vi "Beampointing_Multi_Pico2_test.vi"() -> ()   [LabVIEW 2011]
uses:
  GUI_Template/GUI_master/tcp_new_data_event.ctl
  GUI_Template/GUI_master/tcp new data cluster.ctl
  Ctrs/beam detection.ctl
  GUI_Beampointing_single_TRA/Ctrs/move.ctl
  <vilib>/Utility/file.llb/Read From Spreadsheet File (string).vi
  <userlib>/_OpenG.lib/array/array.llb/Filter 1D Array with Scalar (String)__ogtk.vi
  <userlib>/_OpenG.lib/array/array.llb/Filter 1D Array (String)__ogtk.vi
  <vilib>/Utility/file.llb/Write To Spreadsheet File (string).vi
  <vilib>/Analysis/NI_AALBase.lvlib
panel:
  out "x-y*floor(x/y)":dbl
  out "error out":errorcluster
  out "config path":string
  out "Array 3":bool[](array[boolean])
  out "Array 2":u16[](array[numeric])
  out "Array":u16[](array[numeric])
  out "Moving Y":string
  out "Moving X":string
  out "particles":T1(array[cluster])
  out "millisecond timer value":u32
  out "appended path":path
  out "millisecond timer 2":u32
  in  "GUIdevice 98":string="PicoPad4"
  in  "Position.Axis 111::98":dbl=77.0 caption="Motor Axis 1" min=-20000.0 max=20000.0 format="%#_6f"
  in  "Position.Axis 112::98":dbl=77.0 caption="Motor Axis 1" min=-20000.0 max=20000.0 format="%#_6f"
  in  "Position.Axis 113::98":dbl=77.0 caption="Motor Axis 1" min=-20000.0 max=20000.0 format="%#_6f"
  in  "Position.Axis 121::98":dbl=77.0 caption="Motor Axis 1" min=-999999.0 max=999999.0 format="%#_6f"
  in  "Position.Axis 122::98":dbl=77.0 caption="Motor Axis 1" min=-999999.0 max=999999.0 format="%#_6f"
  in  "Position.Axis 123::98":dbl=77.0 caption="Motor Axis 1" min=-999999.0 max=999999.0 format="%#_6f"
  in  "Position.Axis 131::98":dbl=77.0 caption="Motor Axis 1" min=-999999.0 max=999999.0 format="%#_6f"
  in  "Position.Axis 132::98":dbl=77.0 caption="Motor Axis 1" min=-999999.0 max=999999.0 format="%#_6f"
  in  "Position.Axis 133::98":dbl=77.0 caption="Motor Axis 1" min=-999999.0 max=999999.0 format="%#_6f"
  in  "Position.Axis 141::98":dbl=77.0 caption="Motor Axis 1" min=-999999.0 max=999999.0 format="%#_6f"
  in  "Position.Axis 142::98":dbl=77.0 caption="Motor Axis 1" min=-999999.0 max=999999.0 format="%#_6f"
  in  "Position.Axis 143::98":dbl=77.0 caption="Motor Axis 1" min=-999999.0 max=999999.0 format="%#_6f"
  in  "Position.Axis 211::98":dbl=77.0 caption="Motor Axis 1" min=-999999.0 max=999999.0 format="%#_6f"
  in  "Position.Axis 212::98":dbl=77.0 caption="Motor Axis 1" min=-999999.0 max=999999.0 format="%#_6f"
  in  "Position.Axis 213::98":dbl=77.0 caption="Motor Axis 1" min=-999999.0 max=999999.0 format="%#_6f"
  in  "Position.Axis 221::98":dbl=77.0 caption="Motor Axis 1" min=-999999.0 max=999999.0 format="%#_6f"
  in  "Position.Axis 222::98":dbl=77.0 caption="Motor Axis 1" min=-999999.0 max=999999.0 format="%#_6f"
  in  "Position.Axis 223::98":dbl=77.0 caption="Motor Axis 1" min=-999999.0 max=999999.0 format="%#_6f"
  in  "Position.Axis 231::98":dbl=77.0 caption="Motor Axis 1" min=-999999.0 max=999999.0 format="%#_6f"
  in  "Position.Axis 232::98":dbl=77.0 caption="Motor Axis 1" min=-999999.0 max=999999.0 format="%#_6f"
  in  "Position.Axis 233::98":dbl=77.0 caption="Motor Axis 1" min=-999999.0 max=999999.0 format="%#_6f"
  in  "Position.Axis 241::98":dbl=77.0 caption="Motor Axis 1" min=-999999.0 max=999999.0 format="%#_6f"
  in  "Position.Axis 242::98":dbl=77.0 caption="Motor Axis 1" min=-999999.0 max=999999.0 format="%#_6f"
  in  "Position.Axis 243::98":dbl=77.0 caption="Motor Axis 1" min=-999999.0 max=999999.0 format="%#_6f"
  in  "Position.Axis 311::98":dbl=77.0 caption="Motor Axis 1" min=-999999.0 max=999999.0 format="%#_6f"
  in  "Position.Axis 312::98":dbl=77.0 caption="Motor Axis 1" min=-999999.0 max=999999.0 format="%#_6f"
  in  "Position.Axis 313::98":dbl=77.0 caption="Motor Axis 1" min=-999999.0 max=999999.0 format="%#_6f"
  in  "Position.Axis 321::98":dbl=77.0 caption="Motor Axis 1" min=-999999.0 max=999999.0 format="%#_6f"
  in  "Position.Axis 322::98":dbl=77.0 caption="Motor Axis 1" min=-999999.0 max=999999.0 format="%#_6f"
  in  "Position.Axis 323::98":dbl=77.0 caption="Motor Axis 1" min=-999999.0 max=999999.0 format="%#_6f"
  in  "Position.Axis 331::98":dbl=77.0 caption="Motor Axis 1" min=-999999.0 max=999999.0 format="%#_6f"
  in  "Position.Axis 332::98":dbl=77.0 caption="Motor Axis 1" min=-999999.0 max=999999.0 format="%#_6f"
  in  "Position.Axis 333::98":dbl=77.0 caption="Motor Axis 1" min=-999999.0 max=999999.0 format="%#_6f"
  in  "Position.Axis 341::98":dbl=77.0 caption="Motor Axis 1" min=-999999.0 max=999999.0 format="%#_6f"
  in  "Position.Axis 342::98":dbl=77.0 caption="Motor Axis 1" min=-999999.0 max=999999.0 format="%#_6f"
  in  "Position.Axis 343::98":dbl=77.0 caption="Motor Axis 1" min=-999999.0 max=999999.0 format="%#_6f"
  in  "Position.Axis 411::98":dbl=77.0 caption="Motor Axis 1" min=-999999.0 max=999999.0 format="%#_6f"
  in  "Position.Axis 412::98":dbl=77.0 caption="Motor Axis 1" min=-999999.0 max=999999.0 format="%#_6f"
  in  "Position.Axis 413::98":dbl=77.0 caption="Motor Axis 1" min=-999999.0 max=999999.0 format="%#_6f"
  in  "Position.Axis 421::98":dbl=77.0 caption="Motor Axis 1" min=-999999.0 max=999999.0 format="%#_6f"
  in  "Position.Axis 422::98":dbl=77.0 caption="Motor Axis 1" min=-999999.0 max=999999.0 format="%#_6f"
  in  "Position.Axis 423::98":dbl=77.0 caption="Motor Axis 1" min=-999999.0 max=999999.0 format="%#_6f"
  in  "Position.Axis 431::98":dbl=77.0 caption="Motor Axis 1" min=-999999.0 max=999999.0 format="%#_6f"
  in  "Position.Axis 432::98":dbl=77.0 caption="Motor Axis 1" min=-999999.0 max=999999.0 format="%#_6f"
  in  "Position.Axis 433::98":dbl=77.0 caption="Motor Axis 1" min=-999999.0 max=999999.0 format="%#_6f"
  in  "Position.Axis 441::98":dbl=77.0 caption="Motor Axis 1" min=-999999.0 max=999999.0 format="%#_6f"
  in  "Position.Axis 442::98":dbl=77.0 caption="Motor Axis 1" min=-999999.0 max=999999.0 format="%#_6f"
  in  "Position.Axis 443::98":dbl=77.0 caption="Motor Axis 1" min=-999999.0 max=999999.0 format="%#_6f"
  in  "Position.Axis 511::98":dbl=77.0 caption="Motor Axis 1" min=-999999.0 max=999999.0 format="%#_6f"
  in  "Position.Axis 512::98":dbl=77.0 caption="Motor Axis 1" min=-999999.0 max=999999.0 format="%#_6f"
  in  "Position.Axis 513::98":dbl=77.0 caption="Motor Axis 1" min=-999999.0 max=999999.0 format="%#_6f"
  in  "Position.Axis 521::98":dbl=77.0 caption="Motor Axis 1" min=-999999.0 max=999999.0 format="%#_6f"
  in  "Position.Axis 522::98":dbl=77.0 caption="Motor Axis 1" min=-999999.0 max=999999.0 format="%#_6f"
  in  "Position.Axis 523::98":dbl=77.0 caption="Motor Axis 1" min=-999999.0 max=999999.0 format="%#_6f"
  in  "Position.Axis 531::98":dbl=77.0 caption="Motor Axis 1" min=-999999.0 max=999999.0 format="%#_6f"
  in  "Position.Axis 532::98":dbl=77.0 caption="Motor Axis 1" min=-999999.0 max=999999.0 format="%#_6f"
  in  "Position.Axis 533::98":dbl=77.0 caption="Motor Axis 1" min=-999999.0 max=999999.0 format="%#_6f"
  in  "Position.Axis 541::98":dbl=77.0 caption="Motor Axis 1" min=-999999.0 max=999999.0 format="%#_6f"
  in  "Position.Axis 542::98":dbl=77.0 caption="Motor Axis 1" min=-999999.0 max=999999.0 format="%#_6f"
  in  "Position.Axis 543::98":dbl=77.0 caption="Motor Axis 1" min=-999999.0 max=999999.0 format="%#_6f"
  in  "Numeric":dbl
  out "Current State":string
  in  "output cluster 2":T5 {"detection para"."smal para"."Measurement Parameter" items=["Center of Mass X", "Center of Mass Y", "First Pixel X", "First Pixel Y", "Bounding Rect Left", "Bounding Rect Top", "Bounding Rect Right", "Bounding Rect Bottom", "Max Feret Diameter Start X", "Max Feret Diameter Start Y", "Max Feret Diameter End X", "Max Feret Diameter End Y", "Max Horiz. Segment Length Left", "Max Horiz. Segment Length Right", "Max Horiz. Segment Length Row", "-", "Bounding Rect Width", "Bounding Rect Height", "Bounding Rect Diagonal", "Perimeter", "Convex Hull Perimeter", "Holes' Perimeter", "Max Feret Diameter", "Equivalent Ellipse Major Axis", "Equivalent Ellipse Minor Axis", "Equivalent Ellipse Minor Axis (Feret)", "Equivalent Rect Long Side", "Equivalent Rect Short Side", "Equivalent Rect Diagonal", "Equivalent Rect Short Side (Feret)", "Average Horiz. Segment Length", "Average Vert. Segment Length", "Hydraulic Radius", "Waddel Disk Diameter", "-", "Area", "Holes' Area", "Particle & Holes' Area", "Convex Hull Area", "Image Area", "-", "Number of Holes", "Number of Horiz. Segments", "Number of Vert. Segments", "-", "Orientation", "Max Feret Diameter Orientation", "-", "% Area/Image Area", "% Area/(Particle & Holes' Area)", "Ratio of Equivalent Ellipse Axes", "Ratio of Equivalent Rect Sides", "-", "Elongation Factor", "Compactness Factor", "Heywood Circularity Factor", "Type Factor", "-", "Sum X", "Sum Y", "Sum XX", "Sum XY", "Sum YY", "Sum XXX", "Sum XXY", "Sum XYY", "Sum YYY", "-", "Moment of Inertia XX", "Moment of Inertia XY", "Moment of Inertia YY", "Moment of Inertia XXX", "Moment of Inertia XXY", "Moment of Inertia XYY", "Moment of Inertia YYY", "Norm. Moment of Inertia XX", "Norm. Moment of Inertia XY", "Norm. Moment of Inertia YY", "Norm. Moment of Inertia XXX", "Norm. Moment of Inertia XXY", "Norm. Moment of Inertia XYY", "Norm. Moment of Inertia YYY", "Hu Moment 1", "Hu Moment 2", "Hu Moment 3", "Hu Moment 4", "Hu Moment 5", "Hu Moment 6", "Hu Moment 7"]; "detection para"."smal para"."Range Lower Value" format="%.2f"; "detection para"."smal para"."Range Upper Value" format="%.2f"; "detection para"."detection method" items=["clustering", "entropy", "metric", "moments", "inter-class variance"]; "detection para"."Filter" items=["No Filter", "Median Filter", "Low Pass Filter"]}
  out "CCDs":string[](array[string])
  in  "GUIdevice 12":string
  in  "GUIdevice 11":string
  in  "GUIdevice 10":string
  in  "GUIdevice 9":string
  out "error out 2":errorcluster
  in  "active cams":string[](array[string])
  in  "Motor Y":dbl[][](array[numeric])
  in  "Motor X":dbl[][](array[numeric])
  out "Names":string[](array[string])
  in  "Offset X stats":dbl[][](array[numeric])
  in  "Offset Y stats":dbl[][](array[numeric])
  out "Box":T6(array[cluster])
  in  "Tab Control 2":enum32{"Config ", "Main", "History"}(tab)=enum."Main"
  out "Waveform Chart":u32(graph)
  in  "associated motors":T7
  out "Cameras":T8
  out "Status":cluster{i32, i32, "Centroid X":dbl[][]}(graph)
  in  "Exposure:12":dbl=0.095 min=0.0001 max=1.0 format="%#_6f"
  in  "Triggerdelay::12":dbl=0.003 min=0.0 max=0.09 format="%#_6f"
  in  "Exposure::11":dbl=0.095 min=0.0001 max=1.0 format="%#_6f"
  in  "Triggerdelay::11":dbl=0.003 min=0.0 max=0.09 format="%#_6f"
  in  "Exposure::10":dbl=0.095 min=0.0001 max=1.0 format="%#_6f"
  in  "Triggerdelay::10":dbl=0.003 min=0.0 max=0.09 format="%#_6f"
  in  "Exposure::9":dbl=0.095 min=0.0001 max=1.0 format="%#_6f"
  in  "Triggerdelay::9":dbl=0.003 min=0.0 max=0.09 format="%#_6f"
  in  "Trigger::9":bool
  in  "Trigger::10":bool caption="Trigger:10"
  in  "Trigger::11":bool
  in  "Trigger::12":bool
  in  "Target.Y::9":dbl=45.0 caption="T9y" min=0.0 max=2000.0 format="%#_6f"
  in  "Target.X::9":dbl=47.0 caption="Tx9" min=0.0 max=2000.0 format="%#_6f"
  in  "Target.Y::10":dbl=45.0 caption="T10y" min=0.0 max=2000.0 format="%#_6f"
  in  "Target.X::10":dbl=47.0 caption="T10x" min=0.0 max=2000.0 format="%#_6f"
  in  "Target.Y::11":dbl=45.0 caption="T11y" min=0.0 max=2000.0 format="%#_6f"
  in  "Target.X::11":dbl=47.0 caption="T11x" min=0.0 max=2000.0 format="%#_6f"
  in  "Target.Y::12":dbl=45.0 caption="T12y" min=0.0 max=2000.0 format="%#_6f"
  in  "Target.X::12":dbl=47.0 caption="T12x" min=0.0 max=2000.0 format="%#_6f"
  in  "Exposure::8":dbl=0.095 min=0.01 max=1.0 format="%#_6f"
  in  "Triggerdelay::8":dbl=0.003 min=0.0 max=0.09 format="%#_6f"
  in  "Trigger::8":bool
  in  "Target.Y::8":dbl=45.0 caption="T8y" min=0.0 max=2000.0 format="%#_6f"
  in  "Target.X::8":dbl=47.0 caption="T8x" min=0.0 max=2000.0 format="%#_6f"
  in  "Target.Y::7":dbl=45.0 caption="T7x" min=0.0 max=2000.0 format="%#_6f"
  in  "Target.X::7":dbl=47.0 caption="T7y" min=0.0 max=2000.0 format="%#_6f"
  in  "Target.Y::6":dbl=45.0 caption="T6y" min=0.0 max=2000.0 format="%#_6f"
  in  "Target.X::6":dbl=47.0 caption="T6x" min=0.0 max=2000.0 format="%#_6f"
  in  "Target.Y::5":dbl=45.0 caption="T5y" min=0.0 max=2000.0 format="%#_6f"
  in  "Target.X::5":dbl=47.0 caption="T5x" min=0.0 max=2000.0 format="%#_6f"
  in  "Target.Y::4":dbl=45.0 caption="T4y" min=0.0 max=2000.0 format="%#_6f"
  in  "Target.X::4":dbl=47.0 caption="T4x" min=0.0 max=2000.0 format="%#_6f"
  in  "Target.Y::3":dbl=163.0 caption="T3y" min=0.0 max=2000.0 format="%#_6f"
  in  "Target.X::3":dbl=152.0 caption="T3x" min=0.0 max=2000.0 format="%#_6f"
  in  "Target.Y::2":dbl=74.0 caption="T2y" min=1.0 max=600.0 format="%#_6f"
  in  "Target.X::2":dbl=75.0 caption="T2x" min=1.0 max=800.0 format="%#_6f"
  in  "Target.Y::1":dbl=61.0 caption="T1y" min=1.0 max=600.0 format="%#_6f"
  in  "Target.X::1":dbl=77.0 caption="T1x" min=1.0 max=800.0 format="%#_6f"
  in  "Exposure::7":dbl=0.095 min=0.0001 max=1.0 format="%#_6f"
  in  "Triggerdelay::7":dbl=0.003 min=0.0 max=0.09 format="%#_6f"
  in  "Trigger::7":bool
  in  "Exposure::6":dbl=0.095 min=0.0001 max=1.0 format="%#_6f"
  in  "Triggerdelay::6":dbl=0.003 min=0.0 max=0.09 format="%#_6f"
  in  "Trigger::6":bool
  in  "Exposure::5":dbl=0.095 min=0.0001 max=1.0 format="%#_6f"
  in  "Triggerdelay::5":dbl=0.003 min=0.0 max=0.09 format="%#_6f"
  in  "Trigger::5":bool
  in  "Exposure::4":dbl=0.095 min=0.0001 max=1.0 format="%#_6f"
  in  "Triggerdelay::4":dbl=0.003 min=0.0 max=0.09 format="%#_6f"
  in  "Trigger::4":bool
  in  "Exposure::3":dbl=0.095 min=0.0001 max=1.0 format="%#_6f"
  in  "Triggerdelay::3":dbl=0.003 min=0.0 max=0.09 format="%#_6f"
  in  "Trigger::3":bool
  in  "Exposure::2":dbl=0.095 min=0.0001 max=1.0 format="%#_6f"
  in  "Triggerdelay::2":dbl=0.003 min=0.0 max=0.09 format="%#_6f"
  in  "Trigger::2":bool
  out "image::1":T9(plugin-control) caption="PA2_Input1"
  out "image::2":T9(plugin-control) caption="PA2_Input2"
  out "image::3":T9(plugin-control) caption="L1_TelInpNear"
  out "image::4":T9(plugin-control) caption="L2_TelInpFar"
  out "image::5":T9(plugin-control) caption="L4_TREXpass1"
  out "image::6":T9(plugin-control) caption="L5_TREXPass2"
  out "image::7":T9(plugin-control) caption="L6_TREXpass3"
  out "image::8":T9(plugin-control) caption="L7_TREXPass4"
  in  "Exposure::1":dbl=0.095 min=0.0001 max=1.0 format="%#_6f"
  in  "Triggerdelay::1":dbl=0.003 min=0.0 max=0.09 format="%#_6f"
  in  "Trigger::1":bool
  in  "UDP error message":string
  out "required Y":bool[](array[boolean])
  out "required X":bool[](array[boolean])
  out "detected":bool[](array[boolean])
  out "name array":string[](array[string])
  out "image::9":T9(plugin-control) caption="L8_M10Leak"
  out "image::10":T9(plugin-control) caption="B1_TelInput"
  out "image::11":T9(plugin-control) caption="B2_TelLens1"
  out "image::12":T9(plugin-control) caption="B5_CompressorOut"
  out "speedmode X":bool[](array[boolean])
  out "speedmode Y":bool[](array[boolean])
  out "CCD 9":cluster{timestamp[], dbl[]}[](graph)
  out "CCD 10":cluster{timestamp[], dbl[]}[](graph)
  out "CCD 11":cluster{timestamp[], dbl[]}[](graph)
  out "CCD 12":cluster{timestamp[], dbl[]}[](graph)
  out "CCD 5":cluster{timestamp[], dbl[]}[](graph)
  out "CCD 6":cluster{timestamp[], dbl[]}[](graph)
  out "CCD 7":cluster{timestamp[], dbl[]}[](graph)
  out "CCD 8":cluster{timestamp[], dbl[]}[](graph)
  out "CCD 2":cluster{timestamp[], dbl[]}[](graph)
  out "CCD 1":cluster{timestamp[], dbl[]}[](graph)
  out "CCD 3":cluster{timestamp[], dbl[]}[](graph)
  out "CCD 4":cluster{timestamp[], dbl[]}[](graph)
  out "History index":i32
  in  "History Size":i32=500
  out "Particle Reports (Pixels)":T10(array[cluster])
  in  "Feedback Global":bool
  in  "detection para":T3[](array[typedef])=[{"Filter"=1, "Filter Para"={"X Size"=5, "Y Size"=5, "% Tolerance"=1}, "detection method"=4, "smal para"=[{"Measurement Parameter"=35, "Range Lower Value"=0.0, "Range Upper Value"=0.0, "Range"=TRUE, "Measurement Type"=FALSE}], "Remove small Objects"=TRUE, "Restrict to round Objects"=FALSE}, {"Filter"=1, "Filter Para"={"X Size"=5, "Y Size"=5, "% Tolerance"=1}, "detection method"=4, "smal para"=[{"Measurement Parameter"=35, "Range Lower Value"=0.0, "Range Upper Value"=500.0, "Range"=FALSE, "Measurement Type"=FALSE}], "Remove small Objects"=TRUE, "Restrict to round Objects"=FALSE}, {"Filter"=1, "Filter Para"={"X Size"=5, "Y Size"=5, "% Tolerance"=1}, "detection method"=4, "smal para"=[{"Measurement Parameter"=35, "Range Lower Value"=0.0, "Range Upper Value"=500.0, "Range"=TRUE, "Measurement Type"=FALSE}], "Remove small Objects"=TRUE, "Restrict to round Objects"=FALSE}, {"Filter"=1, "Filter Para"={"X Size"=5, "Y Size"=5, "% Tolerance"=1}, "detection method"=4, "smal para"=[{"Measurement Parameter"=35, "Range Lower Value"=0.0, "Range Upper Value"=500.0, "Range"=TRUE, "Measurement Type"=FALSE}], "Remove small Objects"=TRUE, "Restrict to round Objects"=FALSE}, {"Filter"=1, "Filter Para"={"X Size"=5, "Y Size"=5, "% Tolerance"=1}, "detection method"=4, "smal para"=[{"Measurement Parameter"=35, "Range Lower Value"=0.0, "Range Upper Value"=500.0, "Range"=TRUE, "Measurement Type"=FALSE}], "Remove small Objects"=TRUE, "Restrict to round Objects"=FALSE}, {"Filter"=1, "Filter Para"={"X Size"=5, "Y Size"=5, "% Tolerance"=1}, "detection method"=4, "smal para"=[{"Measurement Parameter"=35, "Range Lower Value"=0.0, "Range Upper Value"=500.0, "Range"=TRUE, "Measurement Type"=FALSE}], "Remove small Objects"=TRUE, "Restrict to round Objects"=FALSE}, {"Filter"=1, "Filter Para"={"X Size"=5, "Y Size"=5, "% Tolerance"=1}, "detection method"=4, "smal para"=[{"Measurement Parameter"=35, "Range Lower Value"=0.0, "Range Upper Value"=500.0, "Range"=TRUE, "Measurement Type"=FALSE}], "Remove small Objects"=TRUE, "Restrict to round Objects"=FALSE}, {"Filter"=1, "Filter Para"={"X Size"=5, "Y Size"=5, "% Tolerance"=1}, "detection method"=3, "smal para"=[{"Measurement Parameter"=35, "Range Lower Value"=0.0, "Range Upper Value"=0.0, "Range"=FALSE, "Measurement Type"=FALSE}], "Remove small Objects"=TRUE, "Restrict to round Objects"=FALSE}, {"Filter"=1, "Filter Para"={"X Size"=5, "Y Size"=5, "% Tolerance"=1}, "detection method"=4, "smal para"=[{"Measurement Parameter"=35, "Range Lower Value"=0.0, "Range Upper Value"=0.0, "Range"=FALSE, "Measurement Type"=FALSE}], "Remove small Objects"=TRUE, "Restrict to round Objects"=FALSE}, {"Filter"=1, "Filter Para"={"X Size"=5, "Y Size"=5, "% Tolerance"=1}, "detection method"=4, "smal para"=[{"Measurement Parameter"=35, "Range Lower Value"=0.0, "Range Upper Value"=500.0, "Range"=TRUE, "Measurement Type"=FALSE}], "Remove small Objects"=TRUE, "Restrict to round Objects"=FALSE}, {"Filter"=1, "Filter Para"={"X Size"=5, "Y Size"=5, "% Tolerance"=1}, "detection method"=4, "smal para"=[{"Measurement Parameter"=35, "Range Lower Value"=0.0, "Range Upper Value"=500.0, "Range"=TRUE, "Measurement Type"=FALSE}], "Remove small Objects"=TRUE, "Restrict to round Objects"=FALSE}, {"Filter"=1, "Filter Para"={"X Size"=5, "Y Size"=5, "% Tolerance"=1}, "detection method"=4, "smal para"=[{"Measurement Parameter"=35, "Range Lower Value"=0.0, "Range Upper Value"=500.0, "Range"=TRUE, "Measurement Type"=FALSE}], "Remove small Objects"=TRUE, "Restrict to round Objects"=FALSE}] {"smal para"."Measurement Parameter" items=["Center of Mass X", "Center of Mass Y", "First Pixel X", "First Pixel Y", "Bounding Rect Left", "Bounding Rect Top", "Bounding Rect Right", "Bounding Rect Bottom", "Max Feret Diameter Start X", "Max Feret Diameter Start Y", "Max Feret Diameter End X", "Max Feret Diameter End Y", "Max Horiz. Segment Length Left", "Max Horiz. Segment Length Right", "Max Horiz. Segment Length Row", "-", "Bounding Rect Width", "Bounding Rect Height", "Bounding Rect Diagonal", "Perimeter", "Convex Hull Perimeter", "Holes' Perimeter", "Max Feret Diameter", "Equivalent Ellipse Major Axis", "Equivalent Ellipse Minor Axis", "Equivalent Ellipse Minor Axis (Feret)", "Equivalent Rect Long Side", "Equivalent Rect Short Side", "Equivalent Rect Diagonal", "Equivalent Rect Short Side (Feret)", "Average Horiz. Segment Length", "Average Vert. Segment Length", "Hydraulic Radius", "Waddel Disk Diameter", "-", "Area", "Holes' Area", "Particle & Holes' Area", "Convex Hull Area", "Image Area", "-", "Number of Holes", "Number of Horiz. Segments", "Number of Vert. Segments", "-", "Orientation", "Max Feret Diameter Orientation", "-", "% Area/Image Area", "% Area/(Particle & Holes' Area)", "Ratio of Equivalent Ellipse Axes", "Ratio of Equivalent Rect Sides", "-", "Elongation Factor", "Compactness Factor", "Heywood Circularity Factor", "Type Factor", "-", "Sum X", "Sum Y", "Sum XX", "Sum XY", "Sum YY", "Sum XXX", "Sum XXY", "Sum XYY", "Sum YYY", "-", "Moment of Inertia XX", "Moment of Inertia XY", "Moment of Inertia YY", "Moment of Inertia XXX", "Moment of Inertia XXY", "Moment of Inertia XYY", "Moment of Inertia YYY", "Norm. Moment of Inertia XX", "Norm. Moment of Inertia XY", "Norm. Moment of Inertia YY", "Norm. Moment of Inertia XXX", "Norm. Moment of Inertia XXY", "Norm. Moment of Inertia XYY", "Norm. Moment of Inertia YYY", "Hu Moment 1", "Hu Moment 2", "Hu Moment 3", "Hu Moment 4", "Hu Moment 5", "Hu Moment 6", "Hu Moment 7"]; "smal para"."Range Lower Value" format="%.2f"; "smal para"."Range Upper Value" format="%.2f"; "detection method" items=["clustering", "entropy", "metric", "moments", "inter-class variance"]; "Filter" items=["No Filter", "Median Filter", "Low Pass Filter"]}
  in  "GUIdevice 8":string="B5_CompressorOut"
  in  "Tab Control":T11(tab)
  in  "Center":bool
  in  "Save Stats":bool
  in  "Save Config":bool
  in  "Load Config":bool
  in  "update speed [ms]":i32=200
  in  "Img to avg":i32=20
  in  "Reset History":bool
  in  "save path":path=path "W:/BP_DATA"
  in  "autodetect":bool
  in  "Detection Rate":dbl=0.8 min=0.001 max=1.0
  in  "new tdms":bool
  in  "Speedmode @":dbl=3.0 min=1.0 max=20.0
  in  "Align":bool
  in  "deivice ini":bool
  in  "beam detection para":T3={"Filter"=1, "Filter Para"={"X Size"=5, "Y Size"=5, "% Tolerance"=1}, "detection method"=4, "smal para"=[{"Measurement Parameter"=35, "Range Lower Value"=0.0, "Range Upper Value"=500.0, "Range"=FALSE, "Measurement Type"=FALSE}], "Remove small Objects"=TRUE, "Restrict to round Objects"=FALSE} {"smal para"."Measurement Parameter" items=["Center of Mass X", "Center of Mass Y", "First Pixel X", "First Pixel Y", "Bounding Rect Left", "Bounding Rect Top", "Bounding Rect Right", "Bounding Rect Bottom", "Max Feret Diameter Start X", "Max Feret Diameter Start Y", "Max Feret Diameter End X", "Max Feret Diameter End Y", "Max Horiz. Segment Length Left", "Max Horiz. Segment Length Right", "Max Horiz. Segment Length Row", "-", "Bounding Rect Width", "Bounding Rect Height", "Bounding Rect Diagonal", "Perimeter", "Convex Hull Perimeter", "Holes' Perimeter", "Max Feret Diameter", "Equivalent Ellipse Major Axis", "Equivalent Ellipse Minor Axis", "Equivalent Ellipse Minor Axis (Feret)", "Equivalent Rect Long Side", "Equivalent Rect Short Side", "Equivalent Rect Diagonal", "Equivalent Rect Short Side (Feret)", "Average Horiz. Segment Length", "Average Vert. Segment Length", "Hydraulic Radius", "Waddel Disk Diameter", "-", "Area", "Holes' Area", "Particle & Holes' Area", "Convex Hull Area", "Image Area", "-", "Number of Holes", "Number of Horiz. Segments", "Number of Vert. Segments", "-", "Orientation", "Max Feret Diameter Orientation", "-", "% Area/Image Area", "% Area/(Particle & Holes' Area)", "Ratio of Equivalent Ellipse Axes", "Ratio of Equivalent Rect Sides", "-", "Elongation Factor", "Compactness Factor", "Heywood Circularity Factor", "Type Factor", "-", "Sum X", "Sum Y", "Sum XX", "Sum XY", "Sum YY", "Sum XXX", "Sum XXY", "Sum XYY", "Sum YYY", "-", "Moment of Inertia XX", "Moment of Inertia XY", "Moment of Inertia YY", "Moment of Inertia XXX", "Moment of Inertia XXY", "Moment of Inertia XYY", "Moment of Inertia YYY", "Norm. Moment of Inertia XX", "Norm. Moment of Inertia XY", "Norm. Moment of Inertia YY", "Norm. Moment of Inertia XXX", "Norm. Moment of Inertia XXY", "Norm. Moment of Inertia XYY", "Norm. Moment of Inertia YYY", "Hu Moment 1", "Hu Moment 2", "Hu Moment 3", "Hu Moment 4", "Hu Moment 5", "Hu Moment 6", "Hu Moment 7"]; "smal para"."Range Lower Value" format="%.2f"; "smal para"."Range Upper Value" format="%.2f"; "detection method" items=["clustering", "entropy", "metric", "moments", "inter-class variance"]; "Filter" items=["No Filter", "Median Filter", "Low Pass Filter"]}
  in  "move config":T2={"Tolerance [%]"=0.1, "Stepsize"=0.0001, "Invert Axis"=TRUE, "Invert Direction X"=FALSE, "Invert Direction Y"=TRUE, "enable feedback"=FALSE, "Set Centriod Target"=FALSE}
  in  "ActiveMotor":u16(ring)=7 items=["PA2_Input1", "PA2_Input2", "L2_TelInpFar", "L1_TelInpNear", "L4_TREXPASS1", "L5_TREXPass2", "L6_TREXPass3", "L7_TREXPass4", "L8_M10Leak", "B1_TelInput", "B2_TelLens1", "NoName", "NoName", "NoName", "MBeamSplitterL", "Mdiode", "NoName", "NoName", "NoName", "NoName"]
  in  "ActiveMotorName::99":string
  in  "RelativeMove.Axis 1.CCW::99":bool caption="RelativeMove.Axis 1.CCW::1"
  in  "RelativeMove.Axis 1.CW::99":bool caption="RelativeMove.Axis 1.CW::1"
  in  "RelativeMove.Axis 2.CCW::99":bool caption="RelativeMove.Axis. 2.CCW::1"
  in  "RelativeMove.Axis 2.CW::99":bool caption="RelativeMove.Axis 2.CW::1"
  in  "RelativeSettings.Axis 1.Position::99":dbl caption="Axis 1 Position" min=-999999.0 max=999999.0 format="%_4p"
  in  "RelativeSettings.Axis 2.Position::99":dbl caption="Axis 2 Position" min=-999999.0 max=999999.0 format="%_4p"
  in  "RelativeSettings.Axis 2.StepSize::99":dbl=50.0 caption="Axis 2 StepSize" min=0.0 max=999999.0 format="%_4p"
  in  "RelativeSettings.Axis 1.StepSize::99":dbl=50.0 caption="Axis 1 Stepsize" min=0.0 max=999999.0 format="%_4p"
  out "Arguments Y":string
  in  "active axis refs 2":T12(array[cluster])
  in  "active Axis ref":cluster{"Ref X":refnum<vi>, "Ref Y":refnum<vi>}
  in  "CCDs":u16(ring) items=["PA2_Input1", "PA2_Input2", "L1_TelInpNear", "L2_TelInpFar", "L4_TREXpass1", "L5_TREXPass2", "L6_TREXpass3", "L7_TREXPass4", "L8_M10Leak", "B1_TelInput", "B2_TelLens1", "B5_CompressorOut"]
  out "motor refs":refnum<vi>[](array[refnum])
  in  "Position.Axis 511::99":dbl=77.0 caption="Motor Axis 1" min=-20000.0 max=20000.0 format="%#_6f"
  in  "Position.Axis 512::99":dbl=77.0 caption="Motor Axis 1" min=-20000.0 max=20000.0 format="%#_6f"
  in  "Position.Axis 513::99":dbl=77.0 caption="Motor Axis 1" min=-20000.0 max=20000.0 format="%#_6f"
  in  "Position.Axis 521::99":dbl=77.0 caption="Motor Axis 1" min=-20000.0 max=20000.0 format="%#_6f"
  in  "Position.Axis 522::99":dbl=77.0 caption="Motor Axis 1" min=-20000.0 max=20000.0 format="%#_6f"
  in  "Position.Axis 523::99":dbl=77.0 caption="Motor Axis 1" min=-20000.0 max=20000.0 format="%#_6f"
  in  "Position.Axis 531::99":dbl=77.0 caption="Motor Axis 1" min=-20000.0 max=20000.0 format="%#_6f"
  in  "Position.Axis 532::99":dbl=77.0 caption="Motor Axis 1" min=-20000.0 max=20000.0 format="%#_6f"
  in  "Position.Axis 533::99":dbl=77.0 caption="Motor Axis 1" min=-20000.0 max=20000.0 format="%#_6f"
  in  "Position.Axis 541::99":dbl=77.0 caption="Motor Axis 1" min=-20000.0 max=20000.0 format="%#_6f"
  in  "Position.Axis 542::99":dbl=77.0 caption="Motor Axis 1" min=-20000.0 max=20000.0 format="%#_6f"
  in  "Position.Axis 543::99":dbl=77.0 caption="Motor Axis 1" min=-20000.0 max=20000.0 format="%#_6f"
  in  "Position.Axis 411::99":dbl=77.0 caption="Motor Axis 1" min=-20000.0 max=20000.0 format="%#_6f"
  in  "Position.Axis 412::99":dbl=77.0 caption="Motor Axis 1" min=-20000.0 max=20000.0 format="%#_6f"
  in  "Position.Axis 413::99":dbl=77.0 caption="Motor Axis 1" min=-20000.0 max=20000.0 format="%#_6f"
  in  "Position.Axis 421::99":dbl=77.0 caption="Motor Axis 1" min=-20000.0 max=20000.0 format="%#_6f"
  in  "Position.Axis 422::99":dbl=77.0 caption="Motor Axis 1" min=-20000.0 max=20000.0 format="%#_6f"
  in  "Position.Axis 423::99":dbl=77.0 caption="Motor Axis 1" min=-20000.0 max=20000.0 format="%#_6f"
  in  "Position.Axis 431::99":dbl=77.0 caption="Motor Axis 1" min=-20000.0 max=20000.0 format="%#_6f"
  in  "Position.Axis 432::99":dbl=77.0 caption="Motor Axis 1" min=-20000.0 max=20000.0 format="%#_6f"
  in  "Position.Axis 433::99":dbl=77.0 caption="Motor Axis 1" min=-20000.0 max=20000.0 format="%#_6f"
  in  "Position.Axis 441::99":dbl=77.0 caption="Motor Axis 1" min=-20000.0 max=20000.0 format="%#_6f"
  in  "Position.Axis 442::99":dbl=77.0 caption="Motor Axis 1" min=-20000.0 max=20000.0 format="%#_6f"
  in  "Position.Axis 443::99":dbl=77.0 caption="Motor Axis 1" min=-20000.0 max=20000.0 format="%#_6f"
  in  "Position.Axis 311::99":dbl=77.0 caption="Motor Axis 1" min=-200000.0 max=200000.0 format="%#_6f"
  in  "Position.Axis 312::99":dbl=77.0 caption="Motor Axis 1" min=-200000.0 max=200000.0 format="%#_6f"
  in  "Position.Axis 313::99":dbl=77.0 caption="Motor Axis 1" min=-999999.0 max=999999.0 format="%#_6f"
  in  "Position.Axis 321::99":dbl=77.0 caption="Motor Axis 1" min=-20000.0 max=20000.0 format="%#_6f"
  in  "Position.Axis 322::99":dbl=77.0 caption="Motor Axis 1" min=-20000.0 max=20000.0 format="%#_6f"
  in  "Position.Axis 323::99":dbl=77.0 caption="Motor Axis 1" min=-20000.0 max=20000.0 format="%#_6f"
  in  "Position.Axis 331::99":dbl=77.0 caption="Motor Axis 1" min=-20000.0 max=20000.0 format="%#_6f"
  in  "Position.Axis 332::99":dbl=77.0 caption="Motor Axis 1" min=-20000.0 max=20000.0 format="%#_6f"
  in  "Position.Axis 333::99":dbl=77.0 caption="Motor Axis 1" min=-20000.0 max=20000.0 format="%#_6f"
  in  "Position.Axis 341::99":dbl=77.0 caption="Motor Axis 1" min=-20000.0 max=20000.0 format="%#_6f"
  in  "Position.Axis 342::99":dbl=77.0 caption="Motor Axis 1" min=-20000.0 max=20000.0 format="%#_6f"
  in  "Position.Axis 343::99":dbl=77.0 caption="Motor Axis 1" min=-20000.0 max=20000.0 format="%#_6f"
  in  "Position.Axis 241::99":dbl=77.0 caption="Motor Axis 1" min=-20000.0 max=20000.0 format="%#_6f"
  in  "Position.Axis 242::99":dbl=77.0 caption="Motor Axis 1" min=-20000.0 max=20000.0 format="%#_6f"
  in  "Position.Axis 243::99":dbl=77.0 caption="Motor Axis 1" min=-20000.0 max=20000.0 format="%#_6f"
  in  "Position.Axis 231::99":dbl=77.0 caption="Motor Axis 1" min=-20000.0 max=20000.0 format="%#_6f"
  in  "Position.Axis 232::99":dbl=77.0 caption="Motor Axis 1" min=-20000.0 max=20000.0 format="%#_6f"
  in  "Position.Axis 233::99":dbl=77.0 caption="Motor Axis 1" min=-20000.0 max=20000.0 format="%#_6f"
  in  "Position.Axis 221::99":dbl=77.0 caption="Motor Axis 1" min=-20000.0 max=20000.0 format="%#_6f"
  in  "Position.Axis 222::99":dbl=77.0 caption="Motor Axis 1" min=-20000.0 max=200000.0 format="%#_6f"
  in  "Position.Axis 223::99":dbl=77.0 caption="Motor Axis 1" min=-20000.0 max=20000.0 format="%#_6f"
  in  "Position.Axis 211::99":dbl=77.0 caption="Motor Axis 1" min=-20000.0 max=200000.0 format="%#_6f"
  in  "Position.Axis 212::99":dbl=77.0 caption="Motor Axis 1" min=-20000.0 max=20000.0 format="%#_6f"
  in  "Position.Axis 213::99":dbl=77.0 caption="Motor Axis 1" min=-20000.0 max=20000.0 format="%#_6f"
  in  "Position.Axis 141::99":dbl=77.0 caption="Motor Axis 1" min=-20000.0 max=20000.0 format="%#_6f"
  in  "Position.Axis 142::99":dbl=77.0 caption="Motor Axis 1" min=-20000.0 max=20000.0 format="%#_6f"
  in  "Position.Axis 143::99":dbl=77.0 caption="Motor Axis 1" min=-20000.0 max=20000.0 format="%#_6f"
  in  "Position.Axis 131::99":dbl=77.0 caption="Motor Axis 1" min=-20000.0 max=20000.0 format="%#_6f"
  in  "Position.Axis 132::99":dbl=77.0 caption="Motor Axis 1" min=-20000.0 max=20000.0 format="%#_6f"
  in  "Position.Axis 133::99":dbl=77.0 caption="Motor Axis 1" min=-20000.0 max=20000.0 format="%#_6f"
  in  "Position.Axis 121::99":dbl=77.0 caption="Motor Axis 1" min=-20000.0 max=20000.0 format="%#_6f"
  in  "Position.Axis 122::99":dbl=77.0 caption="Motor Axis 1" min=-20000.0 max=20000.0 format="%#_6f"
  in  "Position.Axis 123::99":dbl=77.0 caption="Motor Axis 1" min=-20000.0 max=20000.0 format="%#_6f"
  in  "Position.Axis 113::99":dbl=77.0 caption="Motor Axis 1" min=-20000.0 max=20000.0 format="%#_6f"
  in  "Position.Axis 112::99":dbl=77.0 caption="Motor Axis 1" min=-20000.0 max=20000.0 format="%#_6f"
  in  "Position.Axis 111::99":dbl=77.0 caption="Motor Axis 1" min=-20000.0 max=20000.0 format="%#_6f"
  out "Arguments X":string
  in  "GUIdevice 99":string="PicoPad3"
  in  "move properties":T2[](array[typedef])=[{"Tolerance [%]"=0.1, "Stepsize"=0.0001, "Invert Axis"=TRUE, "Invert Direction X"=FALSE, "Invert Direction Y"=TRUE, "enable feedback"=FALSE, "Set Centriod Target"=FALSE}, {"Tolerance [%]"=0.1, "Stepsize"=0.0001, "Invert Axis"=TRUE, "Invert Direction X"=FALSE, "Invert Direction Y"=TRUE, "enable feedback"=FALSE, "Set Centriod Target"=FALSE}, {"Tolerance [%]"=0.1, "Stepsize"=0.0001, "Invert Axis"=TRUE, "Invert Direction X"=FALSE, "Invert Direction Y"=TRUE, "enable feedback"=FALSE, "Set Centriod Target"=FALSE}, {"Tolerance [%]"=0.1, "Stepsize"=0.0001, "Invert Axis"=TRUE, "Invert Direction X"=FALSE, "Invert Direction Y"=TRUE, "enable feedback"=FALSE, "Set Centriod Target"=FALSE}, {"Tolerance [%]"=0.1, "Stepsize"=0.0001, "Invert Axis"=TRUE, "Invert Direction X"=FALSE, "Invert Direction Y"=TRUE, "enable feedback"=FALSE, "Set Centriod Target"=FALSE}, {"Tolerance [%]"=0.1, "Stepsize"=0.0001, "Invert Axis"=TRUE, "Invert Direction X"=FALSE, "Invert Direction Y"=TRUE, "enable feedback"=FALSE, "Set Centriod Target"=FALSE}, {"Tolerance [%]"=0.1, "Stepsize"=0.0001, "Invert Axis"=TRUE, "Invert Direction X"=FALSE, "Invert Direction Y"=TRUE, "enable feedback"=FALSE, "Set Centriod Target"=FALSE}, {"Tolerance [%]"=0.1, "Stepsize"=0.0001, "Invert Axis"=TRUE, "Invert Direction X"=FALSE, "Invert Direction Y"=TRUE, "enable feedback"=FALSE, "Set Centriod Target"=FALSE}, {"Tolerance [%]"=0.1, "Stepsize"=0.0001, "Invert Axis"=TRUE, "Invert Direction X"=FALSE, "Invert Direction Y"=TRUE, "enable feedback"=FALSE, "Set Centriod Target"=FALSE}, {"Tolerance [%]"=0.1, "Stepsize"=0.0001, "Invert Axis"=TRUE, "Invert Direction X"=FALSE, "Invert Direction Y"=TRUE, "enable feedback"=FALSE, "Set Centriod Target"=FALSE}, {"Tolerance [%]"=0.1, "Stepsize"=0.0001, "Invert Axis"=TRUE, "Invert Direction X"=FALSE, "Invert Direction Y"=TRUE, "enable feedback"=FALSE, "Set Centriod Target"=FALSE}, {"Tolerance [%]"=0.1, "Stepsize"=0.0001, "Invert Axis"=TRUE, "Invert Direction X"=FALSE, "Invert Direction Y"=TRUE, "enable feedback"=FALSE, "Set Centriod Target"=FALSE}, {"Tolerance [%]"=0.1, "Stepsize"=0.0001, "Invert Axis"=TRUE, "Invert Direction X"=FALSE, "Invert Direction Y"=TRUE, "enable feedback"=FALSE, "Set Centriod Target"=FALSE}]
  in  "Time":timestamp[][](array[timestamp])
  in  "Mean Size":dbl[][](array[numeric])
  in  "Size":dbl[][](array[numeric])
  in  "active CCDs":i32(listbox)=1
  in  "Offset Y":dbl[][](array[numeric])
  in  "Offset X":dbl[][](array[numeric])
  in  "Mean Centroid X":dbl[][](array[numeric])
  in  "Mean Centroid Y":dbl[][](array[numeric])
  in  "Centroid Y":dbl[][](array[numeric])
  in  "Centroid X":dbl[][](array[numeric])
  in  "GUIdevice 7":string="B2_TelLens1"
  in  "GUIdevice 6":string="B1_TelInput"
  in  "GUIdevice 5":string="L8_M10Leak"
  in  "GUIdevice 4":string="L7_TREXPass4"
  in  "GUIdevice 3":string="L6_TREXpass3"
  in  "GUIdevice 2":string="L5_TREXPass2"
  in  "insert tag":bool=TRUE
  in  "stop":bool
  in  "GUIdevice 1":string="L4_TREXpass1"
  out "tcp data event":T13
  out "error IO 2":errorcluster
  # "x [Tolerance]"
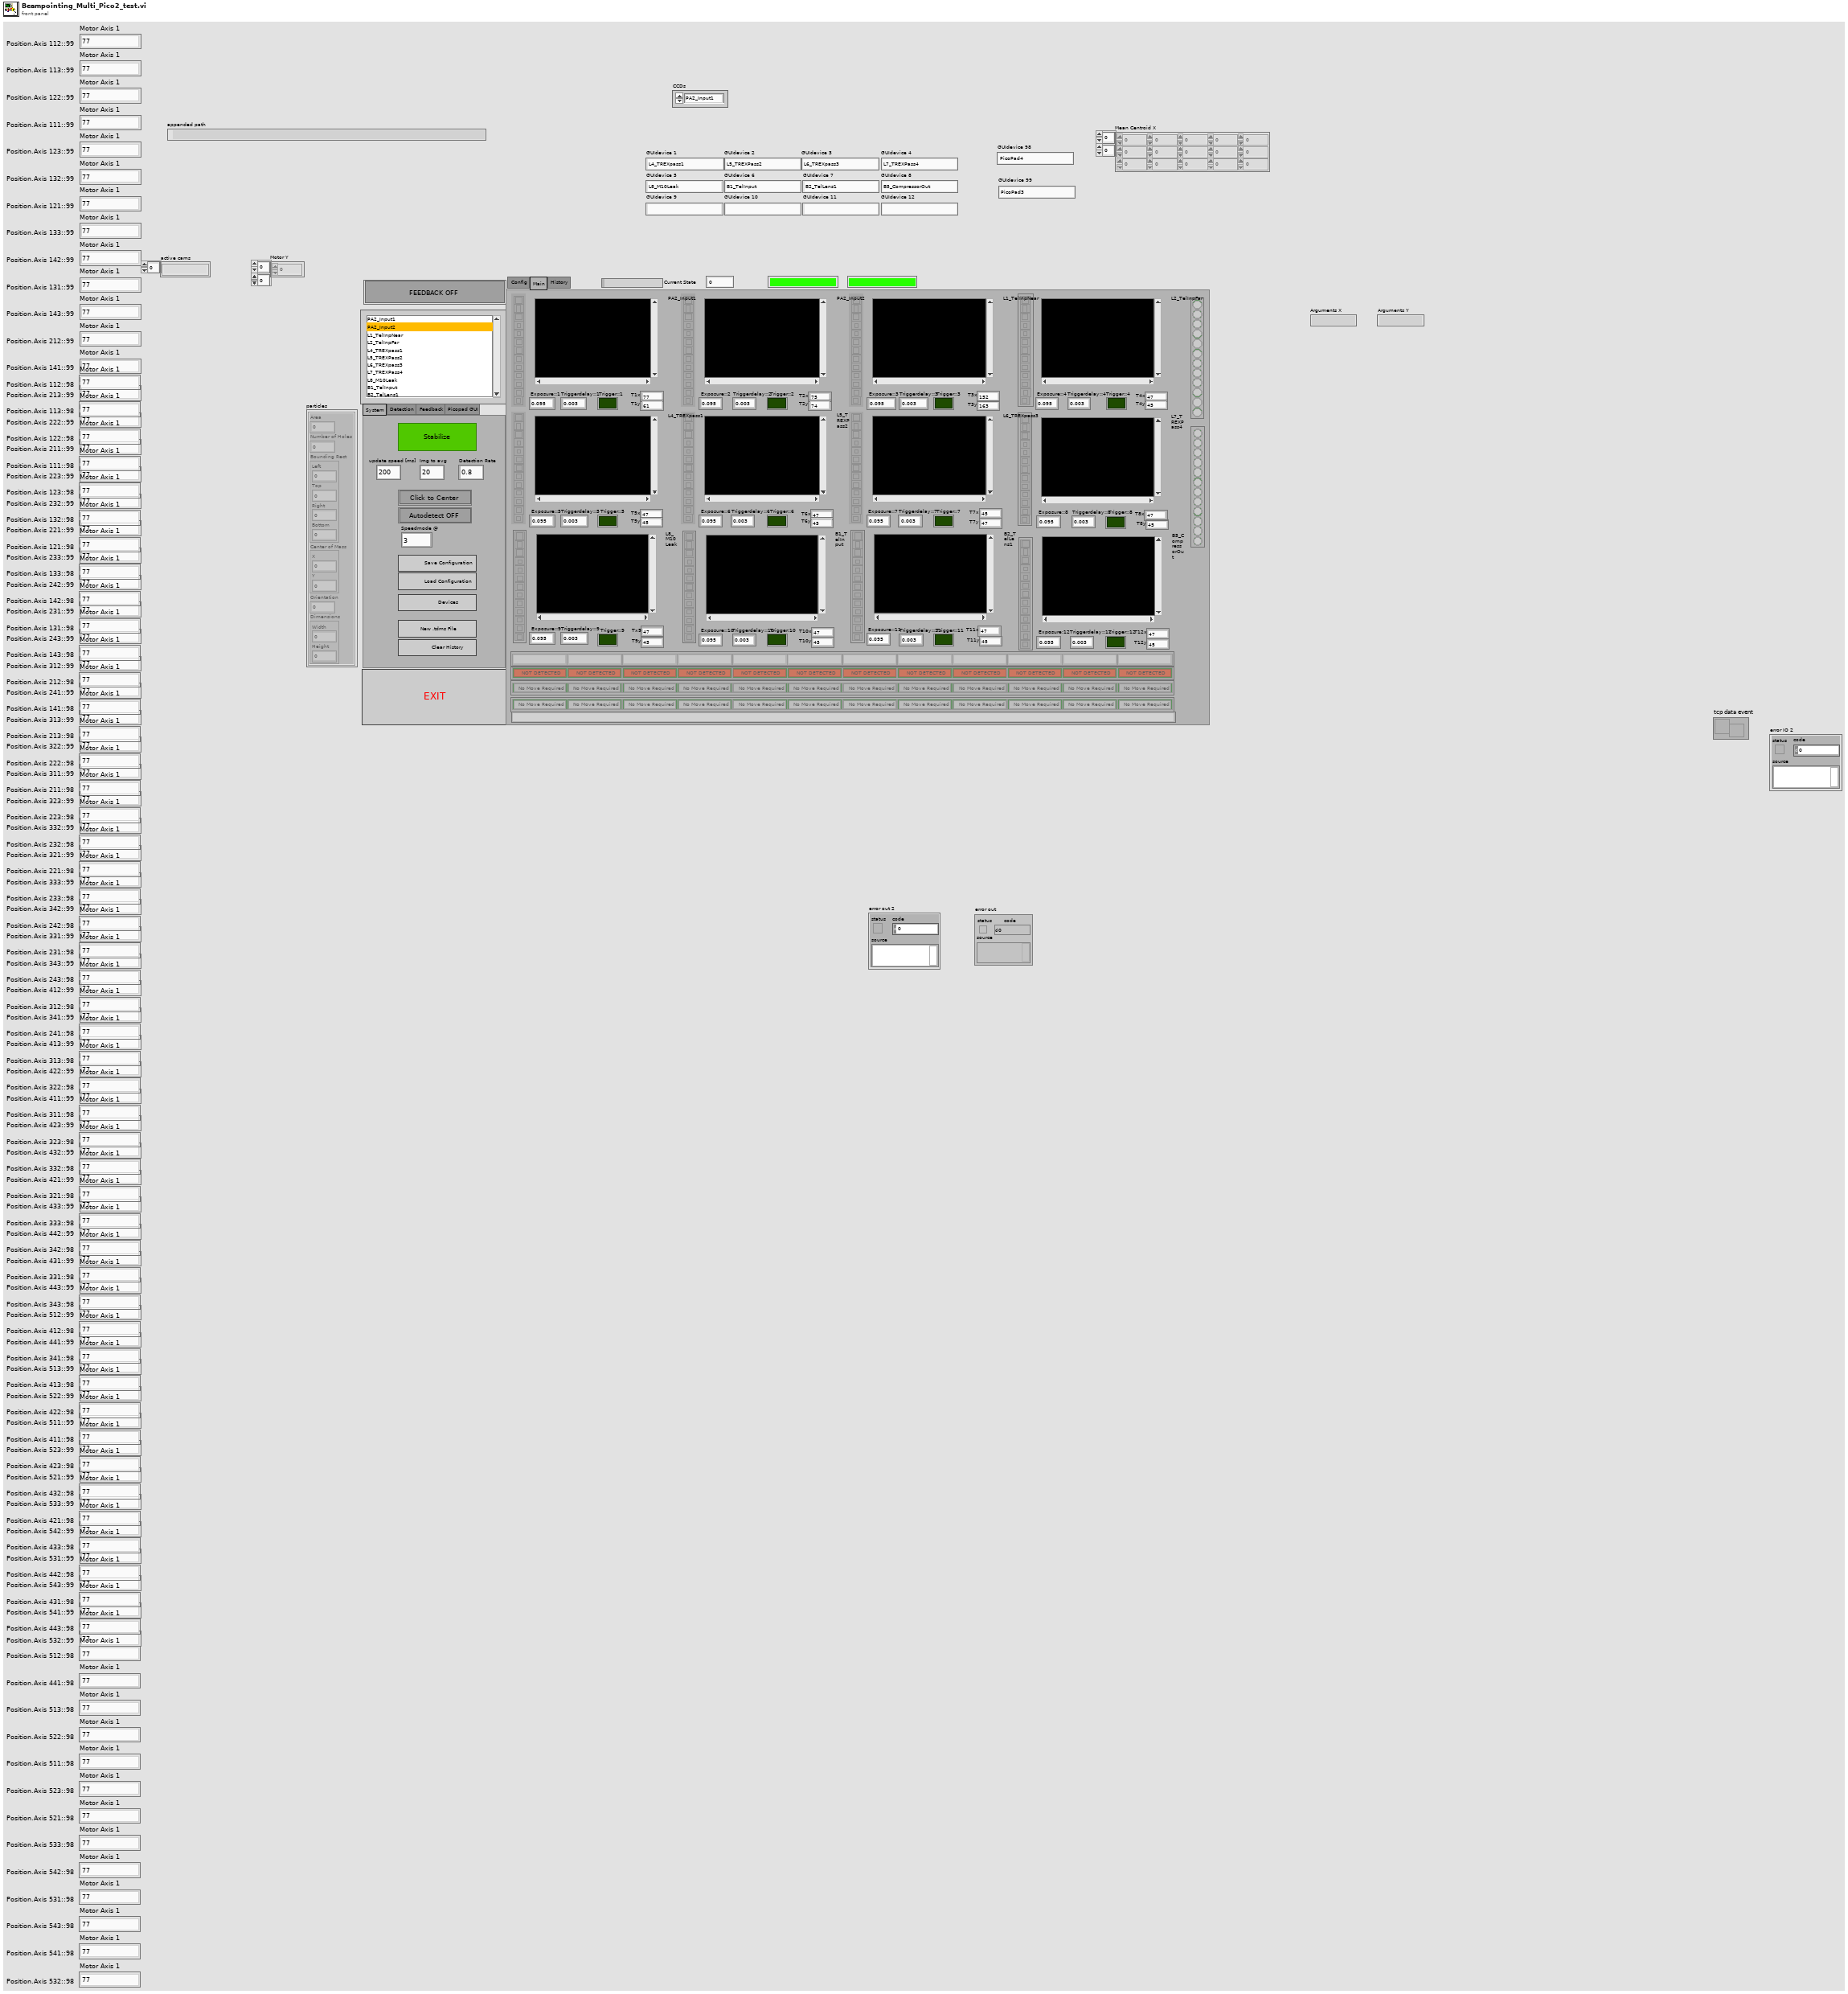
[diagram p1: front panel]
types:
  T1 = cluster{"Area":dbl, "Number of Holes":dbl, "Bounding Rect":cluster{"Left":dbl, "Top":dbl, "Right":dbl, "Bottom":dbl}, "Center of Mass":cluster{"X":dbl, "Y":dbl}, "Orientation":dbl, "Dimensions":cluster{"Width":dbl, "Height":dbl}}[]
  T2 = typedef "move.ctl" = cluster{"Tolerance [%]":dbl, "Stepsize":dbl, "Invert Axis":bool, "Invert Direction X":bool, "Invert Direction Y":bool, "enable feedback":bool, "Set Centriod Target":bool}
  T3 = typedef "beam detection.ctl" = cluster{"Filter":u16, "Filter Para":cluster{"X Size":i32, "Y Size":i32, "% Tolerance":i32}, "detection method":i32, "smal para":cluster{"Measurement Parameter":T4, "Range Lower Value":dbl, "Range Upper Value":dbl, "Range":bool, "Measurement Type":bool}[], "Remove small Objects":bool, "Restrict to round Objects":bool}
  T4 = typedef "Particle Parameters" = i32
  T5 = cluster{"CCDs":string[], "move properties":T2[], "detection para":T3[], "thresholds":cluster{"Lower value":sgl, "Upper value":sgl}[], "Value":cluster{"Motor CCD 1":u16, "Motor CCD 2":u16, "Motor CCD 3":u16, "Motor CCD 4":u16, "Motor CCD 5":u16, "Motor CCD 6":u16, "Motor CCD 7":u16, "Motor CCD 8":u16, "Motor CCD 9":u16, "Motor CCD 10":u16, "Motor CCD 11":u16, "Motor CCD 12":u16}}
  T6 = cluster{"Left":dbl, "Top":dbl, "Right":dbl, "Bottom":dbl}[]
  T7 = cluster{"Motor CCD 1":u16, "Motor CCD 2":u16, "Motor CCD 3":u16, "Motor CCD 4":u16, "Motor CCD 5":u16, "Motor CCD 6":u16, "Motor CCD 7":u16, "Motor CCD 8":u16, "Motor CCD 9":u16, "Motor CCD 10":u16, "Motor CCD 11":u16, "Motor CCD 12":u16}
  T8 = cluster{"[0]":string, "[1]":string, "[2]":string, "[3]":string, "[4]":string, "[5]":string, "[6]":string, "[7]":string, "[8]":string, "[8] 2":string, "[8] 3":string, "[8] 4":string}
  T9 = typedef "IMAQ Image.ctl" = refnum<image>
  T10 = cluster{"Area":dbl, "Number of Holes":dbl, "Bounding Rect":cluster{"Left":dbl, "Top":dbl, "Right":dbl, "Bottom":dbl}, "Center of Mass":cluster{"X":dbl, "Y":dbl}, "Orientation":dbl, "Dimensions":cluster{"Width":dbl, "Height":dbl}}[][]
  T11 = enum32{"System", "Detection", "Feedback", "Picopad GUI"}
  T12 = cluster{"Ref X":refnum<vi>, "Ref Y":refnum<vi>}[]
  T13 = typedef "tcp_new_data_event.ctl" = refnum<user-event>
  T14 = typedef "tcp new data cluster.ctl" = cluster{"EventEnum":enum16{"new data", "connection status update"}, "Device name":string}
  T15 = cluster{"Left":i32, "Top":i32, "Right":i32, "Bottom":i32}
  T16 = enum32{"invalid app kind", "Development System", "Run Time System", "Student Edition", "Embedded LabVIEW", "Evaluation", "Custom"}
  T17 = enum16{"open", "open or create", "create or replace", "create", "open (read-only)"}
  T18 = enum32{"Invalid", "Standard", "Closed", "Hidden", "Minimized", "Maximized"}
  T19 = enum16{"open", "replace", "create", "open or create", "replace or create", "replace or create with confirmation"}
  T20 = typedef "Image Type" = u32
  T21 = cluster{"[0]":string, "[1]":string, "[2]":string, "[3]":string, "[4]":string, "[5]":string, "[6]":string, "[7]":string, "[8]":string, "[9]":string, "[10]":string, "[11]":string}
  T22 = cluster{"Target.X::1":refnum<vi>, "Target.Y::1":refnum<vi>}
  T23 = cluster{"Target.X::2":refnum<vi>, "Target.Y::2":refnum<vi>}
  T24 = cluster{"Target.X::3":refnum<vi>, "Target.Y::3":refnum<vi>}
  T25 = cluster{"Target.X::4":refnum<vi>, "Target.Y::4":refnum<vi>}
  T26 = cluster{"Target.X::5":refnum<vi>, "Target.Y::5":refnum<vi>}
  T27 = cluster{"Target.X::6":refnum<vi>, "Target.Y::6":refnum<vi>}
  T28 = cluster{"Target.X::7":refnum<vi>, "Target.Y::7":refnum<vi>}
  T29 = cluster{"Target.X::8":refnum<vi>, "Target.Y::8":refnum<vi>}
  T30 = cluster{"Target.X::12":refnum<vi>, "Target.Y::12":refnum<vi>}
  T31 = cluster{"Target.X::9":refnum<vi>, "Target.Y::9":refnum<vi>}
  T32 = cluster{"Target.X::10":refnum<vi>, "Target.Y::10":refnum<vi>}
  T33 = cluster{"Target.X::11":refnum<vi>, "Target.Y::11":refnum<vi>}
  T34 = cluster{"Target.X::12":refnum<vi>, "Target.Y::12":refnum<vi>}[]
  T35 = cluster{"Left":dbl, "Top":dbl, "Right":dbl, "Bottom":dbl}
  T36 = cluster{"Core":cluster{"Current VI Reference":refnum<vi>, "Close Panel on Exit?":bool}, "detection para":T3[], "thresholds":cluster{"Lower value":sgl, "Upper value":sgl}[], "Centroid X":dbl[][], "Centroid Y":dbl[][], "img to avg":i32, "Mean Centroid X":dbl[][], "Mean Centroid Y":dbl[][], "Offset X":dbl[][], "Offset Y":dbl[][], "Offset X stats ":dbl[][], "Offset Y stats ":dbl[][], "Size":dbl[][], "Mean Size":dbl[][], "Time":timestamp[][], "move properties":T2[], "active axis refs 2":cluster{"Ref X":refnum<vi>, "Ref Y":refnum<vi>}[], "active ccd":i32, "Feedback global":bool, "Motor X":dbl[][], "Motor Y":dbl[][], "active cams":string[], "Data Value Reference out":refnum<k34>, "detected":bool[], "speedmode X":bool[], "speedmode Y":bool[]}
  T37 = cluster{"Current VI Reference":refnum<vi>, "Close Panel on Exit?":bool}
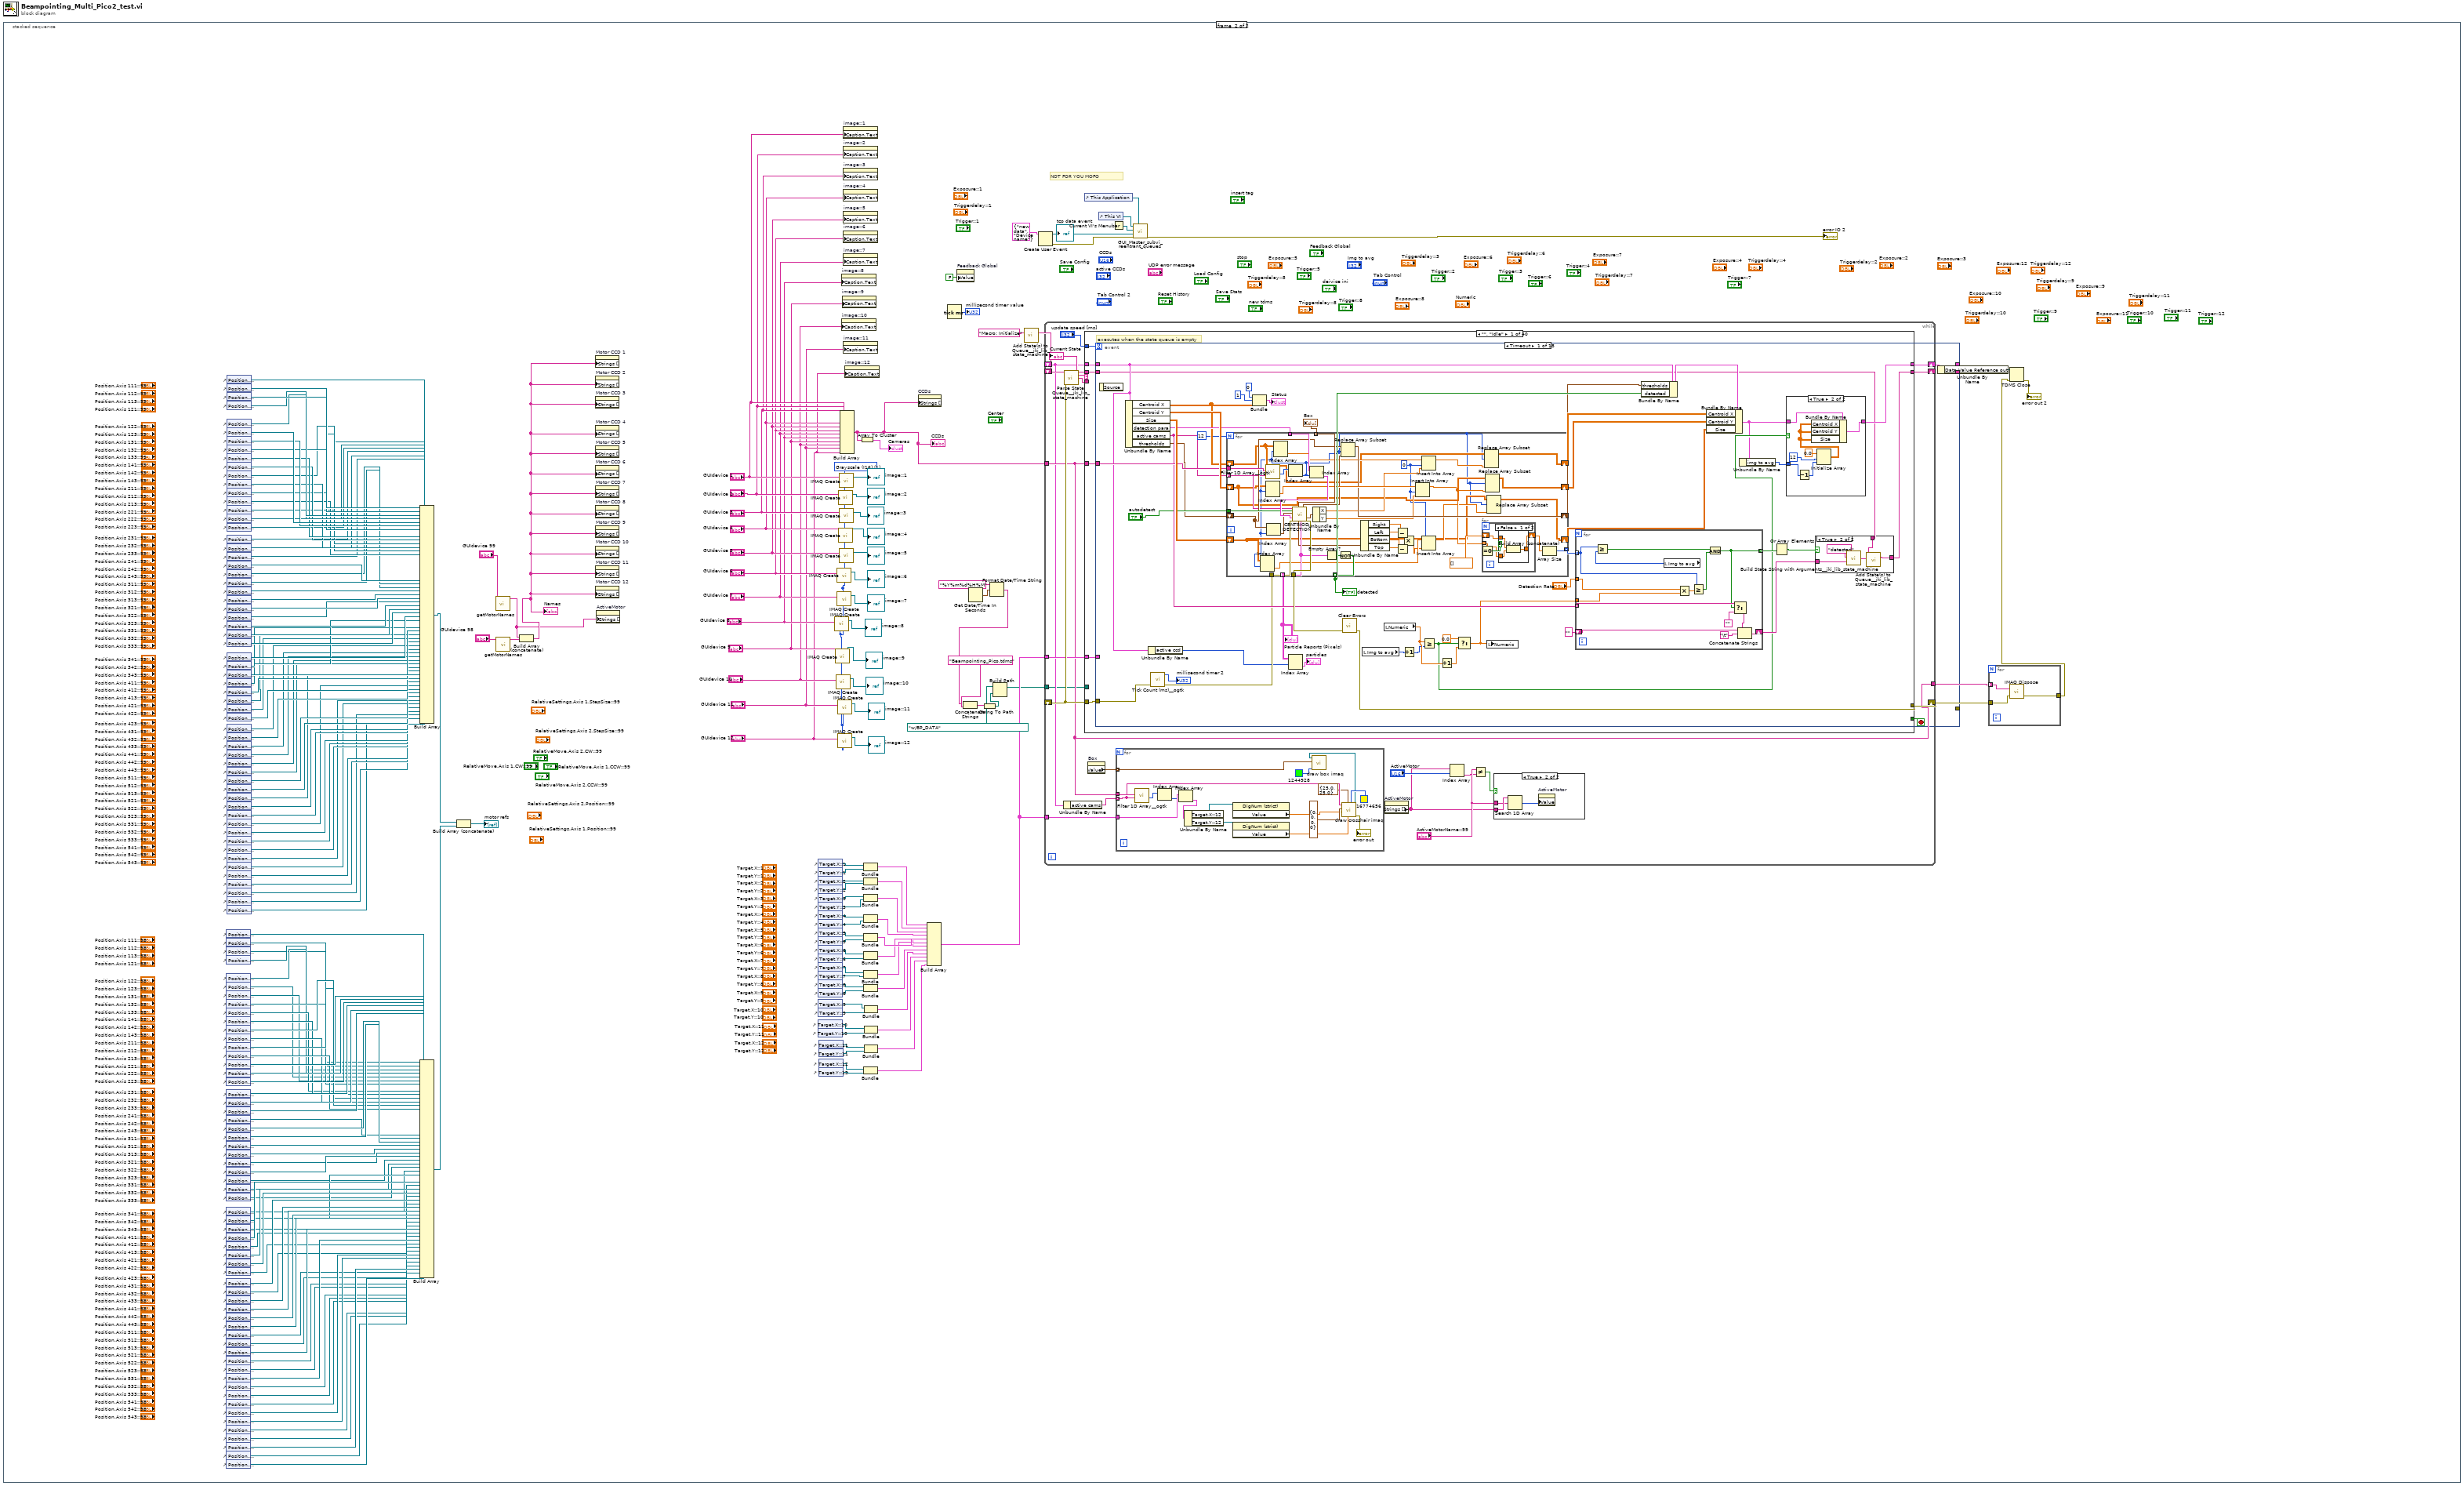
[diagram p0: block diagram]
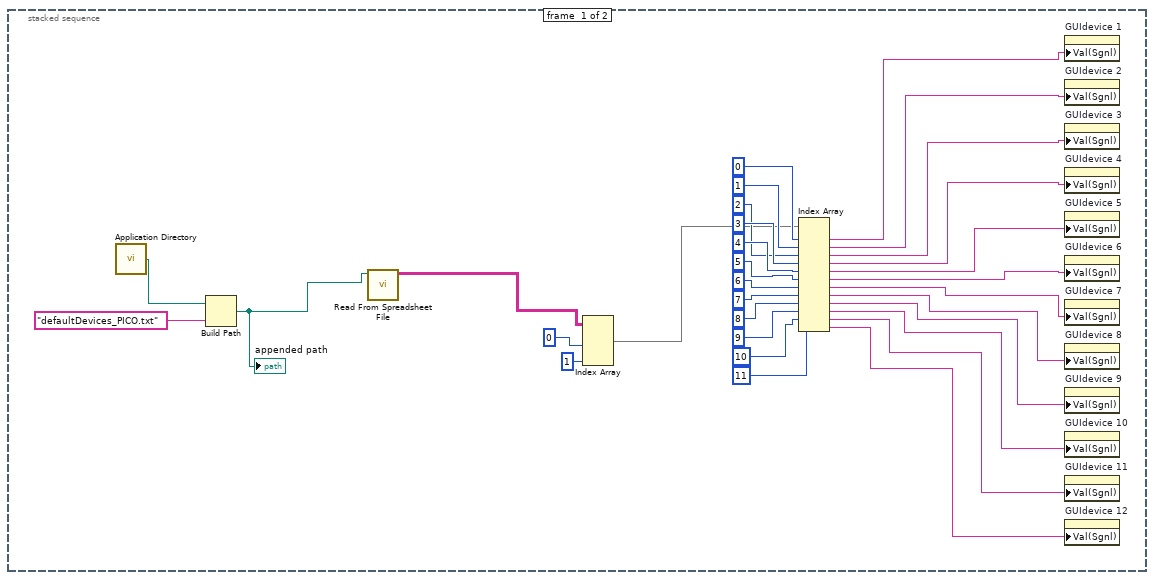
[diagram p2: hidden frame]
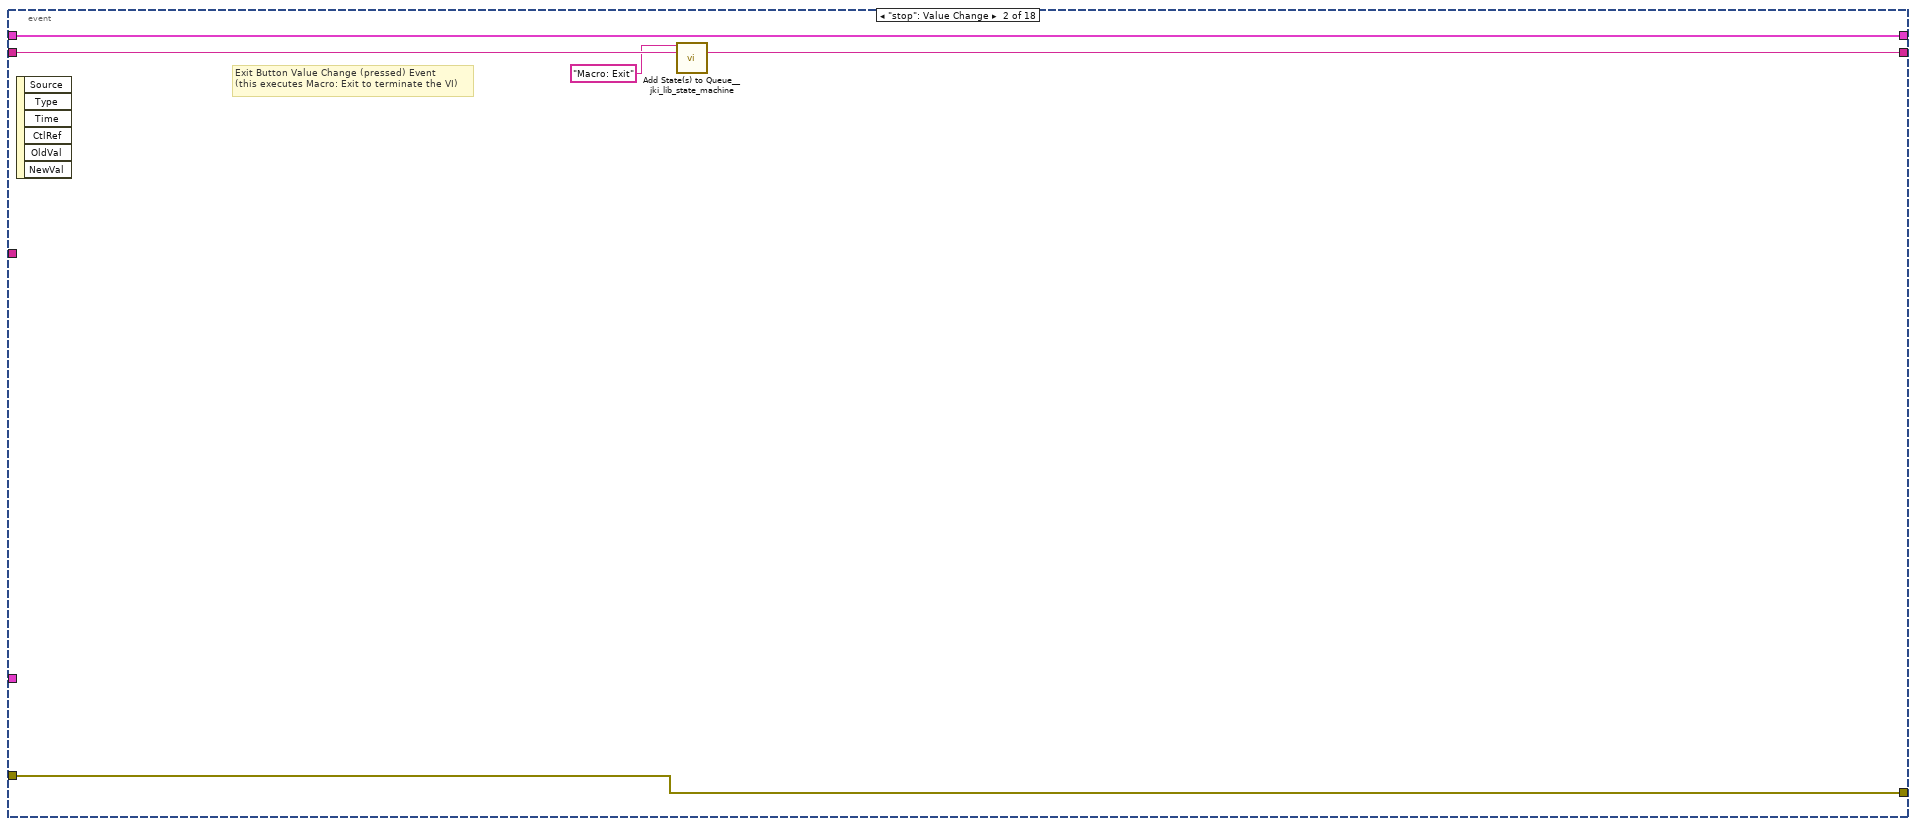
[diagram p7: hidden frame]
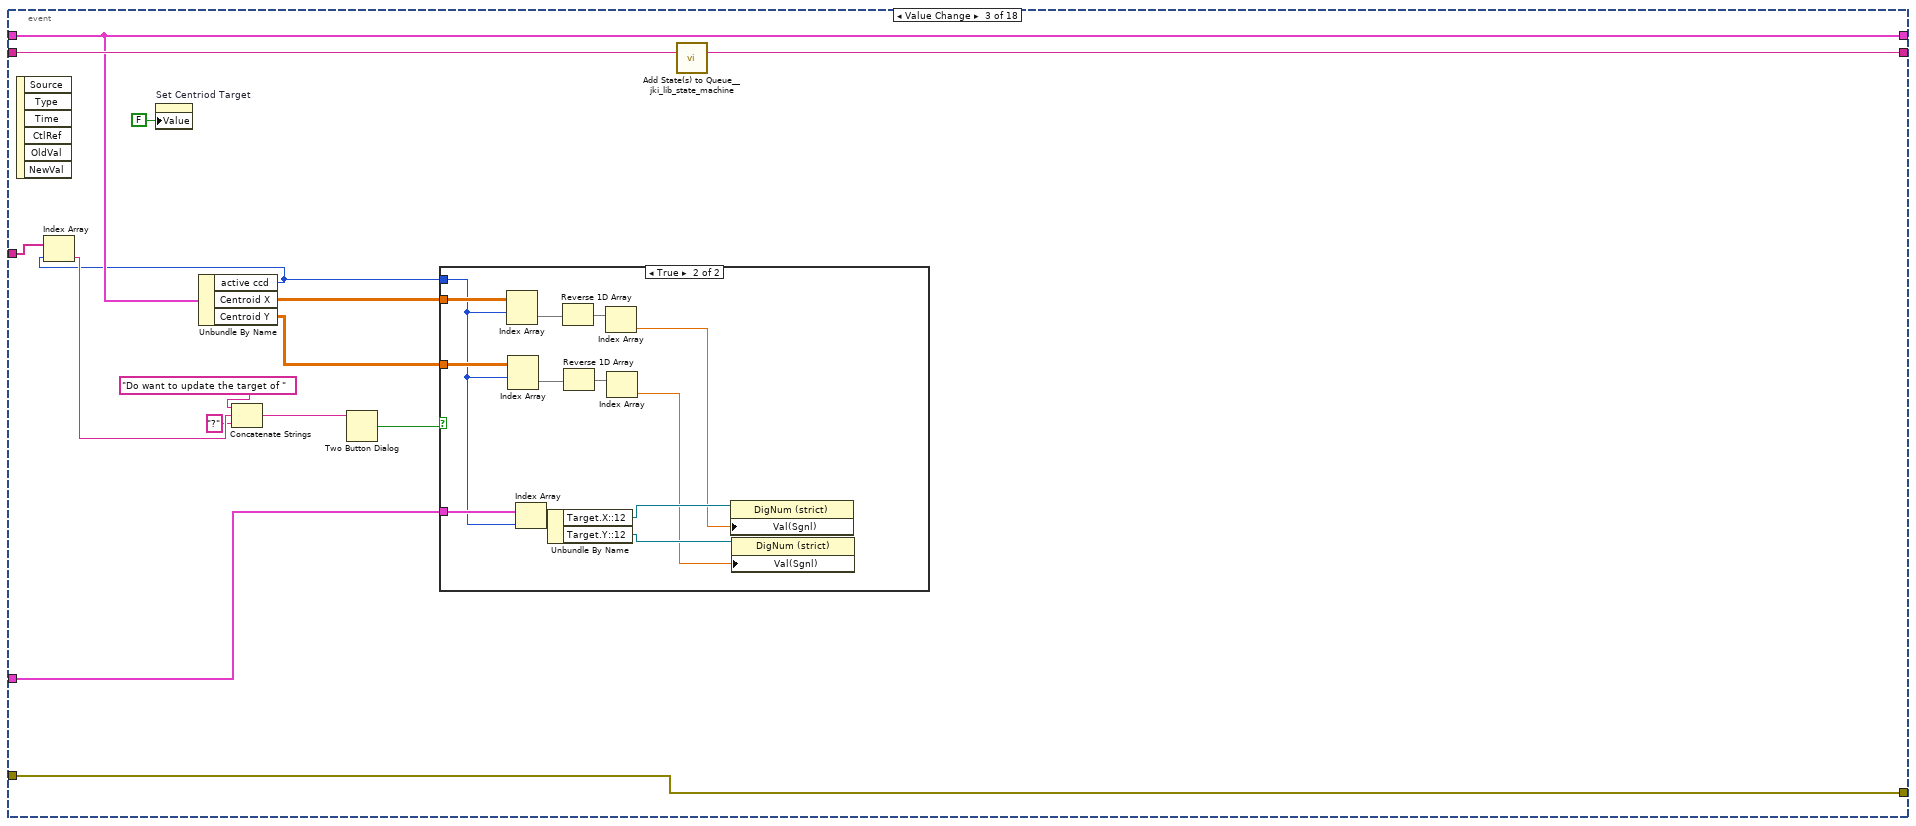
[diagram p8: hidden frame]
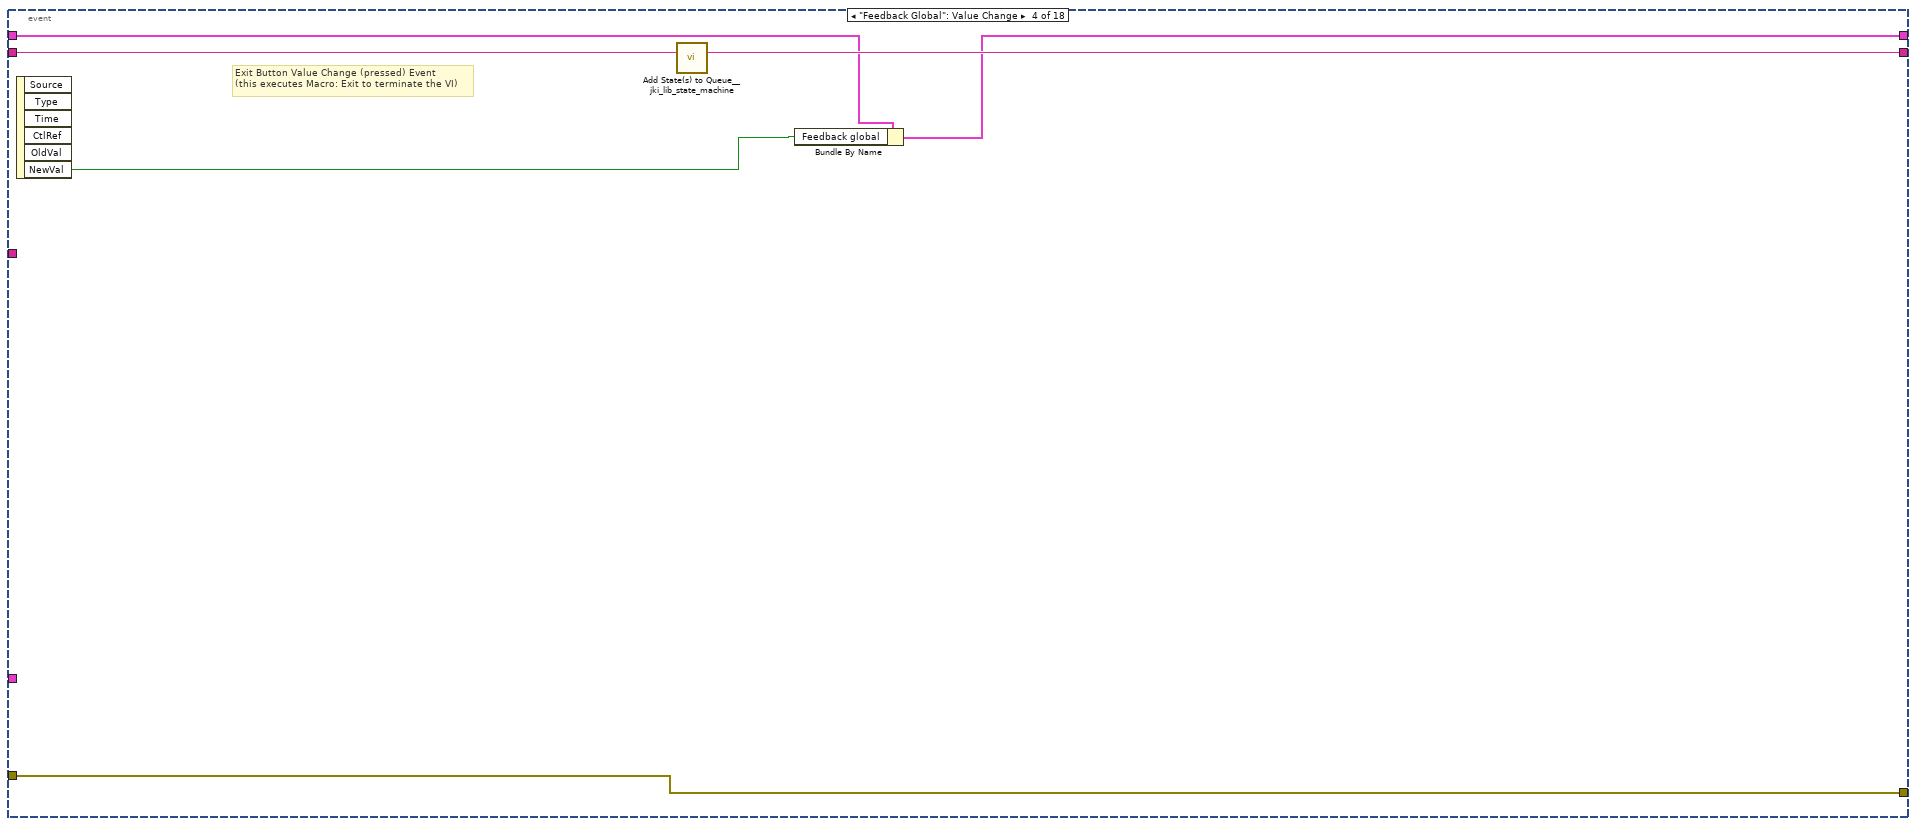
[diagram p10: hidden frame]
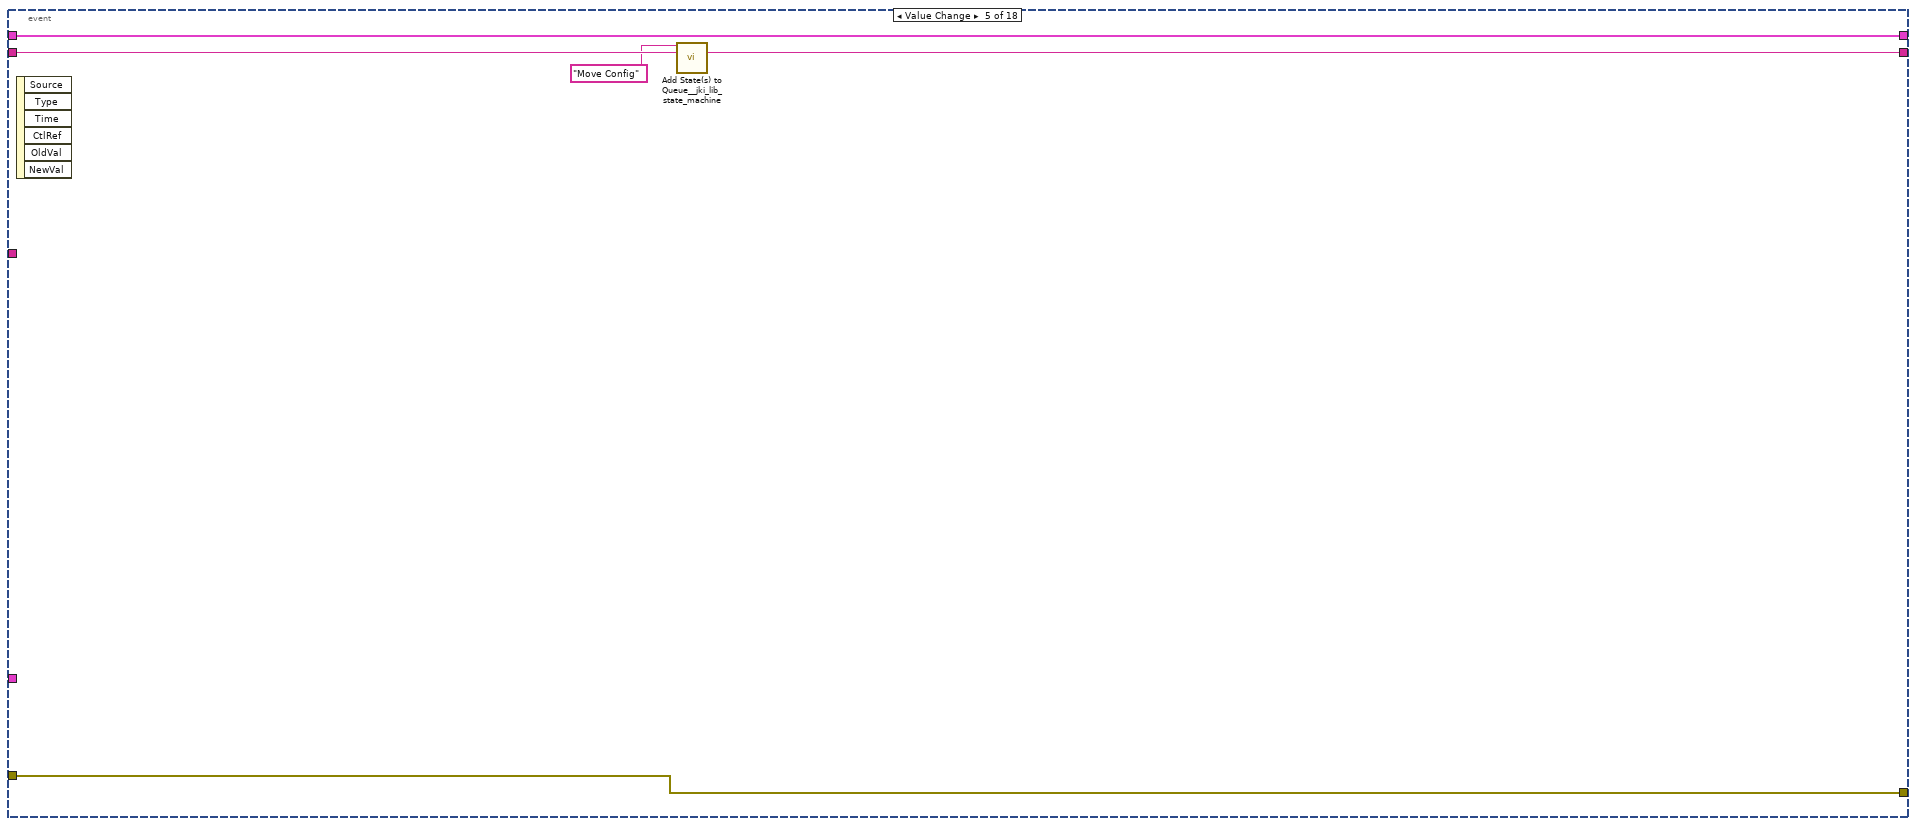
[diagram p11: hidden frame]
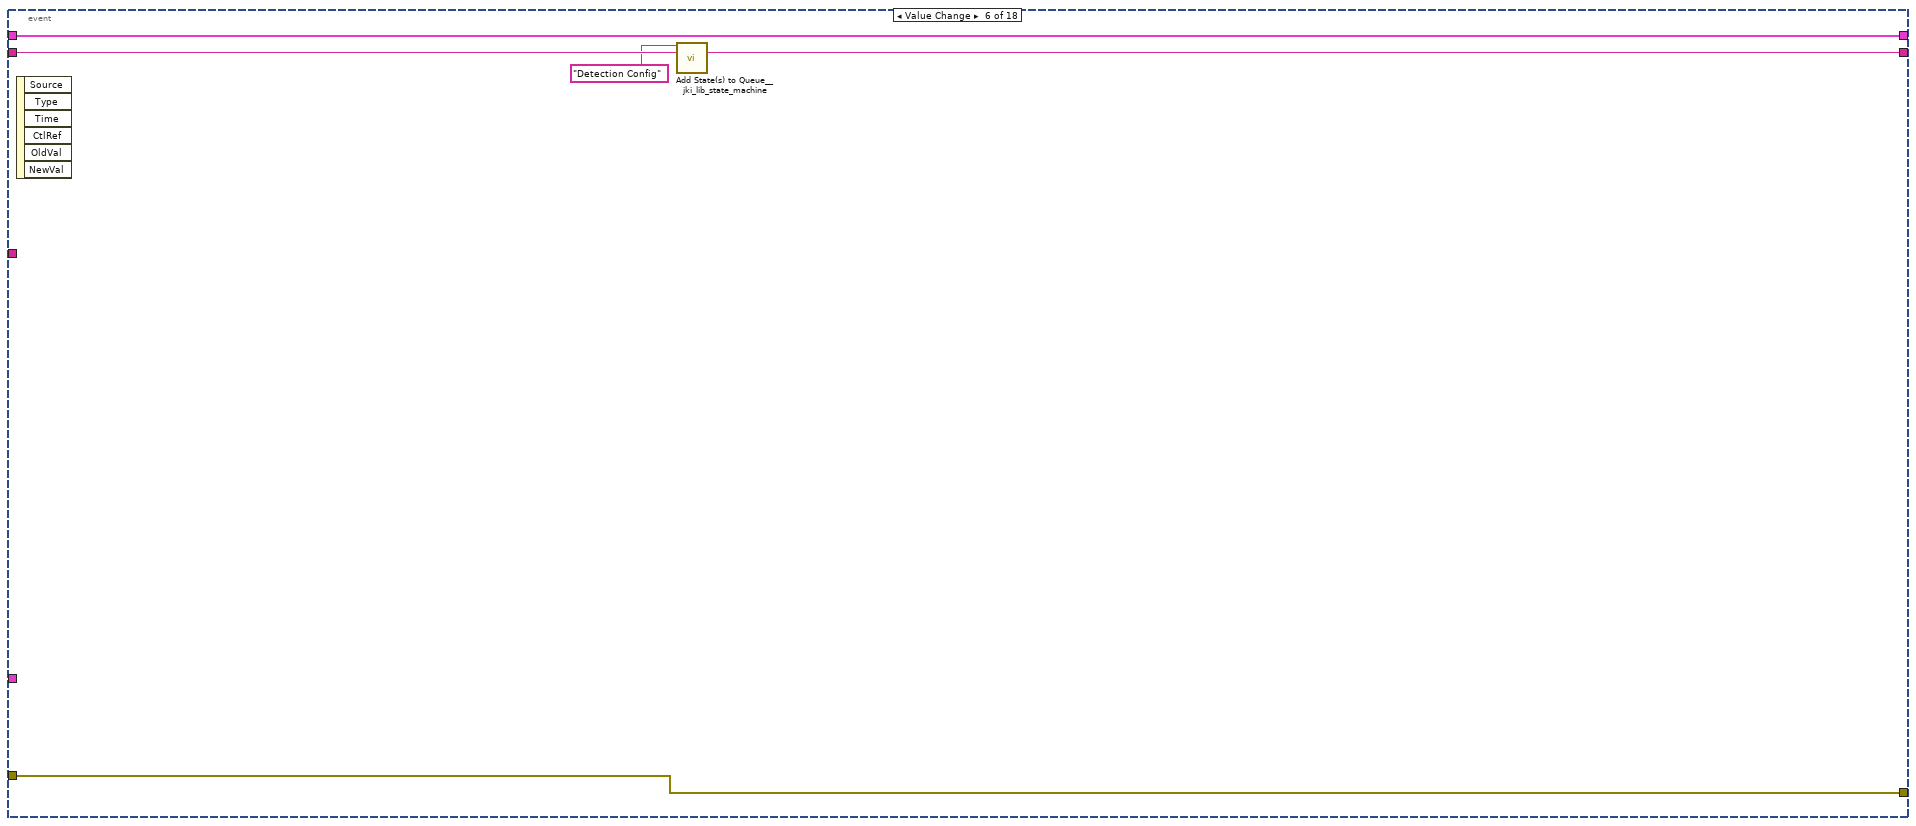
[diagram p12: hidden frame]
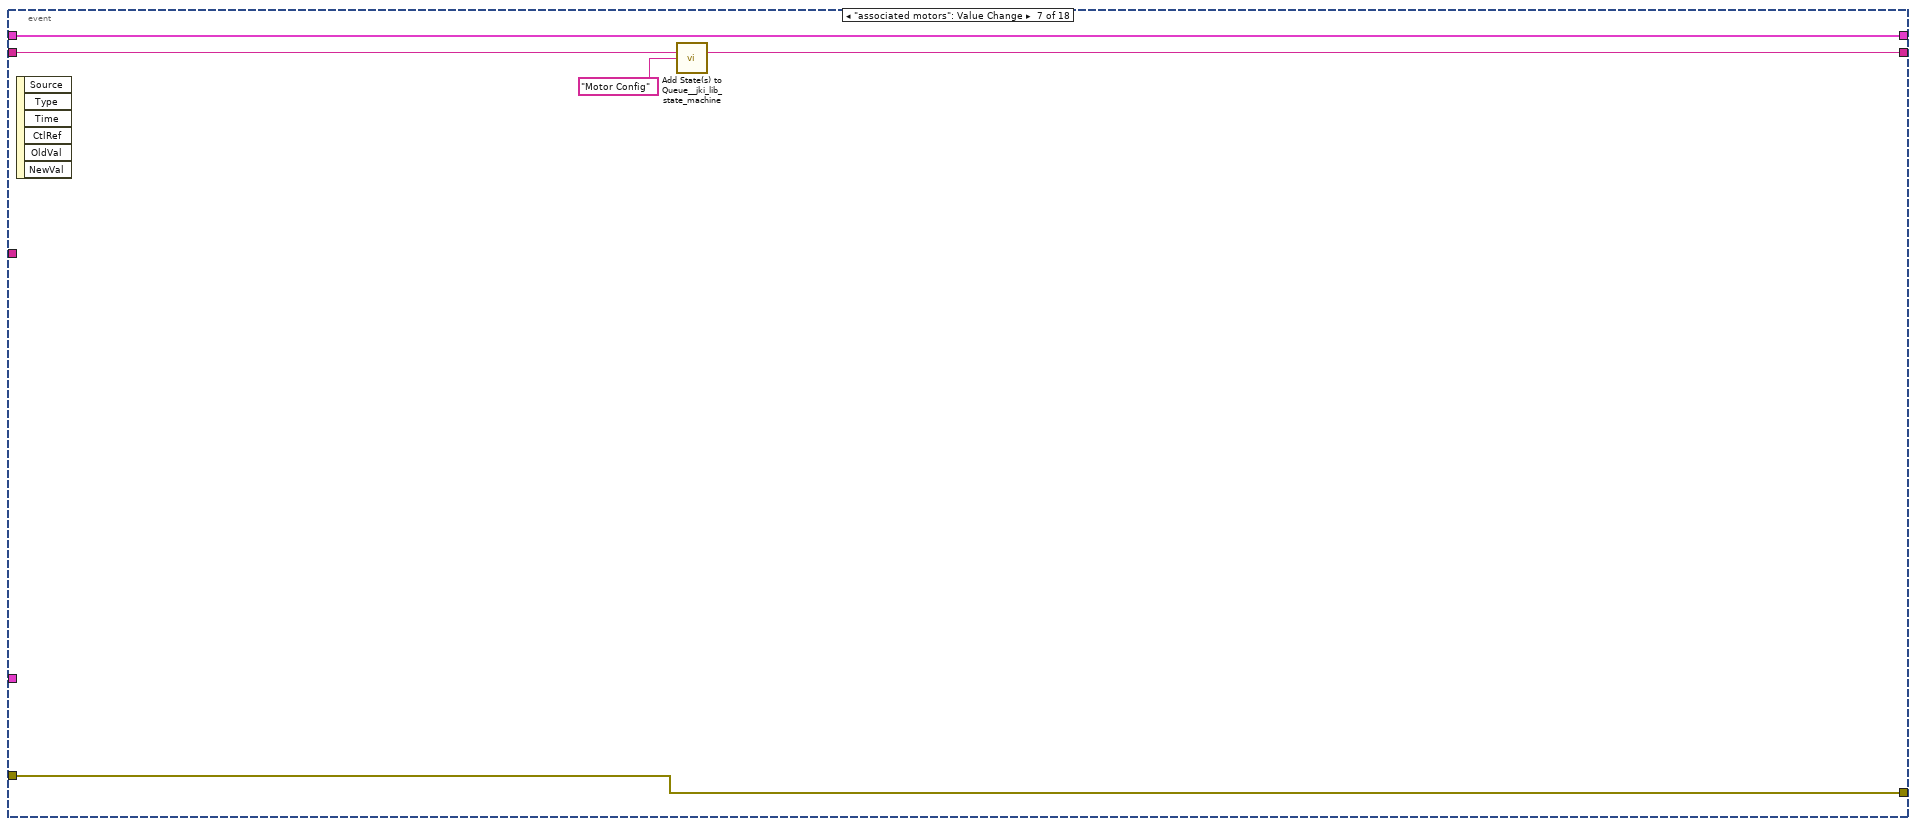
[diagram p13: hidden frame]
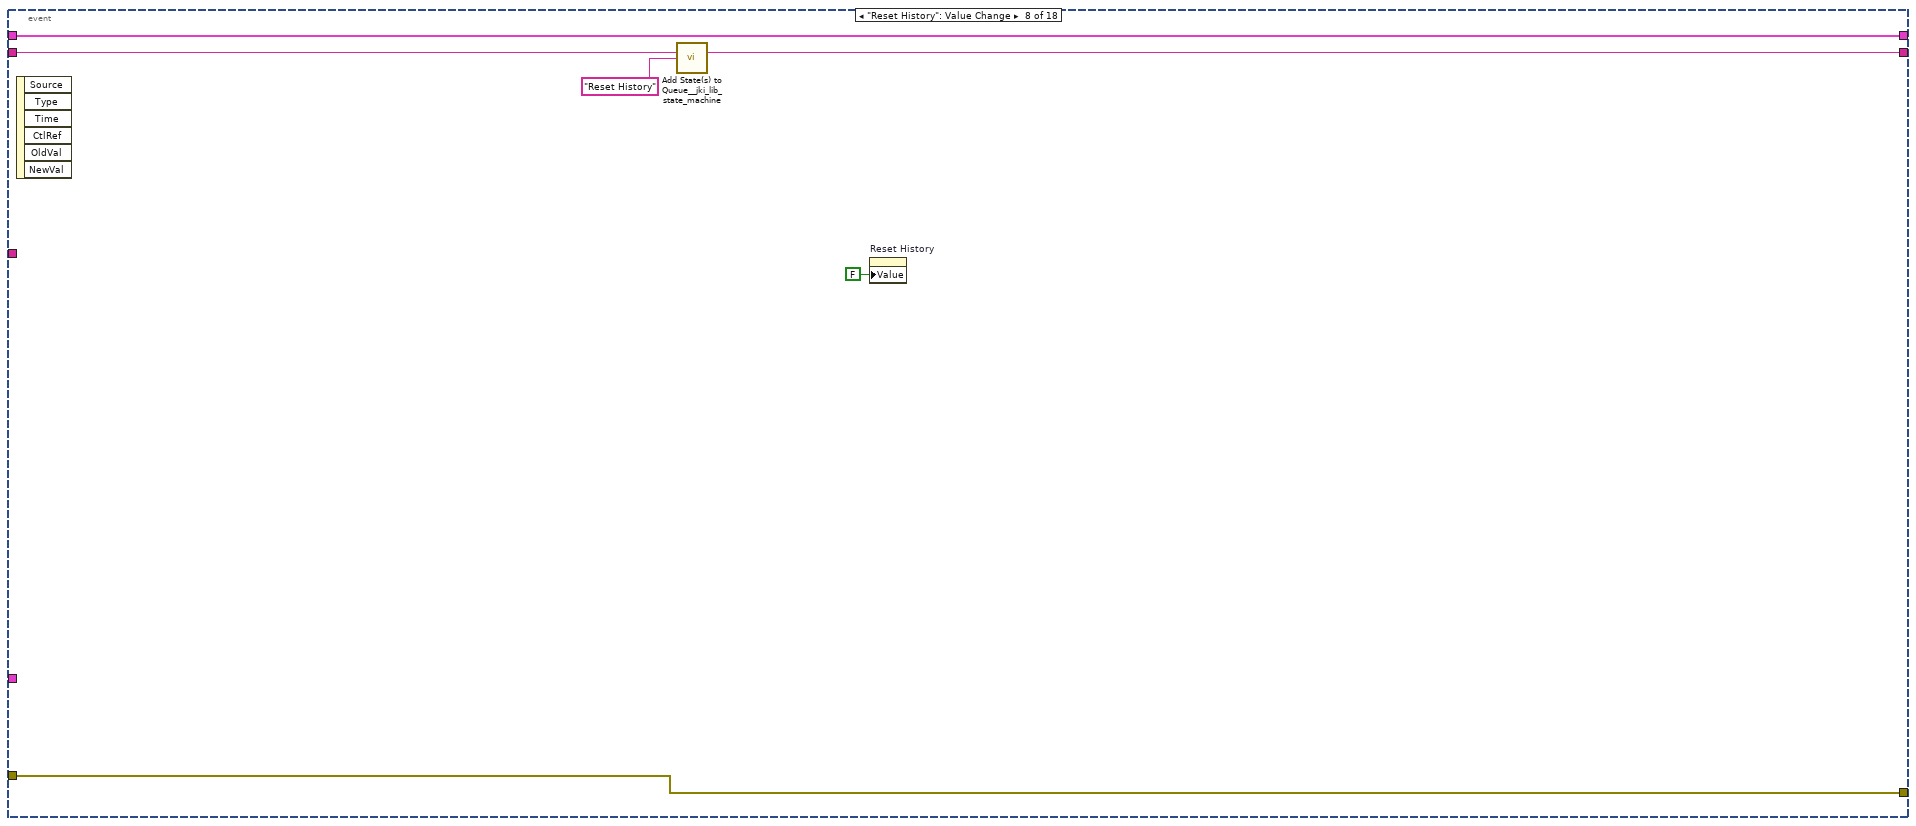
[diagram p14: hidden frame]
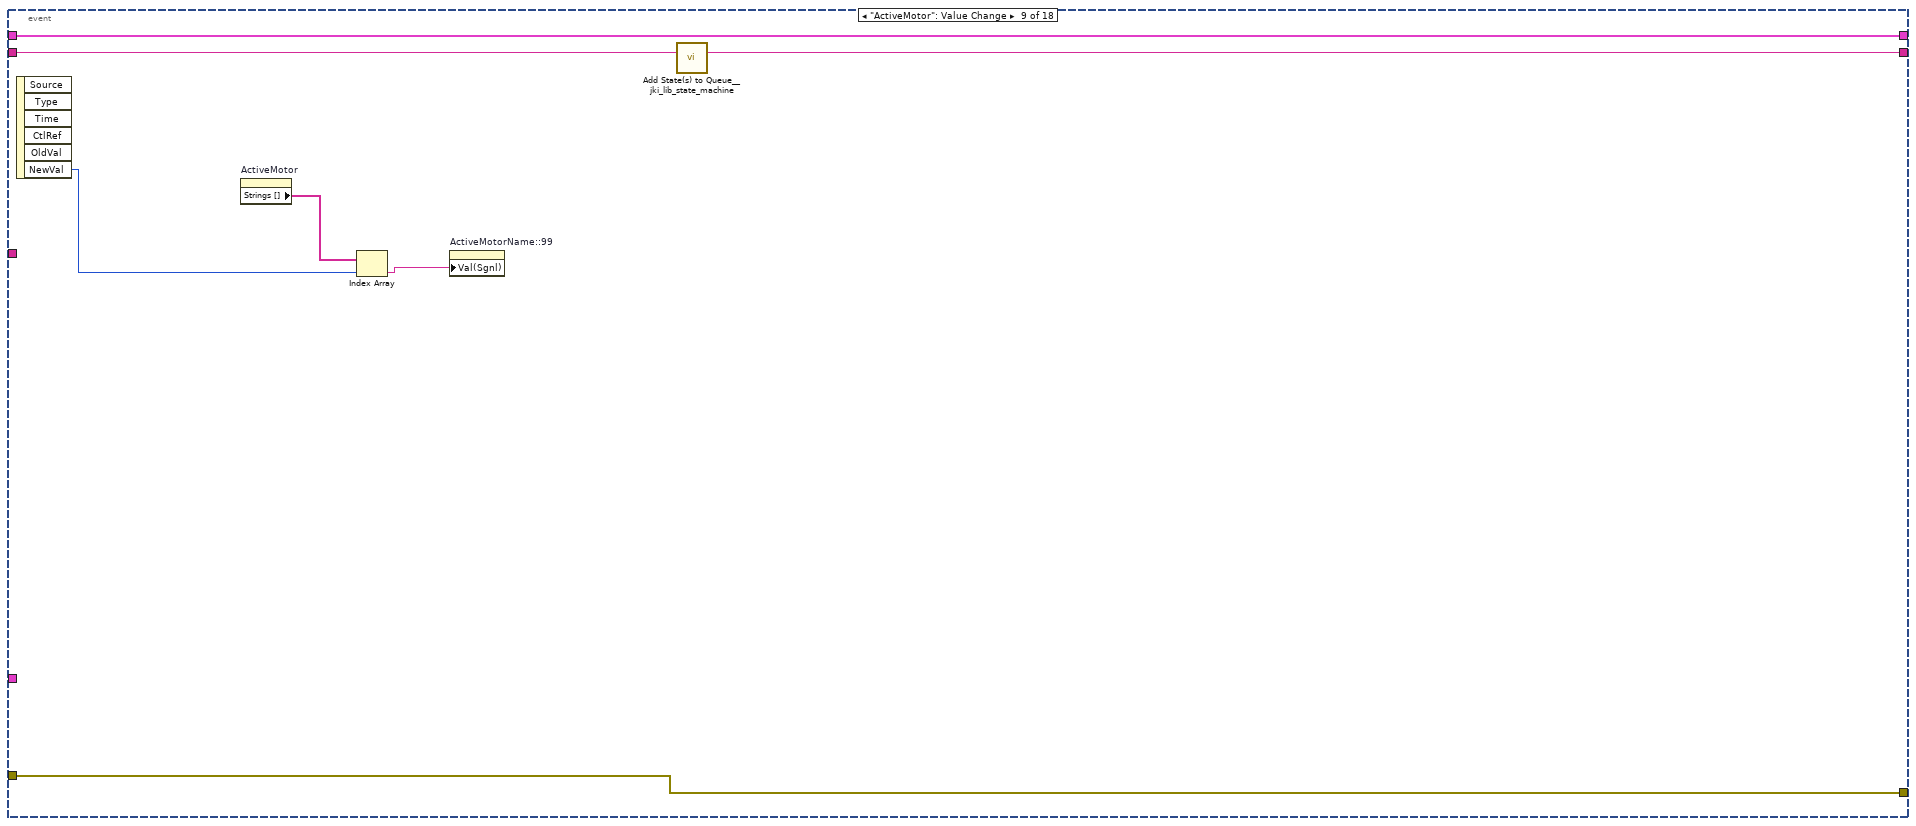
[diagram p15: hidden frame]
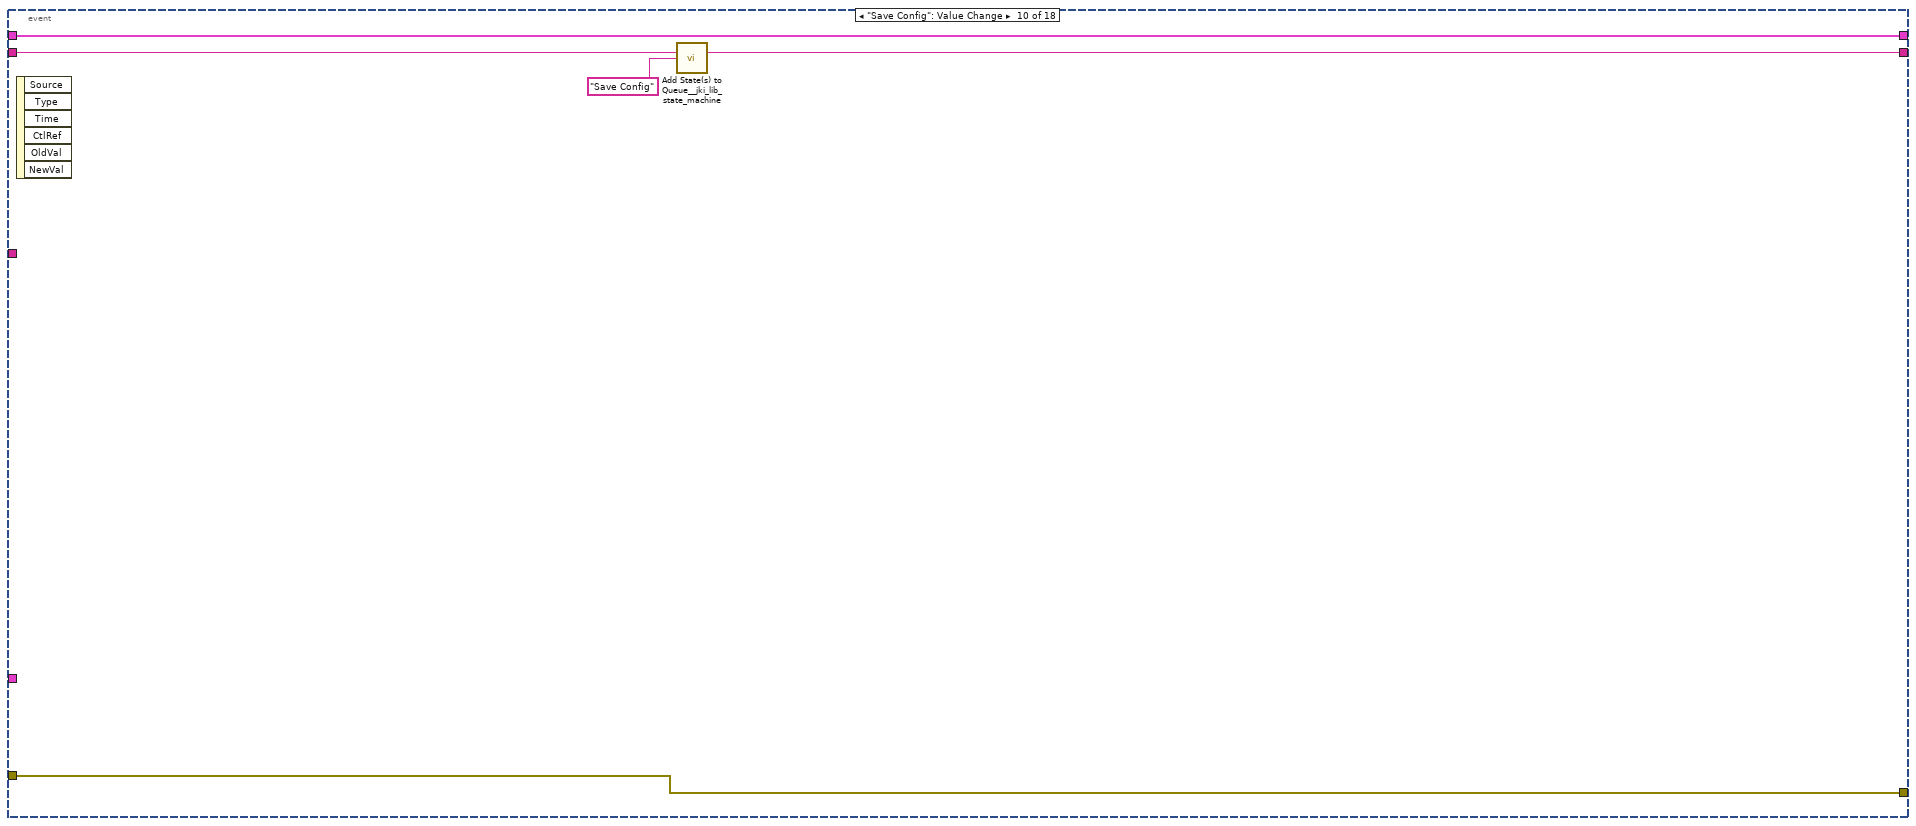
[diagram p16: hidden frame]
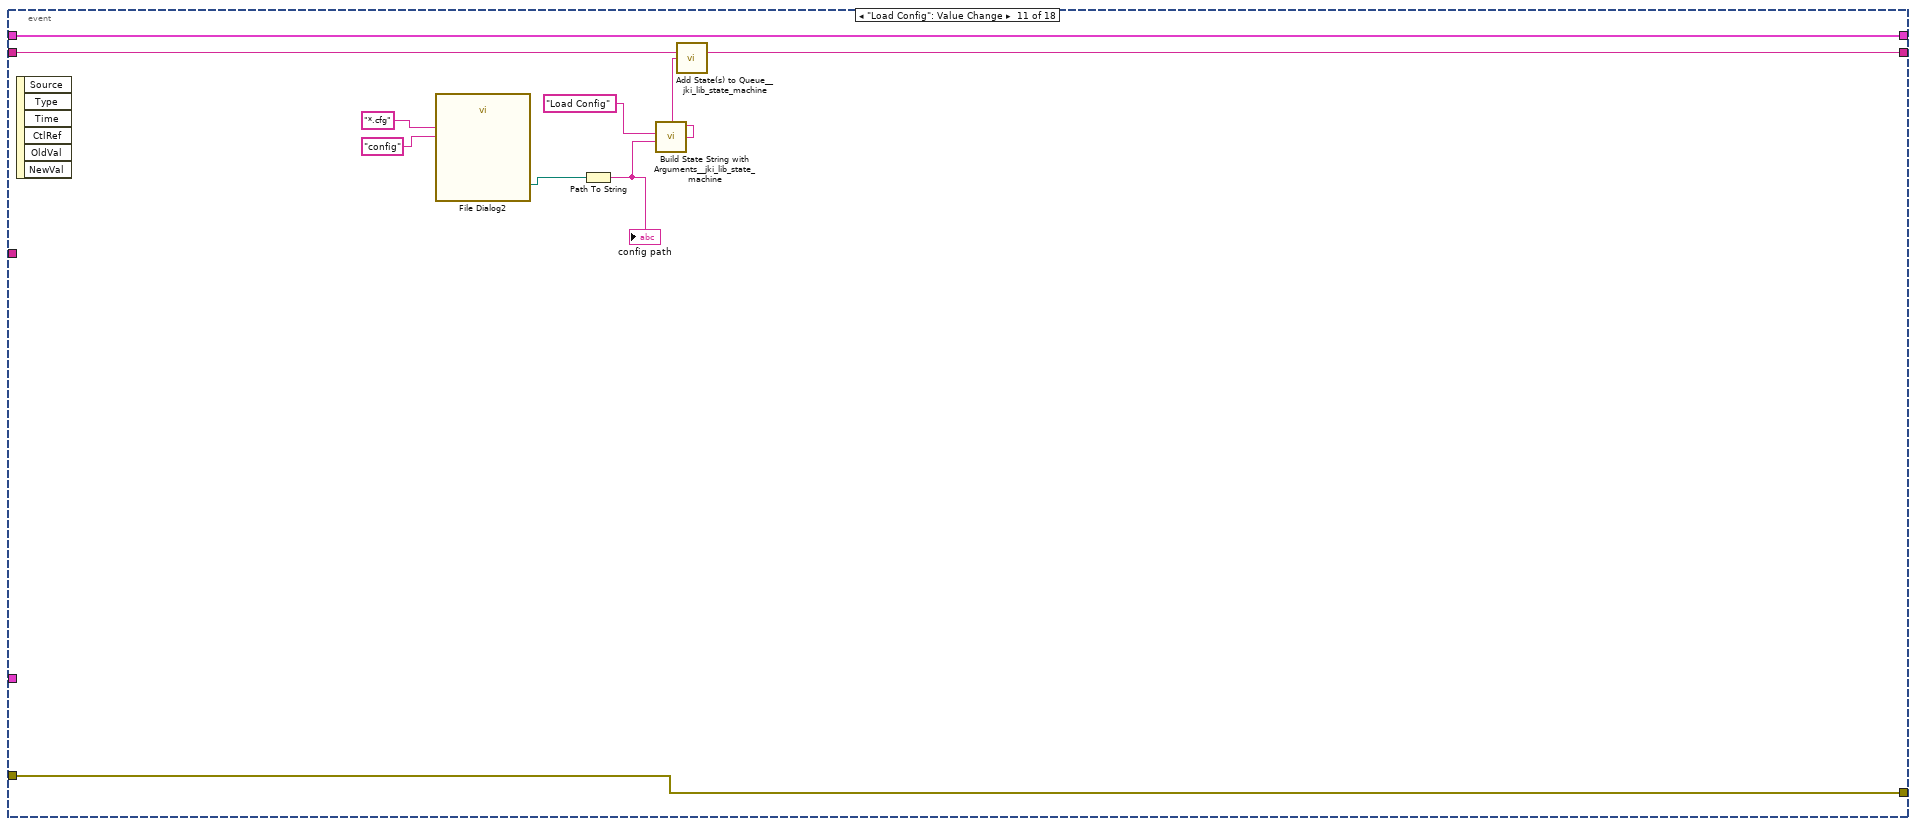
[diagram p17: hidden frame]
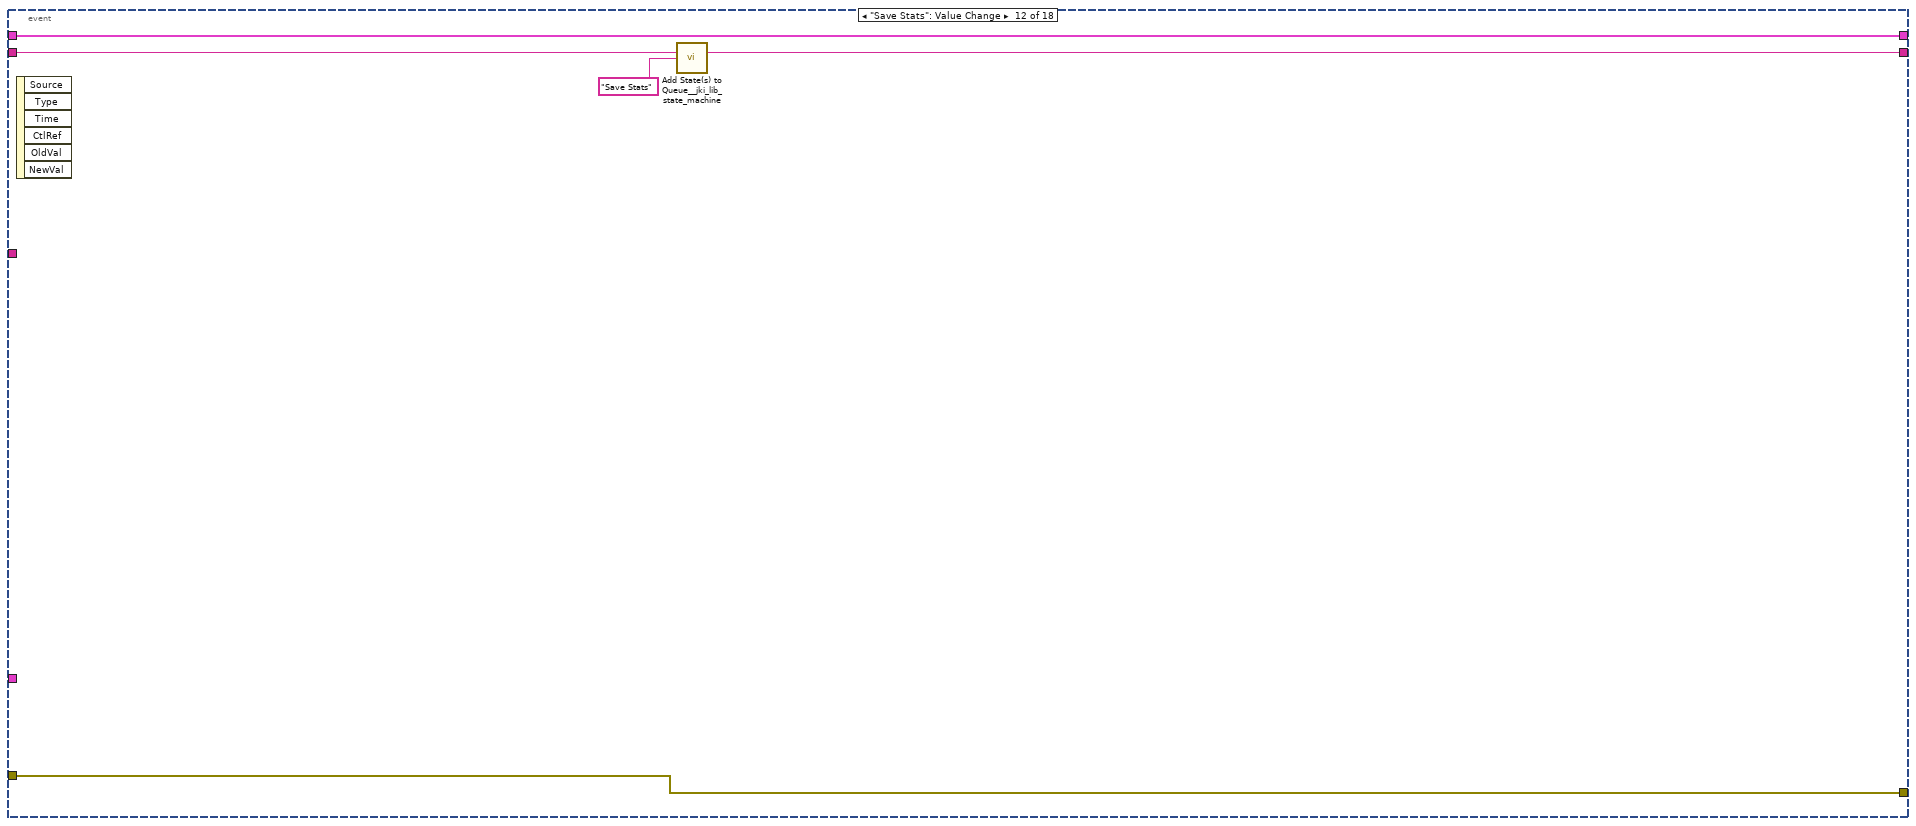
[diagram p18: hidden frame]
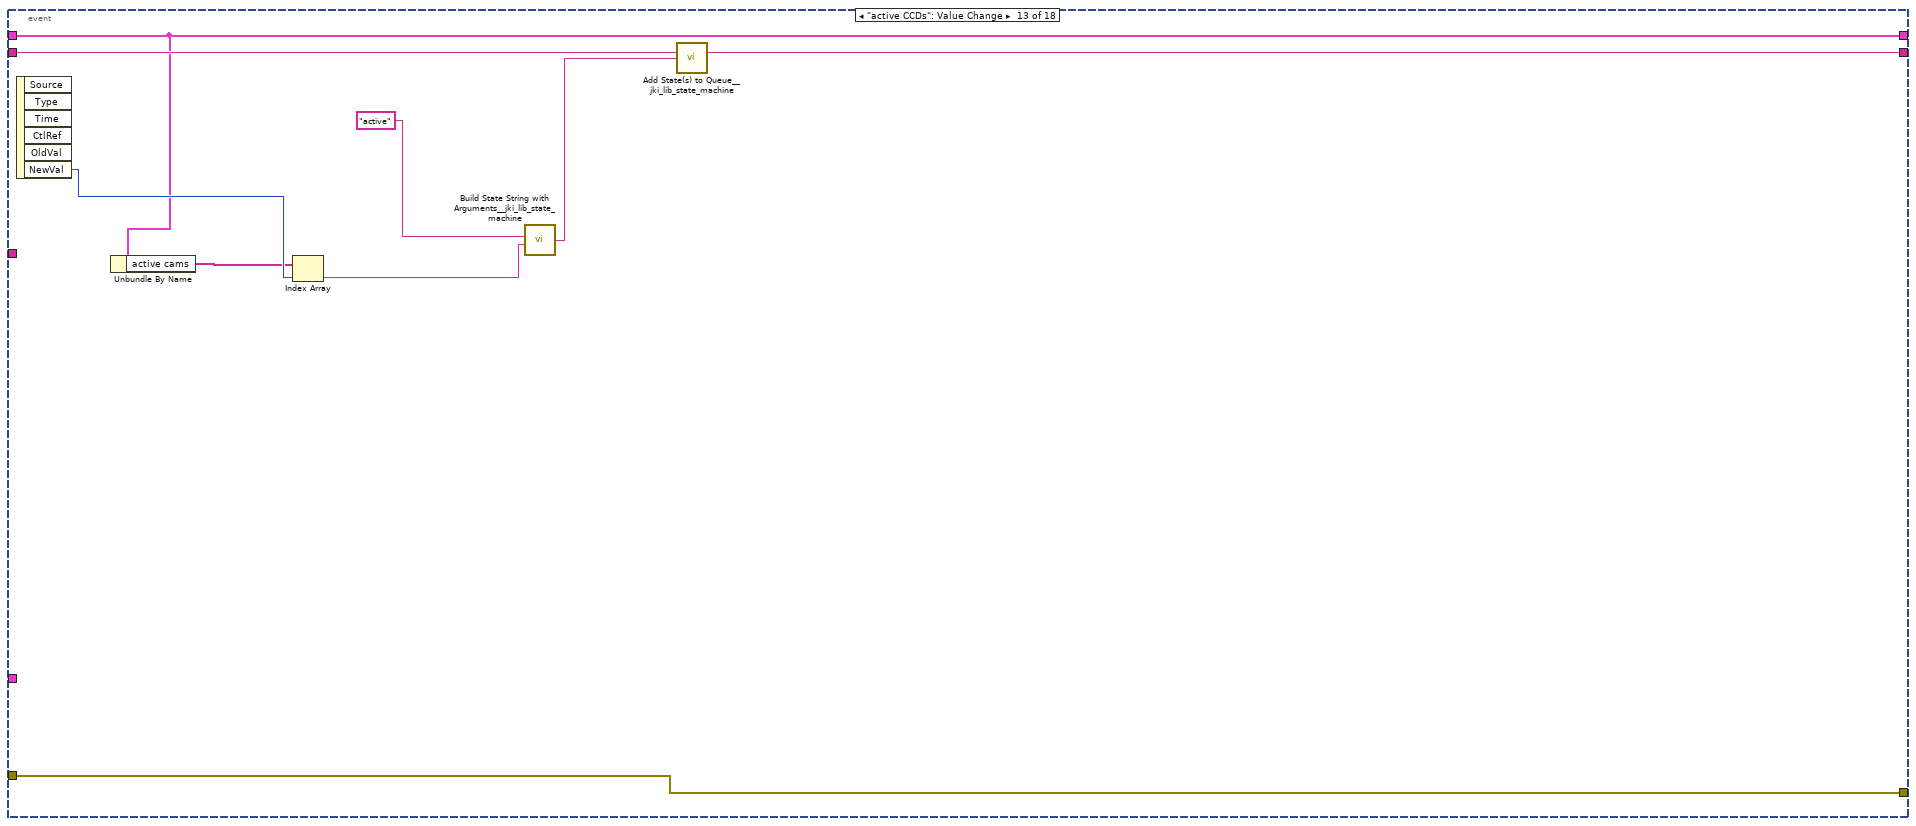
[diagram p19: hidden frame]
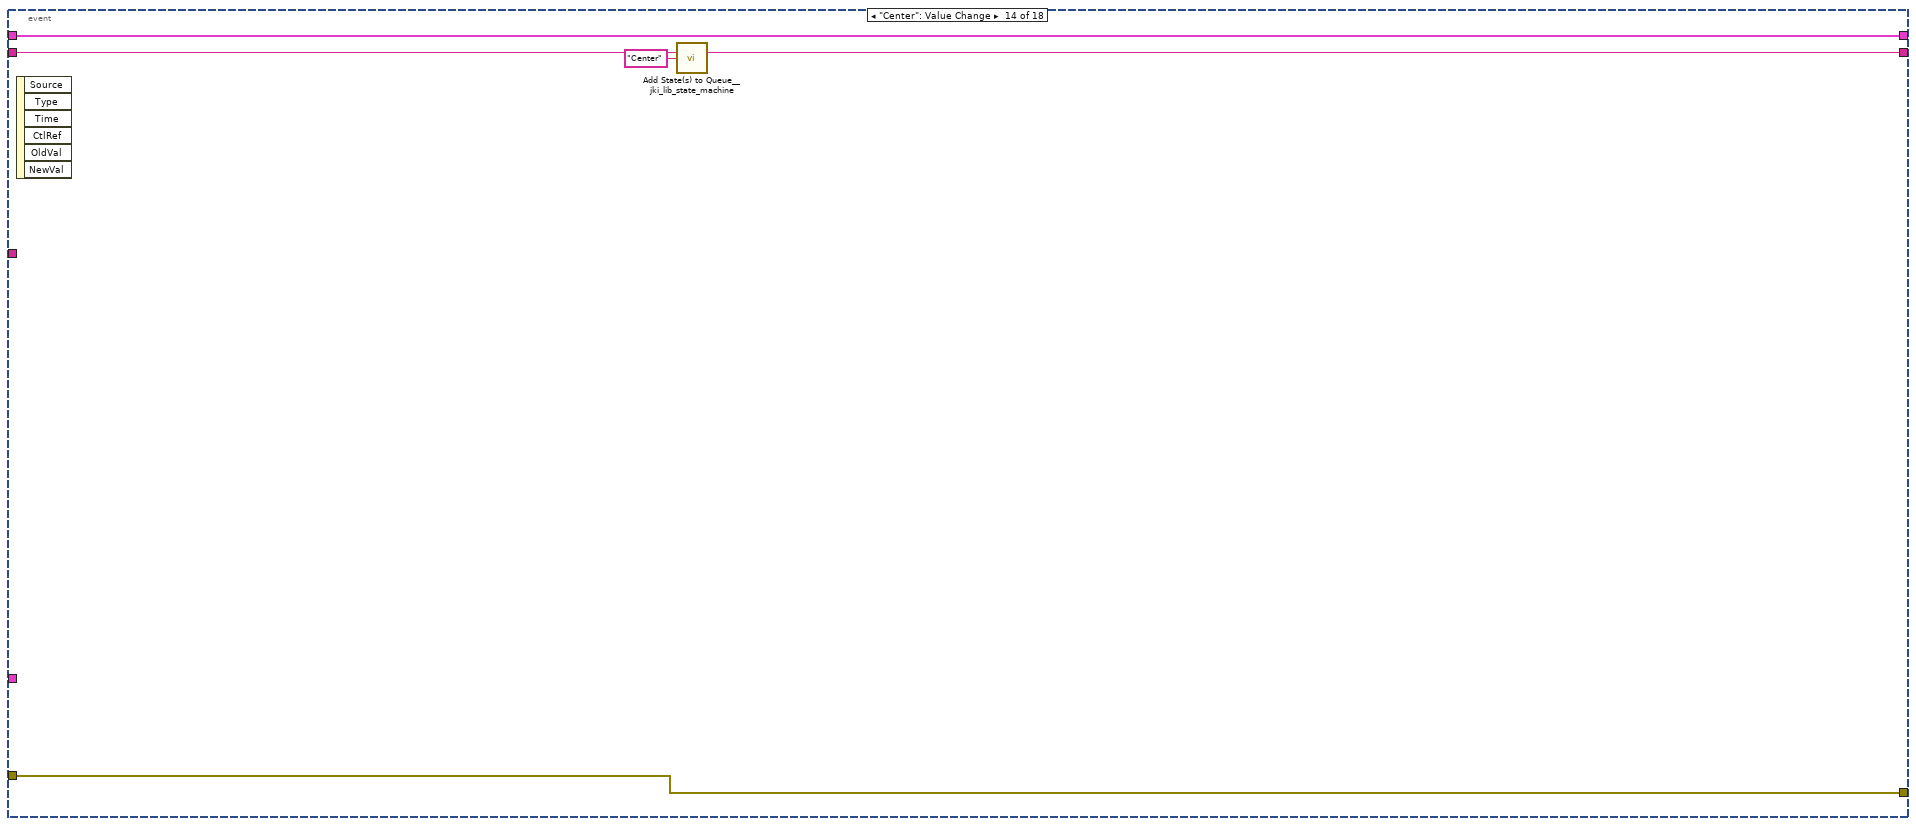
[diagram p20: hidden frame]
diagram:
  n1 = stacked-sequence {
    frame #0 {
      n2 = call <vilib>:"Application Directory.vi"() -> ("Application Directory"=w13:path)
      n3 = Build Path(base path=w13, name or relative path="defaultDevices_PICO.txt") -> (appended path=w15:path)
      "appended path" <- w15
      n4 = call-poly <vilib>:"Read From Spreadsheet File.vi"("file path (dialog if empty)"=w15) -> ("all rows"=w16:string[][])  [unwired: 6 in, 4 out]
      n5 = Index Array(array=w16, index (col) #1=0 ("disabled index (col)"), index (col) #2=1 ("index (col)")) -> (element #1=w19:string[])  [unwired: 2 in, 1 out]
      n6 = Index Array(array=w19, index #1=0 ("index"), index #2=1 ("index"), index #3=2 ("index"), index #4=3 ("index"), index #5=4 ("index"), index #6=5 ("index"), index #7=6 ("index"), index #8=7 ("index"), index #9=8 ("index"), index #10=9 ("index"), index #11=10 ("index"), index #12=11 ("index")) -> (element #1=w12:string, element #2=w11:string, element #3=w10:string, element #4=w9:string, element #5=w8:string, element #6=w7:string, element #7=w6:string, element #8=w5:string, element #9=w4:string, element #10=w3:string, element #11=w2:string, element #12=w1:string)
      n7 = property on="GUIdevice 1" class="Str"("Val(Sgnl)"=w12) -> ()  [unwired: 2 in, 2 out]
      n8 = property on="GUIdevice 2" class="Str"("Val(Sgnl)"=w11) -> ()  [unwired: 2 in, 2 out]
      n9 = property on="GUIdevice 3" class="Str"("Val(Sgnl)"=w10) -> ()  [unwired: 2 in, 2 out]
      n10 = property on="GUIdevice 4" class="Str"("Val(Sgnl)"=w9) -> ()  [unwired: 2 in, 2 out]
      n11 = property on="GUIdevice 5" class="Str"("Val(Sgnl)"=w8) -> ()  [unwired: 2 in, 2 out]
      n12 = property on="GUIdevice 6" class="Str"("Val(Sgnl)"=w7) -> ()  [unwired: 2 in, 2 out]
      n13 = property on="GUIdevice 7" class="Str"("Val(Sgnl)"=w6) -> ()  [unwired: 2 in, 2 out]
      n14 = property on="GUIdevice 8" class="Str"("Val(Sgnl)"=w5) -> ()  [unwired: 2 in, 2 out]
      n15 = property on="GUIdevice 9" class="Str"("Val(Sgnl)"=w4) -> ()  [unwired: 2 in, 2 out]
      n16 = property on="GUIdevice 10" class="Str"("Val(Sgnl)"=w3) -> ()  [unwired: 2 in, 2 out]
      n17 = property on="GUIdevice 11" class="Str"("Val(Sgnl)"=w2) -> ()  [unwired: 2 in, 2 out]
      n18 = property on="GUIdevice 12" class="Str"("Val(Sgnl)"=w1) -> ()  [unwired: 2 in, 2 out]
    }
    frame #1 {
      w104 = T20 1 items=["Grayscale (U8)", "Grayscale (I16)", "Grayscale (SGL)", "Complex (CSG)", "RGB (U32)", "HSL (U32)", "RGB (U64)", "Grayscale (U16)"] ("Image Type")
      # "NOT FOR YOU MOFO"
      n19 = control-ref of="Position.Axis 111::98"() -> (w41:refnum<vi>)
      n20 = control-ref of="Position.Axis 112::98"() -> (w42:refnum<vi>)
      n21 = control-ref of="Position.Axis 113::98"() -> (w43:refnum<vi>)
      n22 = control-ref of="Position.Axis 121::98"() -> (w44:refnum<vi>)
      n23 = control-ref of="Position.Axis 122::98"() -> (w45:refnum<vi>)
      n24 = control-ref of="Position.Axis 123::98"() -> (w46:refnum<vi>)
      n25 = control-ref of="Position.Axis 131::98"() -> (w47:refnum<vi>)
      n26 = control-ref of="Position.Axis 132::98"() -> (w48:refnum<vi>)
      n27 = control-ref of="Position.Axis 133::98"() -> (w49:refnum<vi>)
      n28 = control-ref of="Position.Axis 141::98"() -> (w50:refnum<vi>)
      n29 = control-ref of="Position.Axis 142::98"() -> (w51:refnum<vi>)
      n30 = control-ref of="Position.Axis 143::98"() -> (w52:refnum<vi>)
      n31 = control-ref of="Position.Axis 211::98"() -> (w53:refnum<vi>)
      n32 = control-ref of="Position.Axis 212::98"() -> (w54:refnum<vi>)
      n33 = control-ref of="Position.Axis 213::98"() -> (w55:refnum<vi>)
      n34 = control-ref of="Position.Axis 221::98"() -> (w56:refnum<vi>)
      n35 = control-ref of="Position.Axis 222::98"() -> (w57:refnum<vi>)
      n36 = control-ref of="Position.Axis 223::98"() -> (w58:refnum<vi>)
      n37 = control-ref of="Position.Axis 231::98"() -> (w59:refnum<vi>)
      n38 = control-ref of="Position.Axis 232::98"() -> (w60:refnum<vi>)
      n39 = control-ref of="Position.Axis 233::98"() -> (w61:refnum<vi>)
      n40 = control-ref of="Position.Axis 241::98"() -> (w62:refnum<vi>)
      n41 = control-ref of="Position.Axis 242::98"() -> (w63:refnum<vi>)
      n42 = control-ref of="Position.Axis 243::98"() -> (w64:refnum<vi>)
      n43 = control-ref of="Position.Axis 311::98"() -> (w65:refnum<vi>)
      n44 = control-ref of="Position.Axis 312::98"() -> (w66:refnum<vi>)
      n45 = control-ref of="Position.Axis 313::98"() -> (w67:refnum<vi>)
      n46 = control-ref of="Position.Axis 321::98"() -> (w68:refnum<vi>)
      n47 = control-ref of="Position.Axis 322::98"() -> (w69:refnum<vi>)
      n48 = control-ref of="Position.Axis 323::98"() -> (w70:refnum<vi>)
      n49 = control-ref of="Position.Axis 331::98"() -> (w71:refnum<vi>)
      n50 = control-ref of="Position.Axis 332::98"() -> (w72:refnum<vi>)
      n51 = control-ref of="Position.Axis 333::98"() -> (w73:refnum<vi>)
      n52 = control-ref of="Position.Axis 341::98"() -> (w74:refnum<vi>)
      n53 = control-ref of="Position.Axis 342::98"() -> (w75:refnum<vi>)
      n54 = control-ref of="Position.Axis 343::98"() -> (w76:refnum<vi>)
      n55 = control-ref of="Position.Axis 411::98"() -> (w77:refnum<vi>)
      n56 = control-ref of="Position.Axis 412::98"() -> (w78:refnum<vi>)
      n57 = control-ref of="Position.Axis 413::98"() -> (w79:refnum<vi>)
      n58 = control-ref of="Position.Axis 421::98"() -> (w80:refnum<vi>)
      n59 = control-ref of="Position.Axis 422::98"() -> (w81:refnum<vi>)
      n60 = control-ref of="Position.Axis 423::98"() -> (w82:refnum<vi>)
      n61 = control-ref of="Position.Axis 431::98"() -> (w83:refnum<vi>)
      n62 = control-ref of="Position.Axis 432::98"() -> (w84:refnum<vi>)
      n63 = control-ref of="Position.Axis 433::98"() -> (w85:refnum<vi>)
      n64 = control-ref of="Position.Axis 441::98"() -> (w86:refnum<vi>)
      n65 = control-ref of="Position.Axis 442::98"() -> (w87:refnum<vi>)
      n66 = control-ref of="Position.Axis 443::98"() -> (w88:refnum<vi>)
      n67 = control-ref of="Position.Axis 511::98"() -> (w89:refnum<vi>)
      n68 = control-ref of="Position.Axis 512::98"() -> (w90:refnum<vi>)
      n69 = control-ref of="Position.Axis 513::98"() -> (w91:refnum<vi>)
      n70 = control-ref of="Position.Axis 521::98"() -> (w92:refnum<vi>)
      n71 = control-ref of="Position.Axis 522::98"() -> (w93:refnum<vi>)
      n72 = control-ref of="Position.Axis 523::98"() -> (w94:refnum<vi>)
      n73 = control-ref of="Position.Axis 531::98"() -> (w95:refnum<vi>)
      n74 = control-ref of="Position.Axis 532::98"() -> (w96:refnum<vi>)
      n75 = control-ref of="Position.Axis 533::98"() -> (w97:refnum<vi>)
      n76 = control-ref of="Position.Axis 541::98"() -> (w98:refnum<vi>)
      n77 = control-ref of="Position.Axis 542::98"() -> (w99:refnum<vi>)
      n78 = control-ref of="Position.Axis 543::98"() -> (w100:refnum<vi>)
      n79 = control-ref of="Position.Axis 111::99"() -> (w232:refnum<vi>)
      n80 = control-ref of="Position.Axis 112::99"() -> (w231:refnum<vi>)
      n81 = control-ref of="Position.Axis 113::99"() -> (w230:refnum<vi>)
      n82 = control-ref of="Position.Axis 121::99"() -> (w229:refnum<vi>)
      n83 = control-ref of="Position.Axis 122::99"() -> (w228:refnum<vi>)
      n84 = control-ref of="Position.Axis 123::99"() -> (w227:refnum<vi>)
      n85 = control-ref of="Position.Axis 131::99"() -> (w226:refnum<vi>)
      n86 = control-ref of="Position.Axis 132::99"() -> (w225:refnum<vi>)
      n87 = control-ref of="Position.Axis 133::99"() -> (w224:refnum<vi>)
      n88 = control-ref of="Position.Axis 141::99"() -> (w223:refnum<vi>)
      n89 = control-ref of="Position.Axis 142::99"() -> (w222:refnum<vi>)
      n90 = control-ref of="Position.Axis 143::99"() -> (w221:refnum<vi>)
      n91 = control-ref of="Position.Axis 211::99"() -> (w220:refnum<vi>)
      n92 = control-ref of="Position.Axis 212::99"() -> (w219:refnum<vi>)
      n93 = control-ref of="Position.Axis 213::99"() -> (w218:refnum<vi>)
      n94 = control-ref of="Position.Axis 221::99"() -> (w217:refnum<vi>)
      n95 = control-ref of="Position.Axis 222::99"() -> (w216:refnum<vi>)
      n96 = control-ref of="Position.Axis 223::99"() -> (w215:refnum<vi>)
      n97 = control-ref of="Position.Axis 231::99"() -> (w214:refnum<vi>)
      n98 = control-ref of="Position.Axis 232::99"() -> (w213:refnum<vi>)
      n99 = control-ref of="Position.Axis 233::99"() -> (w212:refnum<vi>)
      n100 = control-ref of="Position.Axis 241::99"() -> (w211:refnum<vi>)
      n101 = control-ref of="Position.Axis 242::99"() -> (w210:refnum<vi>)
      n102 = control-ref of="Position.Axis 243::99"() -> (w209:refnum<vi>)
      n103 = control-ref of="Position.Axis 311::99"() -> (w208:refnum<vi>)
      n104 = control-ref of="Position.Axis 312::99"() -> (w207:refnum<vi>)
      n105 = control-ref of="Position.Axis 313::99"() -> (w206:refnum<vi>)
      n106 = control-ref of="Position.Axis 321::99"() -> (w205:refnum<vi>)
      n107 = control-ref of="Position.Axis 322::99"() -> (w204:refnum<vi>)
      n108 = control-ref of="Position.Axis 323::99"() -> (w203:refnum<vi>)
      n109 = control-ref of="Position.Axis 331::99"() -> (w202:refnum<vi>)
      n110 = control-ref of="Position.Axis 332::99"() -> (w201:refnum<vi>)
      n111 = control-ref of="Position.Axis 333::99"() -> (w200:refnum<vi>)
      n112 = control-ref of="Position.Axis 341::99"() -> (w199:refnum<vi>)
      n113 = control-ref of="Position.Axis 342::99"() -> (w198:refnum<vi>)
      n114 = control-ref of="Position.Axis 343::99"() -> (w197:refnum<vi>)
      n115 = control-ref of="Position.Axis 411::99"() -> (w196:refnum<vi>)
      n116 = control-ref of="Position.Axis 412::99"() -> (w195:refnum<vi>)
      n117 = control-ref of="Position.Axis 413::99"() -> (w194:refnum<vi>)
      n118 = control-ref of="Position.Axis 421::99"() -> (w193:refnum<vi>)
      n119 = control-ref of="Position.Axis 422::99"() -> (w192:refnum<vi>)
      n120 = control-ref of="Position.Axis 423::99"() -> (w191:refnum<vi>)
      n121 = control-ref of="Position.Axis 431::99"() -> (w190:refnum<vi>)
      n122 = control-ref of="Position.Axis 432::99"() -> (w189:refnum<vi>)
      n123 = control-ref of="Position.Axis 433::99"() -> (w188:refnum<vi>)
      n124 = control-ref of="Position.Axis 441::99"() -> (w187:refnum<vi>)
      n125 = control-ref of="Position.Axis 442::99"() -> (w186:refnum<vi>)
      n126 = control-ref of="Position.Axis 443::99"() -> (w185:refnum<vi>)
      n127 = control-ref of="Position.Axis 511::99"() -> (w184:refnum<vi>)
      n128 = control-ref of="Position.Axis 512::99"() -> (w183:refnum<vi>)
      n129 = control-ref of="Position.Axis 513::99"() -> (w182:refnum<vi>)
      n130 = control-ref of="Position.Axis 521::99"() -> (w181:refnum<vi>)
      n131 = control-ref of="Position.Axis 522::99"() -> (w180:refnum<vi>)
      n132 = control-ref of="Position.Axis 523::99"() -> (w179:refnum<vi>)
      n133 = control-ref of="Position.Axis 531::99"() -> (w178:refnum<vi>)
      n134 = control-ref of="Position.Axis 532::99"() -> (w177:refnum<vi>)
      n135 = control-ref of="Position.Axis 533::99"() -> (w176:refnum<vi>)
      n136 = control-ref of="Position.Axis 541::99"() -> (w175:refnum<vi>)
      n137 = control-ref of="Position.Axis 542::99"() -> (w174:refnum<vi>)
      n138 = control-ref of="Position.Axis 543::99"() -> (w173:refnum<vi>)
      n139 = Build Array(w41, w42, w43, w44, w45, w46, w47, w48, w49, w50, w51, w52, w53, w54, w55, w56, w57, w58, w59, w60, w61, w62, w63, w64, w65, w66, w67, w68, w69, w70, w71, w72, w73, w74, w75, w76, w77, w78, w79, w80, w81, w82, w83, w84, w85, w86, w87, w88, w89, w90, w91, w92, w93, w94, w95, w96, w97, w98, w99, w100) -> (w38:refnum<vi>[])
      n140 = Build Array(w232, w231, w230, w229, w228, w227, w226, w225, w224, w223, w222, w221, w220, w219, w218, w217, w216, w215, w214, w213, w212, w211, w210, w209, w208, w207, w206, w205, w204, w203, w202, w201, w200, w199, w198, w197, w196, w195, w194, w193, w192, w191, w190, w189, w188, w187, w186, w185, w184, w183, w182, w181, w180, w179, w178, w177, w176, w175, w174, w173) -> (w37:refnum<vi>[])
      n141 = Build Array (concatenate)(w37, w38) -> (→"motor refs":refnum<vi>[])
      n142 = call "getMotorNames.vi"("DeviceName"="GUIdevice 99") -> ("elements"=w35:string[])  [unwired: 10 in]
      n143 = call "getMotorNames.vi"("DeviceName"="GUIdevice 98") -> ("elements"=w34:string[])  [unwired: 10 in]
      n144 = Build Array (concatenate)(w35, w34) -> (w39:string[])
      "Names" <- w39
      n145 = property on="Motor CCD 1" class="Ring (strict)"("Strings []"=w39) -> ()  [unwired: 2 in, 2 out]
      n146 = property on="Motor CCD 2" class="Ring (strict)"("Strings []"=w39) -> ()  [unwired: 2 in, 2 out]
      n147 = property on="Motor CCD 3" class="Ring (strict)"("Strings []"=w39) -> ()  [unwired: 2 in, 2 out]
      n148 = property on="Motor CCD 4" class="Ring (strict)"("Strings []"=w39) -> ()  [unwired: 2 in, 2 out]
      n149 = property on="Motor CCD 5" class="Ring (strict)"("Strings []"=w39) -> ()  [unwired: 2 in, 2 out]
      n150 = property on="Motor CCD 6" class="Ring (strict)"("Strings []"=w39) -> ()  [unwired: 2 in, 2 out]
      n151 = property on="Motor CCD 7" class="Ring (strict)"("Strings []"=w39) -> ()  [unwired: 2 in, 2 out]
      n152 = property on="Motor CCD 8" class="Ring (strict)"("Strings []"=w39) -> ()  [unwired: 2 in, 2 out]
      n153 = property on="Motor CCD 9" class="Ring (strict)"("Strings []"=w39) -> ()  [unwired: 2 in, 2 out]
      n154 = property on="Motor CCD 10" class="Ring (strict)"("Strings []"=w39) -> ()  [unwired: 2 in, 2 out]
      n155 = property on="Motor CCD 11" class="Ring (strict)"("Strings []"=w39) -> ()  [unwired: 2 in, 2 out]
      n156 = property on="Motor CCD 12" class="Ring (strict)"("Strings []"=w39) -> ()  [unwired: 2 in, 2 out]
      n157 = property on="ActiveMotor" class="Ring (strict)"("Strings []"=w35) -> ()  [unwired: 2 in, 2 out]
      n158 = control-ref of="Target.X::1"() -> (w159:refnum<vi>)
      n159 = control-ref of="Target.Y::1"() -> (w158:refnum<vi>)
      n160 = control-ref of="Target.X::2"() -> (w157:refnum<vi>)
      n161 = control-ref of="Target.Y::2"() -> (w156:refnum<vi>)
      n162 = control-ref of="Target.X::3"() -> (w155:refnum<vi>)
      n163 = control-ref of="Target.Y::3"() -> (w154:refnum<vi>)
      n164 = control-ref of="Target.X::4"() -> (w153:refnum<vi>)
      n165 = control-ref of="Target.Y::4"() -> (w152:refnum<vi>)
      n166 = control-ref of="Target.X::5"() -> (w151:refnum<vi>)
      n167 = control-ref of="Target.Y::5"() -> (w150:refnum<vi>)
      n168 = control-ref of="Target.X::6"() -> (w149:refnum<vi>)
      n169 = control-ref of="Target.Y::6"() -> (w148:refnum<vi>)
      n170 = control-ref of="Target.X::7"() -> (w147:refnum<vi>)
      n171 = control-ref of="Target.Y::7"() -> (w146:refnum<vi>)
      n172 = control-ref of="Target.X::8"() -> (w145:refnum<vi>)
      n173 = control-ref of="Target.Y::8"() -> (w144:refnum<vi>)
      n174 = control-ref of="Target.X::9"() -> (w121:refnum<vi>)
      n175 = control-ref of="Target.Y::9"() -> (w120:refnum<vi>)
      n176 = control-ref of="Target.X::10"() -> (w119:refnum<vi>)
      n177 = control-ref of="Target.Y::10"() -> (w118:refnum<vi>)
      n178 = control-ref of="Target.X::11"() -> (w117:refnum<vi>)
      n179 = control-ref of="Target.Y::11"() -> (w116:refnum<vi>)
      n180 = control-ref of="Target.X::12"() -> (w115:refnum<vi>)
      n181 = control-ref of="Target.Y::12"() -> (w114:refnum<vi>)
      n182 = call "IMAQ Create"("Image Name"="GUIdevice 8", "Image Type"=w104) -> ("New Image"=→"image::8":T9)  [unwired: 3 in, 1 out]
      n183 = call "IMAQ Create"("Image Name"="GUIdevice 9", "Image Type"=w104) -> ("New Image"=→"image::9":T9)  [unwired: 3 in, 1 out]
      n184 = call "IMAQ Create"("Image Name"="GUIdevice 10", "Image Type"=w104) -> ("New Image"=→"image::10":T9)  [unwired: 3 in, 1 out]
      n185 = call "IMAQ Create"("Image Name"="GUIdevice 6", "Image Type"=w104) -> ("New Image"=→"image::6":T9)  [unwired: 3 in, 1 out]
      n186 = call "IMAQ Create"("Image Name"="GUIdevice 7", "Image Type"=w104) -> ("New Image"=→"image::7":T9)  [unwired: 3 in, 1 out]
      n187 = call "IMAQ Create"("Image Name"="GUIdevice 11", "Image Type"=w104) -> ("New Image"=→"image::11":T9)  [unwired: 3 in, 1 out]
      n188 = call "IMAQ Create"("Image Name"="GUIdevice 12", "Image Type"=w104) -> ("New Image"=→"image::12":T9)  [unwired: 3 in, 1 out]
      n189 = call "IMAQ Create"("Image Name"="GUIdevice 2") -> ("New Image"=→"image::2":T9)  [unwired: 4 in, 1 out]
      n190 = call "IMAQ Create"("Image Name"="GUIdevice 4", "Image Type"=w104) -> ("New Image"=→"image::4":T9)  [unwired: 3 in, 1 out]
      n191 = call "IMAQ Create"("Image Name"="GUIdevice 1", "Image Type"=w104) -> ("New Image"=→"image::1":T9)  [unwired: 3 in, 1 out]
      n192 = call "IMAQ Create"("Image Name"="GUIdevice 3", "Image Type"=w104) -> ("New Image"=→"image::3":T9)  [unwired: 3 in, 1 out]
      n193 = call "IMAQ Create"("Image Name"="GUIdevice 5", "Image Type"=w104) -> ("New Image"=→"image::5":T9)  [unwired: 3 in, 1 out]
      n194 = Build Array("GUIdevice 1", "GUIdevice 2", "GUIdevice 3", "GUIdevice 4", "GUIdevice 5", "GUIdevice 6", "GUIdevice 7", "GUIdevice 8", "GUIdevice 9", "GUIdevice 10", "GUIdevice 11", "GUIdevice 12") -> (w133:string[])
      "CCDs" <- w133
      n195 = property on="image::8" class="ImageControl"("Caption.Text"="GUIdevice 8") -> ()  [unwired: 2 in, 2 out]
      n196 = property on="image::10" class="ImageControl"("Caption.Text"="GUIdevice 10") -> ()  [unwired: 2 in, 2 out]
      n197 = property on="image::9" class="ImageControl"("Caption.Text"="GUIdevice 9") -> ()  [unwired: 2 in, 2 out]
      n198 = property on="image::1" class="ImageControl"("Caption.Text"="GUIdevice 1") -> ()  [unwired: 2 in, 2 out]
      n199 = property on="image::2" class="ImageControl"("Caption.Text"="GUIdevice 2") -> ()  [unwired: 2 in, 2 out]
      n200 = property on="image::3" class="ImageControl"("Caption.Text"="GUIdevice 3") -> ()  [unwired: 2 in, 2 out]
      n201 = property on="image::4" class="ImageControl"("Caption.Text"="GUIdevice 4") -> ()  [unwired: 2 in, 2 out]
      n202 = property on="image::5" class="ImageControl"("Caption.Text"="GUIdevice 5") -> ()  [unwired: 2 in, 2 out]
      n203 = property on="image::6" class="ImageControl"("Caption.Text"="GUIdevice 6") -> ()  [unwired: 2 in, 2 out]
      n204 = property on="image::7" class="ImageControl"("Caption.Text"="GUIdevice 7") -> ()  [unwired: 2 in, 2 out]
      n205 = property on="image::11" class="ImageControl"("Caption.Text"="GUIdevice 11") -> ()  [unwired: 2 in, 2 out]
      n206 = property on="image::12" class="ImageControl"("Caption.Text"="GUIdevice 12") -> ()  [unwired: 2 in, 2 out]
      n207 = Array To Cluster(array=w133) -> (cluster=→"Cameras":T21)
      n208 = Bundle("Target.X::1"=w159, "Target.Y::1"=w158) -> (w143:T22)  [unwired: 1 in]
      n209 = Bundle("Target.X::2"=w157, "Target.Y::2"=w156) -> (w142:T23)  [unwired: 1 in]
      n210 = Bundle("Target.X::3"=w155, "Target.Y::3"=w154) -> (w141:T24)  [unwired: 1 in]
      n211 = Bundle("Target.X::4"=w153, "Target.Y::4"=w152) -> (w134:T25)  [unwired: 1 in]
      n212 = Bundle("Target.X::5"=w151, "Target.Y::5"=w150) -> (w140:T26)  [unwired: 1 in]
      n213 = Bundle("Target.X::6"=w149, "Target.Y::6"=w148) -> (w139:T27)  [unwired: 1 in]
      n214 = Bundle("Target.X::7"=w147, "Target.Y::7"=w146) -> (w138:T28)  [unwired: 1 in]
      n215 = Bundle("Target.X::8"=w145, "Target.Y::8"=w144) -> (w137:T29)  [unwired: 1 in]
      n216 = Bundle("Target.X::12"=w115, "Target.Y::12"=w114) -> (w110:T30)  [unwired: 1 in]
      n217 = Bundle("Target.X::9"=w121, "Target.Y::9"=w120) -> (w113:T31)  [unwired: 1 in]
      n218 = Bundle("Target.X::10"=w119, "Target.Y::10"=w118) -> (w112:T32)  [unwired: 1 in]
      n219 = Bundle("Target.X::11"=w117, "Target.Y::11"=w116) -> (w111:T33)  [unwired: 1 in]
      n220 = property on="CCDs" class="Ring (strict)"("Strings []"=w133) -> ()  [unwired: 2 in, 2 out]
      n221 = Build Array(w143, w142, w141, w134, w140, w139, w138, w137, w113, w112, w111, w110) -> (w136:T34)
      n222 = Tick Count (ms)() -> (millisecond timer value=→"millisecond timer value":u32)
      n223 = property on="Feedback Global" class="Bool (strict)"("Value"=FALSE ("Feedback Global")) -> ()  [unwired: 2 in, 2 out]
      n224 = Get Date/Time In Seconds() -> (seconds since 1Jan1904=w123:timestamp)
      n225 = Format Date/Time String(time format string (%c)="%Y%m%d%H%M", seconds (now)=w123) -> (date/time string=w122:string)  [unwired: 1 in]
      n226 = Concatenate Strings(w122, "Beampointing_Pico.tdms" ("string")) -> (w126:string)
      n227 = String To Path(string=w126) -> (path=w125:path)
      n228 = Build Path(base path=path "w:/BP_DATA", name or relative path=w125) -> (appended path=w128:path)
      n229 = call <vilib>:"Add State(s) to Queue__jki_lib_state_machine.vi"("State(s) in (\"\")"="Macro: Initialize") -> ("States Out"=w234:string)  [unwired: 14 in]
      n230 = Create User Event(user event datatype=T14 {"EventEnum"=enum."new data", "Device name"="Device name"} ("New Event")) -> (user event=w242:refnum<user-event>, error out=w244:errorcluster)  [unwired: 1 in]
      "tcp data event" <- w242
      n231 = while "JKI - String-Based Queued State Machine (Basic) v1.0" {
        shift-right: [w266] -> w132
        shift-left: _ -> [w254]
        shift-right: [w269] -> w160
        shift-left: _ -> [w265]
        shift-right: [w268] -> _
        shift-left: w234 -> [w270]
        tunnel: w136 -> [w263]
        tunnel: w133 -> [w261]
        tunnel: [w261] -> w161
        tunnel: w136 -> [w262]
        tunnel: w128 -> [w252]
        stop <- w267 stop-if-true
        n232 = Unbundle By Name(w254) -> ("active cams"=w253:string[])
        n233 = call <vilib>:"Parse State Queue__jki_lib_state_machine.vi"("State Queue"=w270, "Error In (no error)"=w265) -> ("Remaining States"=w272:string, "Current State"=w273:string, "Arguments"=w271:string)  [unwired: 11 in]
        "Current State" <- w273
        n234 = case shown="\"\", \"Idle\"" w273 {
          selector: w273 -> [_ _ w559 _ _ _ _ _ _ _ _ _ _ _ _ _ _ _ _ _ _ _ _ _ _ _ _ _ _ _ _ _ _ _ _ _ _ _ _ _]
          tunnel: w272 -> [w302 w558 w563 w581 w587 w592 w596 w638 w646 w650 w654 w660 w671 w695 w705 w715 w719 w737 w839 w891 w904 w913 w940 w961 w965 w984 w1123 w1277 w1368 w1434 w1472 w1492 w1507 w1595 w1647 w1657 w1664 w1687 w1707 w1734]
          tunnel: w271 -> [_ _ _ _ _ _ _ _ _ _ _ w655 w666 _ _ _ _ w732 w790 _ w901 _ _ _ _ w986 _ w1255 w1345 _ _ _ _ _ _ _ w1661 _ _ _]
          tunnel: w254 -> [w300 w555 w561 w571 w584 w590 w593 _ w642 w647 w652 w658 w665 w692 w703 w707 w716 w729 w791 w889 w896 w909 w932 w954 w962 w968 w1117 w1270 w1361 w1431 w1443 w1489 w1504 w1567 w1644 w1654 w1660 w1673 w1704 w1725]
          tunnel: [w299 w556 w565 w579 errorcluster {"status"=FALSE, "code"=0, "source"=""} ("error out") w589 w594 w606 w639 w648 w651 w656 w668 w693 w704 w713 w717 w733 w795 w880 w902 w911 w938 w959 w963 w988 w1147 w1275 w1366 w1432 w1470 w1490 w1505 w1585 w1645 w1655 w1662 w1665 w1705 w1732] -> w269
          tunnel: w265 -> [w298 w556 w564 w579 w583 w589 w594 w613 w644 w648 w651 w657 w669 w693 w704 w713 w717 w733 w793 w881 w902 w911 w938 w959 w963 w988 w1147 w1275 w1366 w1432 w1470 w1490 w1505 w1590 w1645 w1655 w1662 w1671 w1705 w1732]
          tunnel: [w301 w557 w562 w580 w586 w591 w595 w637 w645 w649 w653 w659 w670 w694 w696 w714 w718 w720 w838 w890 w903 w912 w939 w960 w964 w991 w1148 w1276 w1367 w1433 w1471 w1491 w1506 w1555 w1646 w1656 w1663 w1686 w1706 w1733] -> w268
          tunnel: [_ _ _ _ _ TRUE _ _ _ _ _ _ _ _ _ _ _ _ _ _ _ _ _ _ _ _ _ _ _ _ _ _ _ _ _ _ _ _ _ _] -> w267
          tunnel: [w295 w555 w561 w570 w584 w590 w593 w598 w642 w647 w652 w658 w665 w692 w703 w707 w716 w734 w828 w889 w895 w908 w931 w953 w962 w1013 w1116 w1270 w1361 w1430 w1443 w1489 w1504 w1567 w1643 w1654 w1659 w1674 w1704 w1724] -> w266
          tunnel: "update speed [ms]" -> [w297 _ _ _ _ _ _ _ _ _ _ _ _ _ _ _ _ _ _ _ _ _ _ _ _ _ _ _ _ _ _ _ _ _ _ _ _ _ _ _]
          tunnel: w263 -> [w294 _ _ _ _ _ _ _ _ _ _ _ _ _ _ _ _ _ _ _ _ _ _ _ _ w1011 _ _ _ _ _ _ _ _ _ _ _ _ w1688 _]
          tunnel: w261 -> [w296 _ _ _ _ _ _ w604 _ _ _ _ _ _ _ _ _ w736 w792 _ w897 _ _ _ _ w976 w1113 w1274 w1365 _ w1444 _ w1493 w1593 _ _ _ w1668 _ _]
          tunnel: w252 -> [_ _ _ _ _ _ _ w611 _ _ _ _ _ _ _ _ _ _ _ _ _ _ _ _ _ _ _ _ _ _ _ _ _ _ _ _ _ _ _ _]
          frame "", "Idle" {
            # "executes when the state queue is empty"
            n235 = event shown="[0] Timeout" {
              selector: _ -> [_ _ _ _ _ _ _ _ _ _ _ _ _ _ _ _ _ _]
              dyn-events: _ -> [_ _ _ _ _ _ _ _ _ _ _ _ _ _ _ _ _ _]
              timeout: w297 -> [_ _ _ _ _ _ _ _ _ _ _ _ _ _ _ _ _ _]
              tunnel: w302 -> [w305 w432 w447 w466 w471 w476 w481 w487 w494 w499 w509 w514 w523 w528 w534 w540 w548 w554]
              tunnel: [w320 w431 w446 w465 w470 w475 w480 w486 w493 w498 w508 w513 w522 w527 w533 w539 w547 w553] -> w301
              tunnel: w300 -> [w310 w429 w443 w462 w468 w473 w478 w484 w491 w496 w506 w511 w516 w525 w531 w537 w545 w551]
              tunnel: [w314 w430 w445 w464 w469 w474 w479 w485 w492 w497 w507 w512 w521 w526 w532 w538 w546 w552] -> w299
              tunnel: w298 -> [w317 w430 w445 w464 w469 w474 w479 w485 w492 w497 w507 w512 w521 w526 w532 w538 w546 w552]
              tunnel: [w319 w429 w443 w461 w468 w473 w478 w484 w491 w496 w506 w511 w516 w525 w531 w537 w545 w551] -> w295
              tunnel: w296 -> [w337 _ w439 _ _ _ _ _ _ _ _ _ _ _ _ _ _ _]
              tunnel: w294 -> [_ _ w441 _ _ _ _ _ _ _ _ _ _ _ _ _ _ _]
              event Timeout {
                n236 = event-data() -> ()  [unwired: 1 in, 1 out]
                n237 = Unbundle By Name(w310) -> ("Centroid X"=w307:dbl[][], "Centroid Y"=w347:dbl[][], "Size"=w340:dbl[][], "detection para"=w336:T3[], "active cams"=w331:string[], "thresholds"=w328:cluster{"Lower value":sgl, "Upper value":sgl}[])
                n238 = Unbundle By Name(w310) -> ("active ccd"=w309:i32)
                n239 = call <userlib>:"Tick Count (ms)__ogtk.vi"("error in (no error)"=w317) -> ("error out"=w316:errorcluster, "millisecond timer value"=→"millisecond timer 2":u32)  [unwired: 9 in]
                n240 = for {
                  N: 12 ("Numeric 2") -> [_]
                  tunnel: w331 -> [w392] mode=indexing
                  tunnel: [w393] -> w345 mode=indexing
                  tunnel: w337 -> [w416]
                  tunnel: w336 -> [w414]
                  tunnel: [w412] -> w313 mode=indexing
                  tunnel: [w411] -> w311 mode=indexing
                  tunnel: [w409] -> w332 mode=indexing
                  tunnel: "autodetect" -> [w403]
                  tunnel: w316 -> [w417]
                  tunnel: [w418] -> w338
                  shift-right: [w400] -> w308
                  shift-left: w328 -> [w402]
                  shift-right: [w387] -> w346
                  shift-left: w307 -> [w389]
                  shift-right: [w383] -> w348
                  shift-left: w347 -> [w385]
                  shift-right: [w377] -> w339
                  shift-left: w340 -> [w379]
                  w381 = 0 ("index")
                  n241 = call-poly <userlib>:"Filter 1D Array__ogtk.vi"("items to filter"=w392, "array"=w416) -> ("filtered item indices"=w415:i32[])  [unwired: 4 in, 1 out]
                  n242 = Index Array(array=w415) -> (element=w378:i32)  [unwired: 1 in]
                  n243 = Index Array(array=w379, index (row)=w378) -> (element=w407:dbl[])  [unwired: 1 in]
                  n244 = Index Array(array=w385, index (row)=w378) -> (element=w408:dbl[])  [unwired: 1 in]
                  n245 = Index Array(array=w402, index=w378) -> (element=w406:cluster{"Lower value":sgl, "Upper value":sgl})
                  n246 = Index Array(array=w389, index (row)=w378) -> (element=w391:dbl[])  [unwired: 1 in]
                  n247 = Index Array(array=w414, index=w378) -> (element=w410:T3)
                  n248 = call "CENTRIOD DETECTION.vi"("Refnum in"=w392, "auto threshold"=w403, "Threshold Range In"=w406, "beam detection para"=w410, "error in (no error)"=w417) -> ("Bounding Rect"=w409:T35, "Particle Reports (Pixels)"=w411:T1, "Threshold Range Out"=w401:cluster{"Lower value":sgl, "Upper value":sgl}, "Centriod"=w419:cluster{"X":dbl, "Y":dbl}, "error out"=w418:errorcluster)  [unwired: 7 in, 3 out]
                  n249 = Unbundle By Name(w419) -> ("X"=w390:dbl, "Y"=w386:dbl)
                  n250 = Empty Array?(array=w411) -> (empty?=w413:bool)
                  n251 = Not(x=w413) -> (.not. x?=w412:bool)
                  n252 = Replace Array Subset(array=w402, new element=w401, index=w378) -> (w400:cluster{"Lower value":sgl, "Upper value":sgl}[])
                  n253 = Unbundle By Name(w409) -> ("Right"=w399:dbl, "Left"=w398:dbl, "Bottom"=w397:dbl, "Top"=w396:dbl)
                  n254 = Subtract(x=w399, y=w398) -> (x-y=w394:dbl)
                  n255 = Subtract(x=w397, y=w396) -> (x-y=w395:dbl)
                  n256 = Multiply(x=w394, y=w395) -> (x*y=w382:dbl)
                  n257 = Insert Into Array(array=w408, index=w381, new element=w386) -> (w384:dbl[])
                  n258 = Insert Into Array(array=w407, index=w381, new element=w382) -> (w380:dbl[])
                  n259 = Insert Into Array(array=w391, index=w381, new element=w390) -> (w388:dbl[])
                  n260 = for {
                    shift-right: [w420] -> w404
                    shift-left: dbl[] [] ("Array 4") -> [w423]
                    tunnel: w384 -> [w421] mode=indexing
                    n261 = Equal To 0?(x=w421) -> (x = 0?=w422:bool)
                    n262 = case shown="False" w422 {
                      tunnel: w423 -> [w426 w427]
                      tunnel: w421 -> [w425 _]
                      tunnel: [w424 w427] -> w420
                      frame False {
                        n263 = Build Array (concatenate)(w426, w425) -> (w424:dbl[])
                      }
                      frame True {
                      }
                    }
                  }
                  n264 = Replace Array Subset(array=w389, new element=w388, index (row)=w378) -> (w387:dbl[][])  [unwired: 1 in]
                  n265 = Replace Array Subset(array=w385, new element=w384, index (row)=w378) -> (w383:dbl[][])  [unwired: 1 in]
                  n266 = Replace Array Subset(array=w379, new element=w380, index (row)=w378) -> (w377:dbl[][])  [unwired: 1 in]
                  n267 = Array Size(array=w404) -> (size(s)=w393:i32)
                }
                "detected" <- w313
                "Particle Reports (Pixels)" <- w311
                "Box" <- w332
                n268 = Bundle(0, 1, "Centroid X"=w307) -> (→"Status":cluster{i32, i32, "Centroid X":dbl[][]})  [unwired: 1 in]
                n269 = Index Array(array=w311, index (row)=w309) -> (element=→"particles":T1)  [unwired: 1 in]
                n270 = call <vilib>:"Clear Errors.vi"("error in (no error)"=w338) -> ("error out"=w314:errorcluster)  [unwired: 6 in]
                n271 = local read "Img to avg"() -> (w322:i32)
                n272 = local read "Numeric"() -> (w325:dbl)
                n273 = Increment(x=w322) -> (x+1=w321:i32)
                n274 = Greater Or Equal?(x=w325, y=w321) -> (x >= y?=w318:bool)
                n275 = Increment(x=w325) -> (x+1=w324:dbl)
                n276 = Select(t=0.0, s=w318, f=w324) -> (s? t:f=w323:dbl)
                n277 = local write "Numeric"(w323) -> ()
                n278 = for {
                  tunnel: w345 -> [w369] mode=indexing
                  tunnel: w331 -> [w376] mode=indexing
                  shift-right: [w371] -> w341
                  shift-left: "" ("GUIdevice 7") -> [w374]
                  tunnel: [w364] -> w343 mode=indexing
                  tunnel: "Detection Rate" -> [w368]
                  tunnel: w323 -> [w366]
                  n279 = local read "Img to avg"() -> (w370:i32)
                  n280 = Greater Or Equal?(x=w369, y=w370) -> (x >= y?=w365:bool)
                  n281 = Multiply(x=w368, y=w366) -> (x*y=w367:dbl)
                  n282 = Greater Or Equal?(x=w369, y=w367) -> (x >= y?=w363:bool)
                  n283 = And(x=w365, y=w363) -> (x .and. y?=w364:bool)
                  n284 = Select(t=w376, s=w364, f="") -> (s? t:f=w372:string)
                  n285 = Concatenate Strings(w374, "\t", w372) -> (w371:string)
                }
                n286 = Bundle By Name(cluster=w310, "thresholds"=w308, "detected"=w313) -> (w329:T36)
                n287 = Bundle By Name(cluster=w329, "Centroid X"=w346, "Centroid Y"=w348, "Size"=w339) -> (w304:T36)
                n288 = Unbundle By Name(w304) -> ("img to avg"=w303:i32)
                n289 = Or Array Elements(Boolean array=w343) -> (logical OR=w342:bool)
                n290 = case shown="True" w318 {
                  tunnel: w304 -> [w349 w356]
                  tunnel: [w349 w355] -> w319
                  tunnel: w303 -> [_ w351]
                  frame False {
                  }
                  frame True {
                    n291 = Decrement(x=w351) -> (x-1=w350:i32)
                    n292 = Initialize Array(0.0 ("element"), 12 ("dimension size"), w350) -> (w352:dbl[][])
                    n293 = Bundle By Name(cluster=w356, "Centroid X"=w352, "Centroid Y"=w352, "Size"=w352) -> (w355:T36)
                  }
                }
                n294 = case shown="True" w342 {
                  tunnel: w341 -> [_ w361]
                  tunnel: w305 -> [w357 w359]
                  tunnel: [w357 w358] -> w320
                  frame False {
                  }
                  frame True {
                    n295 = call <vilib>:"Build State String with Arguments__jki_lib_state_machine.vi"("Arguments (\"\")"=w361, "State"="detected") -> ("State with Arguments"=w360:string)  [unwired: 4 in]
                    n296 = call <vilib>:"Add State(s) to Queue__jki_lib_state_machine.vi"("State(s) in (\"\")"=w359, "State(s) at Back (\"\")"=w360) -> ("States Out"=w358:string)  [unwired: 13 in]
                  }
                }
              }
              event "stop": Value Change {
                # "Exit Button Value Change (pressed) Event\n(this executes Macro: Exit to terminate the VI)"
                n297 = event-data() -> ()  [unwired: 1 in, 6 out]
                n298 = call <vilib>:"Add State(s) to Queue__jki_lib_state_machine.vi"("State(s) in Front (\"\")"="Macro: Exit", "State(s) in (\"\")"=w432) -> ("States Out"=w431:string)  [unwired: 13 in]
              }
              event Value Change {
                n299 = event-data() -> ()  [unwired: 1 in, 6 out]
                n300 = property on="Set Centriod Target" class="Bool (strict)"("Value"=FALSE) -> ()  [unwired: 2 in, 2 out]
                n301 = Unbundle By Name(w443) -> ("active ccd"=w435:i32, "Centroid X"=w434:dbl[][], "Centroid Y"=w433:dbl[][])
                n302 = Index Array(array=w439, index=w435) -> (element=w438:string)
                n303 = Concatenate Strings("Do want to update the target of " ("message"), w438, "?" ("string")) -> (w436:string)
                n304 = Two Button Dialog(message=w436) -> (T button?=w442:bool)  [unwired: 2 in]
                n305 = case shown="True" w442 {
                  tunnel: w441 -> [_ w454]
                  tunnel: w435 -> [_ w453]
                  tunnel: w434 -> [_ w460]
                  tunnel: w433 -> [_ w455]
                  frame False {
                  }
                  frame True {
                    n306 = Index Array(array=w460, index (row)=w453) -> (element=w459:dbl[])  [unwired: 1 in]
                    n307 = Index Array(array=w455, index (row)=w453) -> (element=w456:dbl[])  [unwired: 1 in]
                    n308 = Index Array(array=w454, index=w453) -> (element=w452:T30)
                    n309 = Unbundle By Name(w452) -> ("Target.X::12"=w451:refnum<vi>, "Target.Y::12"=w449:refnum<vi>)
                    n310 = Reverse 1D Array(array=w459) -> (reversed array=w458:dbl[])
                    n311 = Reverse 1D Array(array=w456) -> (reversed array=w457:dbl[])
                    n312 = Index Array(array=w458) -> (element=w450:dbl)  [unwired: 1 in]
                    n313 = Index Array(array=w457) -> (element=w448:dbl)  [unwired: 1 in]
                    n314 = property class="DigNum (strict)"(reference=w451, "Val(Sgnl)"=w450) -> ()  [unwired: 1 in, 2 out]
                    n315 = property class="DigNum (strict)"(reference=w449, "Val(Sgnl)"=w448) -> ()  [unwired: 1 in, 2 out]
                  }
                }
                n316 = call <vilib>:"Add State(s) to Queue__jki_lib_state_machine.vi"("State(s) in (\"\")"=w447) -> ("States Out"=w446:string)  [unwired: 14 in]
              }
              event "Feedback Global": Value Change {
                # "Exit Button Value Change (pressed) Event\n(this executes Macro: Exit to terminate the VI)"
                n317 = event-data() -> ("NewVal"=w463:bool)  [unwired: 1 in, 5 out]
                n318 = call <vilib>:"Add State(s) to Queue__jki_lib_state_machine.vi"("State(s) in (\"\")"=w466) -> ("States Out"=w465:string)  [unwired: 14 in]
                n319 = Bundle By Name(cluster=w462, "Feedback global"=w463) -> (w461:T36)
              }
              event Value Change {
                n320 = event-data() -> ()  [unwired: 1 in, 6 out]
                n321 = call <vilib>:"Add State(s) to Queue__jki_lib_state_machine.vi"("State(s) in Front (\"\")"="Move Config", "State(s) in (\"\")"=w471) -> ("States Out"=w470:string)  [unwired: 13 in]
              }
              event Value Change {
                n322 = event-data() -> ()  [unwired: 1 in, 6 out]
                n323 = call <vilib>:"Add State(s) to Queue__jki_lib_state_machine.vi"("State(s) in Front (\"\")"="Detection Config", "State(s) in (\"\")"=w476) -> ("States Out"=w475:string)  [unwired: 13 in]
              }
              event "associated motors": Value Change {
                n324 = event-data() -> ()  [unwired: 1 in, 6 out]
                n325 = call <vilib>:"Add State(s) to Queue__jki_lib_state_machine.vi"("State(s) in (\"\")"=w481, "State(s) at Back (\"\")"="Motor Config" ("State(s) at Back (\"\")")) -> ("States Out"=w480:string)  [unwired: 13 in]
              }
              event "Reset History": Value Change {
                n326 = event-data() -> ()  [unwired: 1 in, 6 out]
                n327 = call <vilib>:"Add State(s) to Queue__jki_lib_state_machine.vi"("State(s) in (\"\")"=w487, "State(s) at Back (\"\")"="Reset History" ("State(s) at Back (\"\")")) -> ("States Out"=w486:string)  [unwired: 13 in]
                n328 = property on="Reset History" class="Bool (strict)"("Value"=FALSE ("Reset History")) -> ()  [unwired: 2 in, 2 out]
              }
              event "ActiveMotor": Value Change {
                n329 = event-data() -> ("NewVal"=w489:u16)  [unwired: 1 in, 5 out]
                n330 = property on="ActiveMotor" class="Ring (strict)"() -> ("Strings []"=w490:string[])  [unwired: 2 in, 2 out]
                n331 = Index Array(array=w490, index=w489) -> (element=w488:string)
                n332 = property on="ActiveMotorName::99" class="Str"("Val(Sgnl)"=w488) -> ()  [unwired: 2 in, 2 out]
                n333 = call <vilib>:"Add State(s) to Queue__jki_lib_state_machine.vi"("State(s) in (\"\")"=w494) -> ("States Out"=w493:string)  [unwired: 14 in]
              }
              event "Save Config": Value Change {
                n334 = event-data() -> ()  [unwired: 1 in, 6 out]
                n335 = call <vilib>:"Add State(s) to Queue__jki_lib_state_machine.vi"("State(s) in (\"\")"=w499, "State(s) at Back (\"\")"="Save Config" ("State(s) at Back (\"\")")) -> ("States Out"=w498:string)  [unwired: 13 in]
              }
              event "Load Config": Value Change {
                n336 = event-data() -> ()  [unwired: 1 in, 6 out]
                n337 = call "File Dialog2"("pattern (all files)"="*.cfg", "pattern label"="config") -> ("selected path"=w503:path)  [unwired: 10 in, 3 out]
                n338 = Path To String(path=w503) -> (string=w501:string)
                "config path" <- w501
                n339 = call <vilib>:"Build State String with Arguments__jki_lib_state_machine.vi"("Arguments (\"\")"=w501, "State"="Load Config" ("State(s) at Back (\"\")")) -> ("State with Arguments"=w500:string)  [unwired: 4 in]
                n340 = call <vilib>:"Add State(s) to Queue__jki_lib_state_machine.vi"("State(s) in (\"\")"=w509, "State(s) at Back (\"\")"=w500) -> ("States Out"=w508:string)  [unwired: 13 in]
              }
              event "Save Stats": Value Change {
                n341 = event-data() -> ()  [unwired: 1 in, 6 out]
                n342 = call <vilib>:"Add State(s) to Queue__jki_lib_state_machine.vi"("State(s) in (\"\")"=w514, "State(s) at Back (\"\")"="Save Stats" ("State(s) at Back (\"\")")) -> ("States Out"=w513:string)  [unwired: 13 in]
              }
              event "active CCDs": Value Change {
                n343 = event-data() -> ("NewVal"=w520:i32)  [unwired: 1 in, 5 out]
                n344 = Unbundle By Name(w516) -> ("active cams"=w515:string[])
                n345 = Index Array(array=w515, index=w520) -> (element=w518:string)
                n346 = call <vilib>:"Build State String with Arguments__jki_lib_state_machine.vi"("Arguments (\"\")"=w518, "State"="active" ("State(s) at Back (\"\")")) -> ("State with Arguments"=w517:string)  [unwired: 4 in]
                n347 = call <vilib>:"Add State(s) to Queue__jki_lib_state_machine.vi"("State(s) in (\"\")"=w523, "State(s) at Back (\"\")"=w517) -> ("States Out"=w522:string)  [unwired: 13 in]
              }
              event "Center": Value Change {
                n348 = event-data() -> ()  [unwired: 1 in, 6 out]
                n349 = call <vilib>:"Add State(s) to Queue__jki_lib_state_machine.vi"("State(s) in (\"\")"=w528, "State(s) at Back (\"\")"="Center" ("State(s) at Back (\"\")")) -> ("States Out"=w527:string)  [unwired: 13 in]
              }
              event "new tdms": Value Change {
                n350 = event-data() -> ()  [unwired: 1 in, 6 out]
                n351 = property on="new tdms" class="Bool (strict)"("Value"=FALSE ("new tdms")) -> ()  [unwired: 2 in, 2 out]
                n352 = call <vilib>:"Add State(s) to Queue__jki_lib_state_machine.vi"("State(s) in (\"\")"=w534, "State(s) at Back (\"\")"="newtdms" ("State(s) at Back (\"\")")) -> ("States Out"=w533:string)  [unwired: 13 in]
              }
              event "deivice ini": Value Change {
                n353 = event-data() -> ()  [unwired: 1 in, 6 out]
                n354 = property on="deivice ini" class="Bool (strict)"("Value"=FALSE ("new tdms")) -> ()  [unwired: 2 in, 2 out]
                n355 = call <vilib>:"Add State(s) to Queue__jki_lib_state_machine.vi"("State(s) in (\"\")"=w540, "State(s) at Back (\"\")"="Device Ini" ("State(s) at Back (\"\")")) -> ("States Out"=w539:string)  [unwired: 13 in]
              }
              event "Img to avg": Value Change {
                n356 = event-data() -> ()  [unwired: 1 in, 6 out]
                n357 = property on="Img to avg" class="DigNum (strict)"() -> ("Value"=w543:i32)  [unwired: 2 in, 2 out]
                n358 = Number To Decimal String(number=w543) -> (decimal integer string=w542:string)  [unwired: 1 in]
                n359 = call <vilib>:"Build State String with Arguments__jki_lib_state_machine.vi"("Arguments (\"\")"=w542, "State"="ImgToAvg" ("State(s) at Back (\"\")")) -> ("State with Arguments"=w541:string)  [unwired: 4 in]
                n360 = call <vilib>:"Add State(s) to Queue__jki_lib_state_machine.vi"("State(s) in (\"\")"=w548, "State(s) at Back (\"\")"=w541) -> ("States Out"=w547:string)  [unwired: 13 in]
              }
              event Panel Close? {
                # "Discard the event because we'll close the front panel ourselves in Macro: Exit"
                # "Close Panel button (pressed) Event\n(this executes Macro: Exit to terminate the VI)"
                n361 = event-data() -> ()  [unwired: 1 in, 1 out]
                n362 = call <vilib>:"Add State(s) to Queue__jki_lib_state_machine.vi"("State(s) in Front (\"\")"="Macro: Exit", "State(s) in (\"\")"=w554) -> ("States Out"=w553:string)  [unwired: 13 in]
                n363 = event-data("Discard?"=TRUE) -> ()  [unwired: 1 in, 1 out]
              }
            }
          }
          frame "---------- Core ----------" {
            # "Do not put any code in this frame.\n(it is a separator no-op)"
            n364 = call <vilib>:"Add State(s) to Queue__jki_lib_state_machine.vi"("State(s) in (\"\")"=w558) -> ("States Out"=w557:string)  [unwired: 14 in]
          }
          frame Default {
            w568 = 42 items=["No error", "Argument error", "Memory is full", "Out of zone", "End of file", "File already open", "Generic file I/O error", "File not found", "File permission error", "Disk is full", "Duplicate path", "Too many files open", "System feature not enabled", "Resource file not found", "Cannot add resource", "Resource not found", "Image not found", "Image memory error", "Pen does not exist", "Config type invalid", "Config token not found", "Config parse error", "Config memory error", "Bad external code format", "Bad external code offset", "External code not present", "Null window", "Destroy window error", "Null menu", "Print aborted", "Bad print record", "Print driver error", "Windows error during printing", "Memory error during printing", "Print dialog error", "Generic print error", "Invalid device refnum", "Device not found", "Device parameter error", "Device unit error", "Cannot open device", "Device call aborted", "Generic error", "Cancelled by user", "Object ID too low", "Object ID too high", "Object not in heap", "Unknown heap", "Unknown object (invalid DefProc)", "Unknown object (DefProc not in table)", "Message out of range", "Invalid (null) method", "Unknown message", "Manager call not supported", "Bad address", "Network operation in progress", "Network operation timed out", "Connection is busy", "Network attribute not supported", "Network error", "Address in use", "System out of memory", "Connection aborted", "Connection refused", "Not connected", "Already connected", "Connection closed", "Initialization error (interapplication manager)", "Bad occurrence", "Wait on unbound occurrence handler", "Occurrence queue overflow", "Datalog type conflict", "Unused", "Unrecognized type (interapplication manager)", "Memory corrupt", "Failed to make temporary DLL", "Old CIN version", "Drag socket not found", "Failed to load drop-object", "Failed to register OLE object", "Failed to release OLE object", "Format specifier type mismatch", "Unknown format specifier", "Too few format specifiers", "Too many format specifiers", "Scan failed", "Newer CIN version", "Error converting to variant", "Runtime menu error", "Password tampered", "Variant attribute not found", "Incompatible variant data type", "Event data is not available", "Event Store is not present", "Occurrence is not found", "Event Queue is not created", "Event info is not available", "Refnum passed is NULL", "Error retrieving Class GUID", "Error retrieving CoClass GUID", "Error retrieving TypeLib GUID.", "Bad built application magic bytes.", "Specific driver is different from the specific driver associated with the Logical Name.", "There is no session opened to the class driver.", "Max Error", "MAX - Error with config objects", "MAX - Error loading configuration", "MAX - Group not supported"]
            # "Current State"
            # "Do not delete, rename, or modify this frame.\n(this is used to capture unhandled states and typos)"
            # "Handle mistyped state name (developer tool)"
            n365 = Format Into String(format string="Software Exception: Unhandled State \"%s\"." ("message"), error in=w564, w559) -> (resulting string=w567:string, error out=w566:errorcluster)  [unwired: 1 in]
            n366 = call <vilib>:"Error Cluster From Error Code.vi"("show call chain? (False)"=TRUE, "error in (no error)"=w566, "error message (\"\")"=w567, "error code (0)"=w568) -> ("error out"=w565:errorcluster)  [unwired: 5 in]
            n367 = call <vilib>:"Add State(s) to Queue__jki_lib_state_machine.vi"("State(s) in (\"\")"=w563) -> ("States Out"=w562:string)  [unwired: 14 in]
          }
          frame "Initialize Core Data" {
            # "Do not delete, rename, or modify this frame.\n(this is used to determine panel behavior on exit)"
            # "originally closed?"
            # "exe?"
            # "If panel starts closed or is an EXE, then close it when we exit"
            n368 = property class="VI"() -> ("Front Panel.Open"=w578:bool)  [unwired: 2 in, 2 out]
            n369 = property class="App"() -> ("App.Kind"=w577:T16)  [unwired: 2 in, 2 out]
            n370 = control-ref of="Current VI Reference"() -> (w572:refnum<vi>)
            n371 = Not(x=w578) -> (.not. x?=w575:bool)
            n372 = Equal?(x=w577, y=T16."Run Time System" ("Application:Kind")) -> (x = y?=w574:bool)
            n373 = Or(x=w575, y=w574) -> (x .or. y?=w573:bool)
            n374 = Bundle By Name(cluster=w571, "Core.Current VI Reference"=w572, "Core.Close Panel on Exit?"=w573) -> (w570:T36)
            n375 = call <vilib>:"Add State(s) to Queue__jki_lib_state_machine.vi"("State(s) in (\"\")"=w581) -> ("States Out"=w580:string)  [unwired: 14 in]
          }
          frame "Error Handler" {
            # "Unhandled Error -- Display it"
            # "Handle any errors here.\nYou can also output any states to clean-up after errors occur"
            # "Clear error"
            n376 = call <vilib>:"General Error Handler.vi"("error in (no error)"=w583) -> ()  [unwired: 10 in, 5 out]
            n377 = call <vilib>:"Add State(s) to Queue__jki_lib_state_machine.vi"("State(s) in Front (\"\")"="/* Post Error States", "State(s) in (\"\")"=w587) -> ("States Out"=w586:string)  [unwired: 13 in]
          }
          frame "Exit" {
            # "Do not put any code in this frame.\n(No errors that occur here will be handled.)"
            n378 = call <vilib>:"Add State(s) to Queue__jki_lib_state_machine.vi"("State(s) in (\"\")"=w592) -> ("States Out"=w591:string)  [unwired: 14 in]
          }
          frame "---------- Data ----------" {
            # "Do not put any code in this frame.\n(It is a separator no-op. You can make a copy of this frame to create a new Data frame)"
            n379 = call <vilib>:"Add State(s) to Queue__jki_lib_state_machine.vi"("State(s) in (\"\")"=w596) -> ("States Out"=w595:string)  [unwired: 14 in]
          }
          frame "Data: Initialize" {
            w608 = bool[] [FALSE, FALSE, FALSE, FALSE, FALSE, FALSE, FALSE, FALSE, FALSE, FALSE, FALSE, TRUE]  # speedmode Y
            w609 = bool[] [FALSE, FALSE, FALSE, FALSE, FALSE, FALSE, FALSE, FALSE, FALSE, FALSE, FALSE, TRUE]  # speedmode X
            w610 = bool[] [FALSE, FALSE, FALSE, FALSE, TRUE, TRUE, TRUE, FALSE, FALSE, FALSE, FALSE, FALSE]  # detected
            w612 = cluster{"Lower value":sgl, "Upper value":sgl}[] [{"Lower value"=93.0, "Upper value"=255.0}, {"Lower value"=105.0, "Upper value"=255.0}, {"Lower value"=0.0, "Upper value"=255.0}, {"Lower value"=127.0, "Upper value"=255.0}, {"Lower value"=0.0, "Upper value"=255.0}, {"Lower value"=0.0, "Upper value"=255.0}, {"Lower value"=0.0, "Upper value"=255.0}, {"Lower value"=0.0, "Upper value"=255.0}, {"Lower value"=0.0, "Upper value"=255.0}, {"Lower value"=0.0, "Upper value"=255.0}, {"Lower value"=0.0, "Upper value"=255.0}, {"Lower value"=0.0, "Upper value"=255.0}]  # thresholds
            w623 = FALSE  # Feedback global
            w625 = 0  # active ccd
            w597 = 2  # img to avg
            w636 = T37 {"Current VI Reference"=refnum, "Close Panel on Exit?"=FALSE}  # Core
            # "Initialize the shift-register data, here.\n(data names are defined by what you wire into the bundle function)"
            n380 = TDMS Open(6:FALSE ("disable buffering (T)"), 7:enum16{"1.0", "2.0"}."2.0" ("file format version (2.0)"), 8:w613, 10:T17."create or replace" ("operation"), 11:w611) -> (0:w607:errorcluster, 3:w605:refnum<k34>)  [unwired: 1 in]
            n381 = call "TDMSbuffersize.vi"("error in (no error)"=w607, "group names"=w604, "Data Value Reference in"=w605) -> ("error out"=w606:errorcluster, "Data Value Reference out"=w603:refnum<k34>)  [unwired: 7 in]
            n382 = call <vilib>:"Add State(s) to Queue__jki_lib_state_machine.vi"("State(s) in (\"\")"=w638) -> ("States Out"=w637:string)  [unwired: 14 in]
            n383 = Bundle("Core"=w636, "detection para"="detection para", "thresholds"=w612, "Centroid X"="Centroid X", "Centroid Y"="Centroid Y", "img to avg"=w597, "Mean Centroid X"="Mean Centroid X", "Mean Centroid Y"="Mean Centroid Y", "Offset X"="Offset X", "Offset Y"="Offset Y", "Offset X stats"="Offset X stats", "Offset Y stats"="Offset Y stats", "Size"="Size", "Mean Size"="Mean Size", "Time"="Time", "move properties"="move properties", "active axis refs 2"="active axis refs 2", "active ccd"=w625, "Feedback global"=w623, "Motor X"="Motor X", "Motor Y"="Motor Y", "active cams"="active cams", "Data Value Reference out"=w603, "detected"=w610, "speedmode X"=w609, "speedmode Y"=w608) -> (w599:T36)  [unwired: 1 in]
            n384 = Initialize Array(0.0 ("element"), 12 ("dimension size"), w597) -> (w600:dbl[][])
            n385 = Bundle By Name(cluster=w599, "Centroid X"=w600, "Centroid Y"=w600, "Size"=w600) -> (w598:T36)
          }
          frame "Data: Cleanup" {
            # "Cleanup any data and references, here.\n(this is called automatically, by the Macro: Exit)"
            n386 = Unbundle By Name(w642) -> ("Core.Current VI Reference"=w643:refnum<vi>)
            n387 = Close Reference(reference=w643, error in (no error)=w644) -> (error out=w640:errorcluster)
            n388 = Unbundle By Name(w642) -> ("Data Value Reference out"=w641:refnum<k34>)
            n389 = TDMS Close(8:w640, 11:w641) -> (0:w639:errorcluster)  [unwired: 1 out]
            n390 = call <vilib>:"Add State(s) to Queue__jki_lib_state_machine.vi"("State(s) in (\"\")"=w646) -> ("States Out"=w645:string)  [unwired: 14 in]
          }
          frame "---------- UI ----------" {
            # "Do not put any code in this frame.\n(It is a separator no-op. You can make a copy of this frame to create a new UI frame)"
            n391 = call <vilib>:"Add State(s) to Queue__jki_lib_state_machine.vi"("State(s) in (\"\")"=w650) -> ("States Out"=w649:string)  [unwired: 14 in]
          }
          frame "UI: Initialize" {
            # "Initialize the User Interface, here.\n(this is called automatically, by the Macro: Init)"
            n392 = call <vilib>:"Add State(s) to Queue__jki_lib_state_machine.vi"("State(s) in (\"\")"=w654) -> ("States Out"=w653:string)  [unwired: 14 in]
          }
          frame "UI: Cursor Set" {
            # "Argument"
            # "Set and Unset Cursor Busy.\n(Usage: \"UI: Cursor Set >> Busy|Idle\")"
            n393 = case shown="\"Idle\", Default" w655 {
              tunnel: w657 -> [w662 w664]
              tunnel: [w661 w663] -> w656
              frame "Idle", Default {
                n394 = call <vilib>:"Unset Busy.vi"("error in (no error)"=w662) -> ("error out"=w661:errorcluster)  [unwired: 10 in]
              }
              frame "Busy" {
                n395 = call <vilib>:"Set Busy.vi"("error in (no error)"=w664) -> ("error out"=w663:errorcluster)  [unwired: 9 in, 1 out]
              }
            }
            n396 = call <vilib>:"Add State(s) to Queue__jki_lib_state_machine.vi"("State(s) in (\"\")"=w660) -> ("States Out"=w659:string)  [unwired: 14 in]
          }
          frame "UI: Front Panel State" {
            # "Argument"
            # "Set Front Panel Open or Closed\n(Usage: \"UI: Front Panel State >> Open|Close\")"
            n397 = Unbundle By Name(w665) -> ("Core.Current VI Reference"=w667:refnum<vi>)
            n398 = case shown="\"Open\", Default" w666 {
              tunnel: w669 -> [w675 w686]
              tunnel: [w676 w687] -> w668
              tunnel: w667 -> [_ _]
              frame "Open", Default {
                n399 = property class="VI"(error in=w675) -> (reference out=w673:refnum<vi>, error out=w674:errorcluster, "Front Panel.Open"=w672:bool)  [unwired: 1 in]
                n400 = case shown="False" w672 {
                  tunnel: [w679 w682] -> w676
                  tunnel: w674 -> [w678 w682]
                  tunnel: w673 -> [w677 _]
                  frame False {
                    n401 = invoke class="VI" method="FP.Open"(reference=w677, error in=w678, "Activate"=TRUE, "State"=T18."Standard") -> (error out=w679:errorcluster)  [unwired: 1 in, 4 out]
                  }
                  frame True {
                  }
                }
              }
              frame "Close" {
                n402 = property class="VI"(error in=w686) -> (reference out=w684:refnum<vi>, error out=w685:errorcluster, "Front Panel.Open"=w683:bool)  [unwired: 1 in]
                n403 = case shown="True" w683 {
                  tunnel: [w688 w691] -> w687
                  tunnel: w685 -> [w688 w690]
                  tunnel: w684 -> [_ w689]
                  frame False {
                  }
                  frame True {
                    n404 = invoke class="VI" method="FP.Close"(reference=w689, error in=w690) -> (error out=w691:errorcluster)  [unwired: 1 in, 2 out]
                  }
                }
              }
            }
            n405 = call <vilib>:"Add State(s) to Queue__jki_lib_state_machine.vi"("State(s) in (\"\")"=w671) -> ("States Out"=w670:string)  [unwired: 14 in]
          }
          frame "---------- Macro ----------" {
            # "Do not put any code in this frame.\n(It is a separator no-op. You can make a copy of this frame to create a new Macro frame)"
            n406 = call <vilib>:"Add State(s) to Queue__jki_lib_state_machine.vi"("State(s) in (\"\")"=w695) -> ("States Out"=w694:string)  [unwired: 14 in]
          }
          frame "Macro: Initialize" {
            w702 = "Data: Initialize\nInitialize Core Data\nUI: Initialize\nUI: Front Panel State >> Open\nDevice Ini >> 3000"  # Data: Initialize Initialize Core Data UI: Initialize UI: Front Panel State >> Open Device Ini >> 3000
            # "Initialization Macro\n(This is called once, when the VI starts)"
            n407 = property on="Img to avg" class="DigNum (strict)"() -> ("Value"=w700:i32)  [unwired: 2 in, 2 out]
            n408 = call <vilib>:"Add State(s) to Queue__jki_lib_state_machine.vi"("State(s) in Front (\"\")"=w702, "State(s) in (\"\")"=w705) -> ("States Out"=w697:string)  [unwired: 13 in]
            n409 = Number To Decimal String(number=w700) -> (decimal integer string=w699:string)  [unwired: 1 in]
            n410 = call <vilib>:"Build State String with Arguments__jki_lib_state_machine.vi"("Arguments (\"\")"=w699, "State"="ImgToAvg") -> ("State with Arguments"=w698:string)  [unwired: 4 in]
            n411 = call <vilib>:"Add State(s) to Queue__jki_lib_state_machine.vi"("State(s) in (\"\")"=w697, "State(s) at Back (\"\")"=w698) -> ("States Out"=w696:string)  [unwired: 13 in]
          }
          frame "Macro: Exit" {
            # "Exit Macro\n(This is called once, when the VI exits)"
            n412 = Unbundle By Name(w707) -> ("Core.Close Panel on Exit?"=w706:bool)
            n413 = Select(t="UI: Front Panel State >> Close", s=w706, f="") -> (s? t:f=w710:string)
            n414 = call <vilib>:"Add State(s) to Queue__jki_lib_state_machine.vi"("State(s) in (\"\")"=w710, "State(s) at Back (\"\")"="Data: Cleanup\nExit") -> ("States Out"=w708:string)  [unwired: 13 in]
            n415 = call <vilib>:"Add State(s) to Queue__jki_lib_state_machine.vi"("State(s) in Front (\"\")"=w708, "State(s) in (\"\")"=w715) -> ("States Out"=w714:string)  [unwired: 13 in]
          }
          frame "---------- Ini and Configure ----------" {
            # "Template Separator\n(You can make a copy of, or modify, this frame)"
            n416 = call <vilib>:"Add State(s) to Queue__jki_lib_state_machine.vi"("State(s) in (\"\")"=w719) -> ("States Out"=w718:string)  [unwired: 14 in]
          }
          frame "Device Ini" {
            # "Your code here.\n(You can make a copy of, or modify, this frame)"
            n417 = Empty String/Path?(string/path=w732) -> (empty?=w730:bool)
            n418 = case shown="False" w730 {
              tunnel: w732 -> [w769 _]
              tunnel: [w768 0] -> w731
              frame False {
                n419 = Decimal String To Number(string=w769) -> (number=w768:i32)  [unwired: 2 in, 1 out]
              }
              frame True {
              }
            }
            n420 = flat-sequence {
              tunnel: w736 -> [w772]
              tunnel: [w772] -> w735
              tunnel: w731 -> [w771]
              tunnel: w735 -> [w775]
              tunnel: [w773] -> w723
              frame #0 {
                n421 = Wait (ms)(milliseconds to wait=w771) -> ()  [unwired: 1 out]
              }
              frame #1 {
                n422 = for {
                  tunnel: w775 -> [w777] mode=indexing
                  shift-right: [w778] -> w773
                  shift-left: string[] [] -> [w779]
                  n423 = Empty String/Path?(string/path=w777) -> (empty?=w776:bool)
                  n424 = case shown="False" w776 {
                    tunnel: w779 -> [w782 w788]
                    tunnel: [w781 w788] -> w778
                    tunnel: w777 -> [w780 _]
                    frame False {
                      n425 = call "send command.vi"("Device Name"=w780) -> ("status"=w783:bool)  [unwired: 4 in]
                      n426 = case shown="False" w783 {
                        tunnel: w782 -> [w784 w787]
                        tunnel: [w784 w786] -> w781
                        tunnel: w780 -> [_ w785]
                        frame False {
                        }
                        frame True {
                          n427 = Build Array (concatenate)(w787, w785) -> (w786:string[])
                        }
                      }
                    }
                    frame True {
                    }
                  }
                }
              }
            }
            n428 = Unbundle By Name(w729) -> ("active cams"=w724:string[])
            n429 = call <vilib>:"Add State(s) to Queue__jki_lib_state_machine.vi"("State(s) in (\"\")"=w737) -> ("States Out"=w721:string)  [unwired: 14 in]
            n430 = Empty Array?(array=w724) -> (empty?=w726:bool)
            n431 = Equal?(x=w724, y=w723) -> (x = y?=w727:bool[])
            n432 = Not(x=w726) -> (.not. x?=w725:bool)
            n433 = Build Array (concatenate)(w727, w725) -> (w728:bool[])
            n434 = And Array Elements(Boolean array=w728) -> (logical AND=w722:bool)
            n435 = case shown="False" w722 {
              tunnel: [w754 w767] -> w734
              tunnel: w729 -> [w739 w767]
              tunnel: w723 -> [w740 _]
              tunnel: w721 -> [w749 w766]
              tunnel: [w747 w766] -> w720
              frame False {
                n436 = Bundle By Name(cluster=w739, "active cams"=w740) -> (w755:T36)
                n437 = property on="active CCDs" class="LstBox (strict)"("Item Names"=w740) -> ()  [unwired: 2 in, 2 out]
                n438 = Array Size(array=w740) -> (size(s)=w758:i32)
                n439 = for {
                  N: 1 -> [_]
                  shift-right: [w760] -> w753
                  shift-left: timestamp[][] [] ("Time") -> [w762]
                  n440 = for {
                    N: 12 -> [_]
                    tunnel: w762 -> [w765] mode=indexing
                    tunnel: [w763] -> w760 mode=indexing
                    n441 = Get Date/Time In Seconds() -> (seconds since 1Jan1904=w764:timestamp)
                    n442 = Build Array (concatenate)(w765, w764) -> (w763:timestamp[])
                  }
                }
                n443 = Unbundle By Name(w739) -> ("img to avg"=w738:i32)
                n444 = Initialize Array(0.0 ("element"), w758, 0 ("dimension size")) -> (w756:dbl[][])
                n445 = Initialize Array(0.0 ("element"), 12 ("dimension size"), w738) -> (w741:dbl[][])
                n446 = Bundle By Name(cluster=w755, "Offset X stats"=w756, "Offset Y stats"=w756, "Centroid X"=w741, "Centroid Y"=w741, "Mean Centroid X"=w756, "Mean Centroid Y"=w756, "Offset X"=w756, "Offset Y"=w756, "Size"=w741, "Mean Size"=w756, "Motor X"=w756, "Motor Y"=w756) -> (w754:T36)
                n447 = property on="Time" class="Arr (strict)"("Value"=w753) -> ()  [unwired: 2 in, 2 out]
                n448 = property on="config path" class="Str"() -> ("Value"=w746:string)  [unwired: 2 in, 2 out]
                n449 = call <vilib>:"Add State(s) to Queue__jki_lib_state_machine.vi"("State(s) in Front (\"\")"="newtdms\nMove Config\nDetection Config\nactive\nCenter" ("State(s) in Front (\"\")"), "State(s) in (\"\")"=w749) -> ("States Out"=w748:string)  [unwired: 13 in]
                n450 = call <vilib>:"Build State String with Arguments__jki_lib_state_machine.vi"("Arguments (\"\")"=w746, "State"="Load Config" ("State(s) in Front (\"\")")) -> ("State with Arguments"=w744:string)  [unwired: 4 in]
                n451 = call <vilib>:"Add State(s) to Queue__jki_lib_state_machine.vi"("State(s) in Front (\"\")"=w744, "State(s) in (\"\")"=w748) -> ("States Out"=w747:string)  [unwired: 13 in]
                "name array" <- w740
              }
              frame True {
              }
            }
          }
          frame "Load Config" {
            # "Your code here.\n(You can make a copy of, or modify, this frame)"
            n452 = Unbundle By Name(w791) -> ("detection para"=w834:T3[], "move properties"=w831:T2[], "thresholds"=w826:cluster{"Lower value":sgl, "Upper value":sgl}[])
            n453 = Empty String/Path?(string/path=w790) -> (empty?=w789:bool)
            n454 = property on="Load Config" class="Bool (strict)"("Value"=FALSE ("Load Config")) -> ()  [unwired: 2 in, 2 out]
            n455 = case shown="False" w789 {
              tunnel: [w845 T5 {"CCDs"=[], "move properties"=[], "detection para"=[], "thresholds"=[], "Value"={"Motor CCD 1"=0, "Motor CCD 2"=0, "Motor CCD 3"=0, "Motor CCD 4"=0, "Motor CCD 5"=0, "Motor CCD 6"=0, "Motor CCD 7"=0, "Motor CCD 8"=0, "Motor CCD 9"=0, "Motor CCD 10"=0, "Motor CCD 11"=0, "Motor CCD 12"=0}} ("output cluster 2")] -> w836
              tunnel: [w843 w852] -> w796
              tunnel: w790 -> [w842 _]
              tunnel: w793 -> [w840 w852]
              tunnel: w791 -> [_ _]
              frame False {
                n456 = String To Path(string=w842) -> (path=w841:path)
                n457 = Open/Create/Replace File(file path (use dialog)=w841, error in=w840, operation (0:open)=T19."open or create") -> (refnum out=w847:refnum<file>, error out=w848:errorcluster)  [unwired: 3 in, 1 out]
                n458 = Read from Binary File(5:"output cluster 2", 8:w848, 11:w847) -> (0:w849:errorcluster, 2:w845:T5, 3:w850:refnum<file>)  [unwired: 3 in, 1 out]
                n459 = Close File(refnum=w850, error in=w849) -> (error out=w843:errorcluster)  [unwired: 1 out]
              }
              frame True {
              }
            }
            n460 = Unbundle By Name(w836) -> ("Value"=w823:T7, "CCDs"=w835:string[], "detection para"=w833:T3[], "move properties"=w832:T2[], "thresholds"=w827:cluster{"Lower value":sgl, "Upper value":sgl}[])
            n461 = Cluster To Array(cluster=w823) -> (array=w824:u16[])
            n462 = call <vilib>:"Add State(s) to Queue__jki_lib_state_machine.vi"("State(s) in (\"\")"=w839, "State(s) at Back (\"\")"="Motor Config" ("State(s) at Back (\"\")")) -> ("States Out"=w838:string)  [unwired: 13 in]
            n463 = for {
              tunnel: w835 -> [w868]
              tunnel: w833 -> [w870]
              tunnel: w832 -> [w869]
              shift-right: [w862] -> w830
              shift-left: w834 -> [w867]
              shift-right: [w860] -> w829
              shift-left: w831 -> [w866]
              tunnel: w792 -> [w865] mode=indexing
              tunnel: w827 -> [w861]
              shift-right: [w857] -> w825
              shift-left: w826 -> [w859]
              tunnel: w824 -> [w856]
              tunnel: [w853] -> w822 mode=indexing
              i -> [w854]
              n464 = call-poly <userlib>:"Filter 1D Array__ogtk.vi"("items to filter"=w865, "array"=w868) -> ("filtered item indices"=w871:i32[])  [unwired: 4 in, 1 out]
              n465 = Index Array(array=w871) -> (element=w855:i32)  [unwired: 1 in]
              n466 = Index Array(array=w856, index=w855) -> (element=w853:u16)
              n467 = Index Array(array=w870, index=w855) -> (element=w864:T3)
              n468 = Index Array(array=w869, index=w855) -> (element=w863:T2)
              n469 = Index Array(array=w861, index=w855) -> (element=w858:cluster{"Lower value":sgl, "Upper value":sgl})
              n470 = Replace Array Subset(array=w867, new element=w864, index=w854) -> (w862:T3[])
              n471 = Replace Array Subset(array=w866, new element=w863, index=w854) -> (w860:T2[])
              n472 = Replace Array Subset(array=w859, new element=w858, index=w854) -> (w857:cluster{"Lower value":sgl, "Upper value":sgl}[])
            }
            n473 = Index Array(array=w822, index #1=0 ("index (row)"), index #2=1 ("index (row)"), index #3=2 ("index (row)"), index #4=3 ("index (row)"), index #5=4 ("index (row)"), index #6=5 ("index (row)"), index #7=6 ("index (row)"), index #8=7 ("index (row)"), index #9=8 ("index (row)"), index #10=9 ("index (row)"), index #11=10 ("index (row)"), index #12=11 ("index (row)")) -> (element #1=w809:u16, element #2=w808:u16, element #3=w807:u16, element #4=w806:u16, element #5=w805:u16, element #6=w804:u16, element #7=w803:u16, element #8=w802:u16, element #9=w801:u16, element #10=w800:u16, element #11=w799:u16, element #12=w798:u16)
            n474 = Bundle By Name(cluster=w823, "Motor CCD 1"=w809, "Motor CCD 2"=w808, "Motor CCD 3"=w807, "Motor CCD 4"=w806, "Motor CCD 5"=w805, "Motor CCD 6"=w804, "Motor CCD 7"=w803, "Motor CCD 8"=w802, "Motor CCD 9"=w801, "Motor CCD 10"=w800, "Motor CCD 11"=w799, "Motor CCD 12"=w798) -> (w797:T7)
            n475 = Bundle By Name(cluster=w791, "detection para"=w830, "move properties"=w829, "thresholds"=w825) -> (w828:T36)
            n476 = property on="associated motors" class="Clust (strict)"(error in=w796, "Val(Sgnl)"=w797) -> (error out=w795:errorcluster)  [unwired: 1 in, 1 out]
          }
          frame "Save Config" {
            # "Your code here.\n(You can make a copy of, or modify, this frame)"
            n477 = Unbundle By Name(w889) -> ("move properties"=w875:T2[], "detection para"=w884:T3[], "thresholds"=w872:cluster{"Lower value":sgl, "Upper value":sgl}[])
            n478 = property on="associated motors" class="Clust (strict)"() -> ("Value"=w883:T7)  [unwired: 2 in, 2 out]
            n479 = property on="Save Config" class="Bool (strict)"("Value"=FALSE ("Save Config")) -> ()  [unwired: 2 in, 2 out]
            n480 = local read "CCDs"() -> (w873:string[])
            n481 = call "File Dialog"("pattern (all files)"="*.cfg", "pattern label"="config") -> ("selected path"=w877:path)  [unwired: 10 in, 3 out]
            n482 = Bundle("CCDs"=w873, "move properties"=w875, "detection para"=w884, "thresholds"=w872, "Value"=w883) -> (w876:T5)  [unwired: 1 in]
            n483 = Open/Create/Replace File(file path (use dialog)=w877, error in=w881, operation (0:open)=T19."replace or create with confirmation") -> (refnum out=w885:refnum<file>, error out=w886:errorcluster)  [unwired: 3 in, 1 out]
            n484 = Write to Binary File(file (use dialog)=w885, data=w876, error in=w886) -> (refnum out=w888:refnum<file>, error out=w887:errorcluster)  [unwired: 3 in, 1 out]
            n485 = Close File(refnum=w888, error in=w887) -> (error out=w880:errorcluster)  [unwired: 1 out]
            n486 = call <vilib>:"Add State(s) to Queue__jki_lib_state_machine.vi"("State(s) in (\"\")"=w891) -> ("States Out"=w890:string)  [unwired: 14 in]
          }
          frame "active" {
            # "Your code here.\n(You can make a copy of, or modify, this frame)"
            n487 = call-poly <userlib>:"Filter 1D Array__ogtk.vi"("items to filter"=w901, "array"=w897) -> ("filtered item indices"=w900:i32[])  [unwired: 4 in, 1 out]
            n488 = Unbundle By Name(w896) -> ("move properties"=w899:T2[], "detection para"=w894:T3[])  [unwired: 1 out]
            n489 = Index Array(array=w900) -> (element=w892:i32)  [unwired: 1 in]
            n490 = Index Array(array=w899, index=w892) -> (element=w898:T2)
            n491 = Index Array(array=w894, index=w892) -> (element=w893:T3)
            n492 = property on="move config" class="Clust (strict)"("Value"=w898) -> ()  [unwired: 2 in, 2 out]
            n493 = property on="beam detection para" class="Clust (strict)"("Value"=w893) -> ()  [unwired: 2 in, 2 out]
            n494 = Bundle By Name(cluster=w896, "active ccd"=w892) -> (w895:T36)
            n495 = call <vilib>:"Add State(s) to Queue__jki_lib_state_machine.vi"("State(s) in (\"\")"=w904) -> ("States Out"=w903:string)  [unwired: 14 in]
          }
          frame "Detection Config" {
            # "Your code here.\n(You can make a copy of, or modify, this frame)"
            n496 = Unbundle By Name(w909) -> ("detection para"=w905:T3[], "active ccd"=w910:i32)
            n497 = Replace Array Subset(array=w905, new element="beam detection para", index=w910) -> (w906:T3[])
            n498 = Bundle By Name(cluster=w909, "detection para"=w906) -> (w908:T36)
            n499 = call <vilib>:"Add State(s) to Queue__jki_lib_state_machine.vi"("State(s) in (\"\")"=w913) -> ("States Out"=w912:string)  [unwired: 14 in]
          }
          frame "Motor Config" {
            # "Your code here.\n(You can make a copy of, or modify, this frame)"
            n500 = Unbundle By Name("associated motors") -> ("Motor CCD 1"=w935:u16, "Motor CCD 2"=w936:u16, "Motor CCD 3"=w937:u16, "Motor CCD 4"=w930:u16, "Motor CCD 5"=w929:u16, "Motor CCD 6"=w928:u16, "Motor CCD 7"=w927:u16, "Motor CCD 8"=w926:u16, "Motor CCD 9"=w925:u16, "Motor CCD 10"=w924:u16, "Motor CCD 11"=w923:u16, "Motor CCD 12"=w922:u16)
            n501 = local read "motor refs"() -> (w933:refnum<vi>[])
            n502 = property on="ActiveMotor" class="Ring (strict)"() -> ("Value"=w916:u16)  [unwired: 2 in, 2 out]
            n503 = property on="ActiveMotor" class="Ring (strict)"() -> ("Strings []"=w918:string[])  [unwired: 2 in, 2 out]
            n504 = Build Array(w935, w936, w937, w930, w929, w928, w927, w926, w925, w924, w923, w922) -> (w921:u16[])
            n505 = Increment(x=w921) -> (x+1=w920:u16[])
            n506 = Index Array(array=w918, index=w916) -> (element=w917:string)
            n507 = for {
              tunnel: w920 -> [w952] mode=indexing
              tunnel: w933 -> [w947]
              tunnel: [w943] -> w919 mode=indexing
              tunnel: [w942] -> w915 mode=indexing
              tunnel: [w941] -> w914 mode=indexing
              n508 = Multiply(x=w952, y=u16 3) -> (x*y=w948:u16)
              n509 = Subtract(x=w948, y=u16 3) -> (x-y=w942:u16)
              n510 = Subtract(x=w948, y=u16 2) -> (x-y=w941:u16)
              n511 = Index Array(array=w947, index=w942) -> (element=w946:refnum<vi>)
              n512 = Index Array(array=w947, index=w941) -> (element=w945:refnum<vi>)
              n513 = Bundle By Name(cluster="active Axis ref", "Ref X"=w946, "Ref Y"=w945) -> (w943:cluster{"Ref X":refnum<vi>, "Ref Y":refnum<vi>})
            }
            "Array" <- w915
            "Array 2" <- w914
            n514 = property on="ActiveMotorName::99" class="Str"("Val(Sgnl)"=w917) -> ()  [unwired: 2 in, 2 out]
            n515 = call <vilib>:"Add State(s) to Queue__jki_lib_state_machine.vi"("State(s) in (\"\")"=w940) -> ("States Out"=w939:string)  [unwired: 14 in]
            n516 = Bundle By Name(cluster=w932, "active axis refs 2"=w919) -> (w931:T36)
          }
          frame "Move Config" {
            # "Your code here.\n(You can make a copy of, or modify, this frame)"
            n517 = Unbundle By Name(w954) -> ("move properties"=w958:T2[], "active ccd"=w957:i32)
            n518 = Replace Array Subset(array=w958, new element="move config", index=w957) -> (w955:T2[])
            n519 = Bundle By Name(cluster=w954, "move properties"=w955) -> (w953:T36)
            n520 = call <vilib>:"Add State(s) to Queue__jki_lib_state_machine.vi"("State(s) in (\"\")"=w961) -> ("States Out"=w960:string)  [unwired: 14 in]
          }
          frame "----------Centroid & Move----------" {
            # "Template Separator\n(You can make a copy of, or modify, this frame)"
            n521 = call <vilib>:"Add State(s) to Queue__jki_lib_state_machine.vi"("State(s) in (\"\")"=w965) -> ("States Out"=w964:string)  [unwired: 14 in]
          }
          frame "detected" {
            n522 = Unbundle By Name(w968) -> ("Offset X"=w1010:dbl[][], "Offset Y"=w1009:dbl[][], "Size"=w1008:dbl[][], "Mean Size"=w1007:dbl[][], "Time"=w1004:timestamp[][], "Motor X"=w982:dbl[][], "active axis refs 2"=w981:T12, "Motor Y"=w980:dbl[][])
            n523 = Spreadsheet String To Array(format string="%s", spreadsheet string=w986, array type (2D Dbl)=string[] []) -> (array=w975:string[])  [unwired: 1 in]
            n524 = call-poly <userlib>:"Filter 1D Array__ogtk.vi"("items to filter"=w975, "array"=w976) -> ("filtered item indices"=w973:i32[])  [unwired: 4 in, 1 out]
            n525 = for {
              tunnel: w976 -> [w1027] mode=indexing
              tunnel: w975 -> [w1026]
              tunnel: [w1024] -> w977 mode=indexing
              n526 = for {
                tunnel: w1027 -> [w1030]
                tunnel: [w1029] -> w1025 mode=indexing
                tunnel: w1026 -> [w1028] mode=indexing
                n527 = Equal?(x=w1030, y=w1028) -> (x = y?=w1029:bool)
              }
              n528 = Or Array Elements(Boolean array=w1025) -> (logical OR=w1024:bool)
            }
            n529 = for {
              N: 12 -> [_]
              tunnel: w973 -> [w1023]
              tunnel: [w1020] -> w972 mode=indexing
              i -> [w1022]
              n530 = Equal?(x=w1023, y=w1022) -> (x = y?=w1021:bool[])
              n531 = Or Array Elements(Boolean array=w1021) -> (logical OR=w1020:bool)
            }
            "Array 3" <- w972
            n532 = call <vilib>:"Build State String with Arguments__jki_lib_state_machine.vi"("Arguments (\"\")"=w986, "State"="stats") -> ("State with Arguments"=w985:string)  [unwired: 4 in]
            n533 = Unbundle By Name(w968) -> ("Mean Centroid X"=w1015:dbl[][], "Mean Centroid Y"=w1014:dbl[][], "Centroid X"=w1017:dbl[][], "Centroid Y"=w1016:dbl[][])
            n534 = call <vilib>:"Add State(s) to Queue__jki_lib_state_machine.vi"("State(s) in (\"\")"=w984, "State(s) at Back (\"\")"=w985) -> ("States Out"=w983:string)  [unwired: 13 in]
            n535 = for {
              tunnel: w1017 -> [w1080]
              tunnel: w1016 -> [w1079]
              tunnel: w1015 -> [w1078]
              tunnel: w1014 -> [w1077]
              tunnel: [w1076] -> w1001 mode=indexing
              tunnel: [w1075] -> w1012 mode=indexing
              tunnel: w1011 -> [w1048] mode=indexing
              tunnel: w1010 -> [w1074]
              tunnel: w1009 -> [w1073]
              tunnel: [w1072] -> w989 mode=indexing
              tunnel: [w1071] -> w1002 mode=indexing
              tunnel: w1008 -> [w1070]
              tunnel: w1007 -> [w1069]
              tunnel: [w1068] -> w1006 mode=indexing
              tunnel: w1004 -> [w1067]
              tunnel: [w1066] -> w1003 mode=indexing
              tunnel: w982 -> [w1040]
              tunnel: w981 -> [w1039]
              tunnel: w980 -> [w1038]
              tunnel: [w1037] -> w979 mode=indexing
              tunnel: [w1036] -> w978 mode=indexing
              tunnel: w977 -> [w1035]
              i -> [w1034]
              n536 = Unbundle By Name(w1048) -> ("Target.X::12"=w1051:refnum<vi>, "Target.Y::12"=w1050:refnum<vi>)
              n537 = Index Array(array=w1040, index (row)=w1034) -> (element=w1043:dbl[])  [unwired: 1 in]
              n538 = Index Array(array=w1039, index=w1034) -> (element=w1042:cluster{"Ref X":refnum<vi>, "Ref Y":refnum<vi>})
              n539 = Index Array(array=w1038, index (row)=w1034) -> (element=w1047:dbl[])  [unwired: 1 in]
              n540 = Index Array(array=w1078, index (row)=w1034) -> (element=w1062:dbl[])  [unwired: 1 in]
              n541 = Index Array(array=w1077, index (row)=w1034) -> (element=w1063:dbl[])  [unwired: 1 in]
              n542 = Index Array(array=w1080, index (row)=w1034) -> (element=w1065:dbl[])  [unwired: 1 in]
              n543 = Index Array(array=w1079, index (row)=w1034) -> (element=w1064:dbl[])  [unwired: 1 in]
              n544 = Index Array(array=w1074, index (row)=w1034) -> (element=w1059:dbl[])  [unwired: 1 in]
              n545 = Index Array(array=w1073, index (row)=w1034) -> (element=w1058:dbl[])  [unwired: 1 in]
              n546 = Index Array(array=w1070, index (row)=w1034) -> (element=w1056:dbl[])  [unwired: 1 in]
              n547 = Index Array(array=w1069, index (row)=w1034) -> (element=w1055:dbl[])  [unwired: 1 in]
              n548 = Index Array(array=w1067, index (row)=w1034) -> (element=w1052:timestamp[])  [unwired: 1 in]
              n549 = Index Array(array=w1035, index=w1034) -> (element=w1033:bool)
              n550 = Unbundle By Name(w1042) -> ("Ref X"=w1041:refnum<vi>, "Ref Y"=w1045:refnum<vi>)
              n551 = property class="DigNum (strict)"(reference=w1051) -> ("Value"=w1032:dbl)  [unwired: 1 in, 2 out]
              n552 = property class="DigNum (strict)"(reference=w1050) -> ("Value"=w1049:dbl)  [unwired: 1 in, 2 out]
              n553 = call <vilib>:"Std Deviation and Variance.vi"("X"=w1065) -> ("mean"=w1031:dbl)  [unwired: 1 in, 2 out]
              n554 = call <vilib>:"Std Deviation and Variance.vi"("X"=w1064) -> ("mean"=w1061:dbl)  [unwired: 1 in, 2 out]
              n555 = call <vilib>:"Std Deviation and Variance.vi"("X"=w1056) -> ("mean"=w1054:dbl)  [unwired: 1 in, 2 out]
              n556 = Get Date/Time In Seconds() -> (seconds since 1Jan1904=w1053:timestamp)
              n557 = property class="DigNum (strict)"(reference=w1041) -> ("Value"=w1044:dbl)  [unwired: 1 in, 2 out]
              n558 = property class="DigNum (strict)"(reference=w1045) -> ("Value"=w1046:dbl)  [unwired: 1 in, 2 out]
              n559 = Subtract(x=w1032, y=w1031) -> (x-y=w1060:dbl)
              n560 = Subtract(x=w1049, y=w1061) -> (x-y=w1057:dbl)
              n561 = case shown="True" w1033 {
                tunnel: [w1098 w1112] -> w1076
                tunnel: [w1097 w1111] -> w1075
                tunnel: [w1096 w1110] -> w1072
                tunnel: [w1095 w1109] -> w1071
                tunnel: [w1094 w1108] -> w1068
                tunnel: [w1093 w1107] -> w1066
                tunnel: w1063 -> [w1092 w1106]
                tunnel: w1062 -> [w1091 w1105]
                tunnel: w1031 -> [w1090 _]
                tunnel: w1061 -> [w1089 _]
                tunnel: w1060 -> [w1088 _]
                tunnel: w1059 -> [w1087 w1104]
                tunnel: w1058 -> [w1086 w1103]
                tunnel: w1057 -> [w1085 _]
                tunnel: w1055 -> [w1084 w1102]
                tunnel: w1054 -> [w1083 _]
                tunnel: w1053 -> [w1082 w1101]
                tunnel: w1052 -> [w1081 w1100]
                frame True {
                  n562 = Build Array (concatenate)(w1091, w1090) -> (w1098:dbl[])
                  n563 = Build Array (concatenate)(w1092, w1089) -> (w1097:dbl[])
                  n564 = Build Array (concatenate)(w1087, w1088) -> (w1096:dbl[])
                  n565 = Build Array (concatenate)(w1086, w1085) -> (w1095:dbl[])
                  n566 = Build Array (concatenate)(w1084, w1083) -> (w1094:dbl[])
                  n567 = Build Array (concatenate)(w1081, w1082) -> (w1093:timestamp[])
                }
                frame False {
                  w1099 = 0.0
                  n568 = Build Array (concatenate)(w1105, w1099) -> (w1112:dbl[])
                  n569 = Build Array (concatenate)(w1106, w1099) -> (w1111:dbl[])
                  n570 = Build Array (concatenate)(w1104, w1099) -> (w1110:dbl[])
                  n571 = Build Array (concatenate)(w1103, w1099) -> (w1109:dbl[])
                  n572 = Build Array (concatenate)(w1102, w1099) -> (w1108:dbl[])
                  n573 = Build Array (concatenate)(w1100, w1101) -> (w1107:timestamp[])
                }
              }
              n574 = Build Array (concatenate)(w1047, w1046) -> (w1036:dbl[])
              n575 = Build Array (concatenate)(w1043, w1044) -> (w1037:dbl[])
            }
            n576 = local write "Numeric"(0.0 ("Numeric")) -> ()
            n577 = Array Size(array=w989) -> (size(s)=w1000:i32[])
            n578 = Index Array(array=w1000, index=1) -> (element=w998:i32)
            "History index" <- w998
            n579 = call <vilib>:"Add State(s) to Queue__jki_lib_state_machine.vi"("State(s) in (\"\")"=w983, "State(s) at Back (\"\")"="Check Move\ntdms" ("State(s) at Back (\"\")")) -> ("States Out"=w992:string)  [unwired: 13 in]
            n580 = Unbundle By Name(w968) -> ("img to avg"=w967:i32)
            n581 = Decrement(x=w967) -> (x-1=w966:i32)
            n582 = Initialize Array(0.0 ("element"), 12 ("dimension size"), w966) -> (w969:dbl[][])
            n583 = Greater?(x=w998, y="History Size") -> (0:w996:bool)
            n584 = Bundle By Name(cluster=w968, "Centroid X"=w969, "Centroid Y"=w969, "Mean Centroid X"=w1001, "Mean Centroid Y"=w1012, "Offset X"=w989, "Offset Y"=w1002, "Mean Size"=w1006, "Size"=w969, "Time"=w1003, "Motor X"=w979, "Motor Y"=w978) -> (w1013:T36)
            n585 = Select(t="history" ("State(s) at Back (\"\")"), s=w996, f="") -> (s? t:f=w993:string)
            n586 = call <vilib>:"Add State(s) to Queue__jki_lib_state_machine.vi"("State(s) in (\"\")"=w992, "State(s) at Back (\"\")"=w993) -> ("States Out"=w991:string)  [unwired: 13 in]
          }
          frame "Check Move" {
            (unwired) "Device Ini" ("State(s) in Front (\"\")")
            # "Your code here.\n(You can make a copy of, or modify, this frame)"
            n587 = Unbundle By Name(w1117) -> ("move properties"=w1120:T2[], "Mean Size"=w1143:dbl[][], "move properties"=w1146:T2[], "Offset X"=w1145:dbl[][], "Offset Y"=w1144:dbl[][], "active cams"=w1124:string[])
            n588 = for {
              tunnel: w1146 -> [w1211]
              tunnel: w1145 -> [w1210]
              tunnel: w1144 -> [w1209]
              tunnel: w1143 -> [w1212]
              tunnel: [w1228] -> w1142 mode=indexing
              tunnel: [w1224] -> w1141 mode=indexing
              tunnel: w1124 -> [w1214] mode=indexing
              tunnel: [w1246] -> w1140 mode=indexing
              tunnel: [w1245] -> w1139 mode=indexing
              tunnel: w1120 -> [w1204]
              tunnel: [w1222] -> w1118 mode=indexing
              tunnel: [w1217] -> w1114 mode=indexing
              tunnel: "Speedmode @" -> [w1216]
              tunnel: w1113 -> [w1215]
              n589 = call-poly <userlib>:"Filter 1D Array__ogtk.vi"("items to filter"=w1214, "array"=w1215) -> ("filtered item indices"=w1213:i32[])  [unwired: 4 in, 1 out]
              n590 = Index Array(array=w1213) -> (element=w1203:i32)  [unwired: 1 in]
              n591 = Index Array(array=w1212, index (row)=w1203) -> (element=w1208:dbl[])  [unwired: 1 in]
              n592 = Index Array(array=w1211, index=w1203) -> (element=w1207:T2)
              n593 = Index Array(array=w1210, index (row)=w1203) -> (element=w1206:dbl[])  [unwired: 1 in]
              n594 = Index Array(array=w1204, index=w1203) -> (element=w1202:T2)
              n595 = Index Array(array=w1209, index (row)=w1203) -> (element=w1205:dbl[])  [unwired: 1 in]
              n596 = Unbundle By Name(w1207) -> ("Tolerance [%]"=w1239:dbl)
              n597 = Reverse 1D Array(array=w1206) -> (reversed array=w1244:dbl[])
              n598 = Reverse 1D Array(array=w1205) -> (reversed array=w1243:dbl[])
              n599 = Reverse 1D Array(array=w1208) -> (reversed array=w1238:dbl[])
              n600 = Unbundle By Name(w1202) -> ("enable feedback"=w1227:bool)
              n601 = Index Array(array=w1244) -> (element=w1242:dbl)  [unwired: 1 in]
              n602 = Index Array(array=w1243) -> (element=w1241:dbl)  [unwired: 1 in]
              n603 = Index Array(array=w1238) -> (element=w1237:dbl)  [unwired: 1 in]
              n604 = Absolute Value(x=w1242) -> (abs(x)=w1223:dbl)
              n605 = Absolute Value(x=w1241) -> (abs(x)=w1220:dbl)
              n606 = Square Root(x=w1237) -> (sqrt(x)=w1236:dbl)
              n607 = Divide(x=w1239, y=100.0) -> (x/y=w1235:dbl)
              n608 = Multiply(x=w1236, y=w1235) -> (x*y=w1219:dbl)
              n609 = Not Equal To 0?(x=w1220) -> (x != 0?=w1225:bool)
              n610 = Not Equal To 0?(x=w1223) -> (x != 0?=w1230:bool)
              n611 = Greater Or Equal?(x=w1223, y=w1219) -> (x >= y?=w1229:bool)
              n612 = Greater Or Equal?(x=w1220, y=w1219) -> (x >= y?=w1226:bool)
              n613 = Divide(x=w1223, y=w1219) -> (x/y=w1221:dbl)
              n614 = Divide(x=w1220, y=w1219) -> (x/y=w1218:dbl)
              n615 = Compound Arithmetic op=AND(w1227, w1230, w1229) -> (w1228:bool)
              n616 = Compound Arithmetic op=AND(w1227, w1226, w1225) -> (w1224:bool)
              n617 = Boolean To (0,1)(Boolean=w1224) -> (0, 1=w1231:i16)
              n618 = Greater?(x=w1221, y=w1216) -> (0:w1222:bool)
              n619 = Greater?(x=w1218, y=w1216) -> (0:w1217:bool)
              n620 = Multiply(x=w1231, y=w1220) -> (x*y=w1232:dbl)
              n621 = Boolean To (0,1)(Boolean=w1228) -> (0, 1=w1234:i16)
              n622 = Multiply(x=w1234, y=w1223) -> (x*y=w1233:dbl)
              n623 = Bundle(w1232, "GUIdevice 8"=w1214) -> (w1245:cluster{dbl, "GUIdevice 8":string})  [unwired: 1 in]
              n624 = Bundle(w1233, "GUIdevice 8"=w1214) -> (w1246:cluster{dbl, "GUIdevice 8":string})  [unwired: 1 in]
            }
            "required X" <- w1142
            "required Y" <- w1141
            "speedmode X" <- w1118
            "speedmode Y" <- w1114
            n625 = case shown="True" "Align" {
              tunnel: w1140 -> [w1154 w1159]
              tunnel: w1139 -> [w1153 w1156]
              tunnel: [w1152 w1158] -> w1136
              tunnel: [w1151 w1155] -> w1130
              frame False {
                n626 = Sort 1D Array(array=w1153) -> (sorted array=w1150:cluster{dbl, "GUIdevice 8":string}[])
                n627 = Sort 1D Array(array=w1154) -> (sorted array=w1149:cluster{dbl, "GUIdevice 8":string}[])
                n628 = Reverse 1D Array(array=w1150) -> (reversed array=w1151:cluster{dbl, "GUIdevice 8":string}[])
                n629 = Reverse 1D Array(array=w1149) -> (reversed array=w1152:cluster{dbl, "GUIdevice 8":string}[])
              }
              frame True {
                w1157 = cluster{dbl, "GUIdevice 8":string}[] [] ("Array")
                n630 = for {
                  shift-right: [w1169] -> w1158
                  shift-left: w1157 -> [w1171]
                  tunnel: w1159 -> [w1170] mode=indexing
                  n631 = Unbundle(w1170) -> (w1173:dbl)  [unwired: 1 out]
                  n632 = Not Equal To 0?(x=w1173) -> (x != 0?=w1172:bool)
                  n633 = case shown="True" w1172 {
                    tunnel: w1171 -> [w1174 w1177]
                    tunnel: w1170 -> [_ w1176]
                    tunnel: [w1174 w1175] -> w1169
                    frame False {
                    }
                    frame True {
                      n634 = Build Array (concatenate)(w1177, w1176) -> (w1175:cluster{dbl, "GUIdevice 8":string}[])
                    }
                  }
                }
                n635 = for {
                  shift-right: [w1160] -> w1155
                  shift-left: w1157 -> [w1162]
                  tunnel: w1156 -> [w1161] mode=indexing
                  n636 = Unbundle(w1161) -> (w1164:dbl)  [unwired: 1 out]
                  n637 = Not Equal To 0?(x=w1164) -> (x != 0?=w1163:bool)
                  n638 = case shown="True" w1163 {
                    tunnel: w1162 -> [w1165 w1168]
                    tunnel: w1161 -> [_ w1167]
                    tunnel: [w1165 w1166] -> w1160
                    frame False {
                    }
                    frame True {
                      n639 = Build Array (concatenate)(w1168, w1167) -> (w1166:cluster{dbl, "GUIdevice 8":string}[])
                    }
                  }
                }
              }
            }
            n640 = call <vilib>:"Add State(s) to Queue__jki_lib_state_machine.vi"("State(s) in (\"\")"=w1123) -> ("States Out"=w1122:string)  [unwired: 14 in]
            n641 = Bundle By Name(cluster=w1117, "speedmode X"=w1118, "speedmode Y"=w1114) -> (w1116:T36)
            n642 = Empty Array?(array=w1136) -> (empty?=w1133:bool)
            n643 = Empty Array?(array=w1130) -> (empty?=w1128:bool)
            n644 = Index Array(array=w1136) -> (element=w1126:cluster{dbl, "GUIdevice 8":string})  [unwired: 1 in]
            n645 = Index Array(array=w1130) -> (element=w1125:cluster{dbl, "GUIdevice 8":string})  [unwired: 1 in]
            n646 = Unbundle(w1126) -> (w1135:dbl)  [unwired: 1 out]
            n647 = Unbundle(w1125) -> (w1131:dbl)  [unwired: 1 out]
            n648 = Equal To 0?(x=w1135) -> (x = 0?=w1134:bool)
            n649 = Equal To 0?(x=w1131) -> (x = 0?=w1129:bool)
            n650 = property on="autodetect" class="Bool (strict)"("Value"=FALSE ("autodetect")) -> ()  [unwired: 2 in, 2 out]
            n651 = Unbundle By Name(w1116) -> ("Feedback global"=w1137:bool)
            n652 = Or(x=w1134, y=w1133) -> (x .or. y?=w1132:bool)
            n653 = Or(x=w1129, y=w1128) -> (x .or. y?=w1127:bool)
            n654 = case shown="True" w1137 {
              tunnel: w1132 -> [_ w1185]
              tunnel: w1136 -> [_ w1184]
              tunnel: w1127 -> [_ w1182]
              tunnel: w1130 -> [_ w1181]
              tunnel: w1122 -> [w1178 w1180]
              tunnel: [w1178 w1179] -> w1138
              frame False {
              }
              frame True {
                n655 = case shown="False" w1185 {
                  tunnel: w1184 -> [w1200 _]
                  tunnel: w1180 -> [w1196 w1201]
                  tunnel: [w1194 w1201] -> w1183
                  frame False {
                    n656 = Index Array(array=w1200) -> (element=w1199:cluster{dbl, "GUIdevice 8":string})  [unwired: 1 in]
                    n657 = Unbundle By Name(w1199) -> ("GUIdevice 8"=w1198:string)
                    n658 = call <vilib>:"Build State String with Arguments__jki_lib_state_machine.vi"("Arguments (\"\")"=w1198, "State"="Move X") -> ("State with Arguments"=w1195:string)  [unwired: 4 in]
                    n659 = call <vilib>:"Add State(s) to Queue__jki_lib_state_machine.vi"("State(s) in (\"\")"=w1196, "State(s) at Back (\"\")"=w1195) -> ("States Out"=w1194:string)  [unwired: 13 in]
                  }
                  frame True {
                  }
                }
                n660 = case shown="False" w1182 {
                  tunnel: w1181 -> [w1192 _]
                  tunnel: w1183 -> [w1188 w1193]
                  tunnel: [w1186 w1193] -> w1179
                  frame False {
                    n661 = Index Array(array=w1192) -> (element=w1191:cluster{dbl, "GUIdevice 8":string})  [unwired: 1 in]
                    n662 = Unbundle By Name(w1191) -> ("GUIdevice 8"=w1190:string)
                    n663 = call <vilib>:"Build State String with Arguments__jki_lib_state_machine.vi"("Arguments (\"\")"=w1190, "State"="Move Y") -> ("State with Arguments"=w1187:string)  [unwired: 4 in]
                    n664 = call <vilib>:"Add State(s) to Queue__jki_lib_state_machine.vi"("State(s) in (\"\")"=w1188, "State(s) at Back (\"\")"=w1187) -> ("States Out"=w1186:string)  [unwired: 13 in]
                  }
                  frame True {
                  }
                }
              }
            }
            n665 = call <vilib>:"Add State(s) to Queue__jki_lib_state_machine.vi"("State(s) in (\"\")"=w1122, "State(s) at Back (\"\")"=w1138) -> ("States Out"=w1148:string)  [unwired: 13 in]
          }
          frame "Move X" {
            # "Your code here.\n(You can make a copy of, or modify, this frame)"
            n666 = Unbundle By Name(w1270) -> ("Offset X"=w1247:dbl[][])
            n667 = call-poly <userlib>:"Filter 1D Array__ogtk.vi"("items to filter"=w1255, "array"=w1274) -> ("filtered item indices"=w1259:i32[])  [unwired: 4 in, 1 out]
            n668 = Unbundle By Name(w1270) -> ("speedmode X"=w1254:bool[], "active axis refs 2"=w1273:T12, "move properties"=w1258:T2[])
            n669 = for {
              tunnel: w1259 -> [w1279] mode=indexing
              tunnel: w1258 -> [w1283]
              shift-right: [w1278] -> w1256
              shift-left: i32[] [] ("filtered item indices") -> [w1281]
              n670 = Index Array(array=w1283, index=w1279) -> (element=w1282:T2)
              n671 = Unbundle By Name(w1282) -> ("enable feedback"=w1280:bool)
              n672 = case shown="True" w1280 {
                tunnel: w1281 -> [w1284 w1287]
                tunnel: w1279 -> [_ w1286]
                tunnel: [w1284 w1285] -> w1278
                frame False {
                }
                frame True {
                  n673 = Build Array (concatenate)(w1287, w1286) -> (w1285:i32[])
                }
              }
            }
            n674 = Index Array(array=w1256) -> (element=w1253:i32)  [unwired: 1 in]
            n675 = Index Array(array=w1247, index (row)=w1253) -> (element=w1269:dbl[])  [unwired: 1 in]
            n676 = Reverse 1D Array(array=w1269) -> (reversed array=w1268:dbl[])
            n677 = Index Array(array=w1273, index=w1253) -> (element=w1272:cluster{"Ref X":refnum<vi>, "Ref Y":refnum<vi>})
            n678 = Index Array(array=w1268) -> (element=w1266:dbl)  [unwired: 1 in]
            n679 = Index Array(array=w1258, index=w1253) -> (element=w1271:T2)
            n680 = Unbundle By Name(w1272) -> ("Ref X"=w1263:refnum<vi>, "Ref Y"=w1262:refnum<vi>)
            n681 = Index Array(array=w1254, index=w1253) -> (element=w1252:bool)
            n682 = Unbundle By Name(w1271) -> ("Invert Direction X"=w1264:bool, "Invert Axis"=w1267:bool, "Stepsize"=w1250:dbl, "enable feedback"=w1261:bool)
            n683 = Greater Or Equal To 0?(x=w1266) -> (x >= 0?=w1265:bool)
            n684 = call <vilib>:"Add State(s) to Queue__jki_lib_state_machine.vi"("State(s) in Front (\"\")"="Wait" ("State(s) in Front (\"\")"), "State(s) in (\"\")"=w1277) -> ("States Out"=w1276:string)  [unwired: 13 in]
            n685 = property on="Speedmode @" class="DigNum (strict)"() -> ("Value"=w1249:dbl)  [unwired: 2 in, 2 out]
            n686 = Multiply(x=w1249, y=w1250) -> (x*y=w1251:dbl)
            n687 = Select(t=w1251, s=w1252, f=w1250) -> (s? t:f=w1248:dbl)
            n688 = case shown="True" w1261 {
              tunnel: w1267 -> [_ w1293]
              tunnel: w1265 -> [_ w1292]
              tunnel: w1248 -> [_ w1291]
              tunnel: w1264 -> [_ w1290]
              tunnel: w1263 -> [_ w1289]
              tunnel: w1262 -> [_ w1288]
              frame False {
              }
              frame True {
                n689 = case shown="False" w1292 {
                  tunnel: w1290 -> [w1301 w1323]
                  tunnel: w1291 -> [w1299 w1321]
                  tunnel: w1293 -> [w1298 w1320]
                  tunnel: w1293 -> [w1297 w1319]
                  tunnel: w1289 -> [w1295 w1317]
                  tunnel: w1288 -> [w1294 w1316]
                  frame True {
                    n690 = case shown="False" w1298 {
                      tunnel: [w1312 w1314] -> w1300
                      tunnel: w1295 -> [w1313 _]
                      tunnel: w1294 -> [_ w1315]
                      frame False {
                        n691 = property class="DigNum (strict)"(reference=w1313) -> ("Value"=w1312:dbl)  [unwired: 1 in, 2 out]
                      }
                      frame True {
                        n692 = property class="DigNum (strict)"(reference=w1315) -> ("Value"=w1314:dbl)  [unwired: 1 in, 2 out]
                      }
                    }
                    n693 = case shown="False" w1301 {
                      tunnel: w1300 -> [w1308 w1311]
                      tunnel: w1299 -> [w1307 w1310]
                      tunnel: [w1306 w1309] -> w1296
                      frame False {
                        n694 = Add(x=w1308, y=w1307) -> (x+y=w1306:dbl)
                      }
                      frame True {
                        n695 = Subtract(x=w1311, y=w1310) -> (x-y=w1309:dbl)
                      }
                    }
                    n696 = case shown="False" w1297 {
                      tunnel: w1296 -> [w1302 w1304]
                      tunnel: w1295 -> [w1303 _]
                      tunnel: w1294 -> [_ w1305]
                      frame False {
                        n697 = property class="DigNum (strict)"(reference=w1303, "Val(Sgnl)"=w1302) -> ()  [unwired: 1 in, 2 out]
                      }
                      frame True {
                        n698 = property class="DigNum (strict)"(reference=w1305, "Val(Sgnl)"=w1304) -> ()  [unwired: 1 in, 2 out]
                      }
                    }
                  }
                  frame False {
                    n699 = case shown="False" w1320 {
                      tunnel: [w1334 w1336] -> w1322
                      tunnel: w1317 -> [w1335 _]
                      tunnel: w1316 -> [_ w1337]
                      frame False {
                        n700 = property class="DigNum (strict)"(reference=w1335) -> ("Value"=w1334:dbl)  [unwired: 1 in, 2 out]
                      }
                      frame True {
                        n701 = property class="DigNum (strict)"(reference=w1337) -> ("Value"=w1336:dbl)  [unwired: 1 in, 2 out]
                      }
                    }
                    n702 = case shown="False" w1323 {
                      tunnel: w1322 -> [w1330 w1333]
                      tunnel: w1321 -> [w1329 w1332]
                      tunnel: [w1328 w1331] -> w1318
                      frame False {
                        n703 = Subtract(x=w1330, y=w1329) -> (x-y=w1328:dbl)
                      }
                      frame True {
                        n704 = Add(x=w1333, y=w1332) -> (x+y=w1331:dbl)
                      }
                    }
                    n705 = case shown="False" w1319 {
                      tunnel: w1318 -> [w1324 w1326]
                      tunnel: w1317 -> [w1325 _]
                      tunnel: w1316 -> [_ w1327]
                      frame False {
                        n706 = property class="DigNum (strict)"(reference=w1325, "Val(Sgnl)"=w1324) -> ()  [unwired: 1 in, 2 out]
                      }
                      frame True {
                        n707 = property class="DigNum (strict)"(reference=w1327, "Val(Sgnl)"=w1326) -> ()  [unwired: 1 in, 2 out]
                      }
                    }
                  }
                }
              }
            }
            "Arguments X" <- w1255
            "Moving X" <- w1255
          }
          frame "Move Y" {
            # "Your code here.\n(You can make a copy of, or modify, this frame)"
            n708 = Unbundle By Name(w1361) -> ("Offset Y"=w1360:dbl[][])
            n709 = call-poly <userlib>:"Filter 1D Array__ogtk.vi"("items to filter"=w1345, "array"=w1365) -> ("filtered item indices"=w1350:i32[])  [unwired: 4 in, 1 out]
            n710 = Unbundle By Name(w1361) -> ("speedmode Y"=w1344:bool[], "active axis refs 2"=w1364:T12, "move properties"=w1348:T2[])
            n711 = for {
              tunnel: w1350 -> [w1370] mode=indexing
              tunnel: w1348 -> [w1374]
              shift-right: [w1369] -> w1349
              shift-left: i32[] [] ("filtered item indices") -> [w1372]
              n712 = Index Array(array=w1374, index=w1370) -> (element=w1373:T2)
              n713 = Unbundle By Name(w1373) -> ("enable feedback"=w1371:bool)
              n714 = case shown="True" w1371 {
                tunnel: w1372 -> [w1375 w1378]
                tunnel: w1370 -> [_ w1377]
                tunnel: [w1375 w1376] -> w1369
                frame False {
                }
                frame True {
                  n715 = Build Array (concatenate)(w1378, w1377) -> (w1376:i32[])
                }
              }
            }
            n716 = Index Array(array=w1349) -> (element=w1343:i32)  [unwired: 1 in]
            n717 = Index Array(array=w1360, index (row)=w1343) -> (element=w1359:dbl[])  [unwired: 1 in]
            n718 = Reverse 1D Array(array=w1359) -> (reversed array=w1358:dbl[])
            n719 = Index Array(array=w1364, index=w1343) -> (element=w1363:cluster{"Ref X":refnum<vi>, "Ref Y":refnum<vi>})
            n720 = Index Array(array=w1358) -> (element=w1356:dbl)  [unwired: 1 in]
            n721 = Index Array(array=w1348, index=w1343) -> (element=w1362:T2)
            n722 = Index Array(array=w1344, index=w1343) -> (element=w1342:bool)
            n723 = Unbundle By Name(w1363) -> ("Ref Y"=w1353:refnum<vi>, "Ref X"=w1352:refnum<vi>)
            n724 = Unbundle By Name(w1362) -> ("Invert Direction Y"=w1354:bool, "Invert Axis"=w1357:bool, "Stepsize"=w1340:dbl, "enable feedback"=w1351:bool)
            n725 = Greater Or Equal To 0?(x=w1356) -> (x >= 0?=w1355:bool)
            n726 = call <vilib>:"Add State(s) to Queue__jki_lib_state_machine.vi"("State(s) in Front (\"\")"="Wait" ("State(s) in Front (\"\")"), "State(s) in (\"\")"=w1368) -> ("States Out"=w1367:string)  [unwired: 13 in]
            n727 = property on="Speedmode @" class="DigNum (strict)"() -> ("Value"=w1339:dbl)  [unwired: 2 in, 2 out]
            n728 = Multiply(x=w1339, y=w1340) -> (x*y=w1338:dbl)
            n729 = Select(t=w1338, s=w1342, f=w1340) -> (s? t:f=w1341:dbl)
            n730 = case shown="True" w1351 {
              tunnel: w1357 -> [_ w1384]
              tunnel: w1355 -> [_ w1383]
              tunnel: w1341 -> [_ w1382]
              tunnel: w1354 -> [_ w1381]
              tunnel: w1353 -> [_ w1380]
              tunnel: w1352 -> [_ w1379]
              frame False {
              }
              frame True {
                n731 = case shown="True" w1383 {
                  tunnel: w1381 -> [w1392 w1414]
                  tunnel: w1382 -> [w1390 w1412]
                  tunnel: w1384 -> [w1389 w1411]
                  tunnel: w1384 -> [w1388 w1410]
                  tunnel: w1380 -> [w1386 w1408]
                  tunnel: w1379 -> [w1385 w1407]
                  frame True {
                    n732 = case shown="False" w1389 {
                      tunnel: [w1403 w1405] -> w1391
                      tunnel: w1386 -> [w1404 _]
                      tunnel: w1385 -> [_ w1406]
                      frame False {
                        n733 = property class="DigNum (strict)"(reference=w1404) -> ("Value"=w1403:dbl)  [unwired: 1 in, 2 out]
                      }
                      frame True {
                        n734 = property class="DigNum (strict)"(reference=w1406) -> ("Value"=w1405:dbl)  [unwired: 1 in, 2 out]
                      }
                    }
                    n735 = case shown="False" w1392 {
                      tunnel: w1391 -> [w1399 w1402]
                      tunnel: w1390 -> [w1398 w1401]
                      tunnel: [w1397 w1400] -> w1387
                      frame False {
                        n736 = Add(x=w1399, y=w1398) -> (x+y=w1397:dbl)
                      }
                      frame True {
                        n737 = Subtract(x=w1402, y=w1401) -> (x-y=w1400:dbl)
                      }
                    }
                    n738 = case shown="False" w1388 {
                      tunnel: w1387 -> [w1393 w1395]
                      tunnel: w1386 -> [w1394 _]
                      tunnel: w1385 -> [_ w1396]
                      frame False {
                        n739 = property class="DigNum (strict)"(reference=w1394, "Val(Sgnl)"=w1393) -> ()  [unwired: 1 in, 2 out]
                      }
                      frame True {
                        n740 = property class="DigNum (strict)"(reference=w1396, "Val(Sgnl)"=w1395) -> ()  [unwired: 1 in, 2 out]
                      }
                    }
                  }
                  frame False {
                    n741 = case shown="False" w1411 {
                      tunnel: [w1425 w1427] -> w1413
                      tunnel: w1408 -> [w1426 _]
                      tunnel: w1407 -> [_ w1428]
                      frame False {
                        n742 = property class="DigNum (strict)"(reference=w1426) -> ("Value"=w1425:dbl)  [unwired: 1 in, 2 out]
                      }
                      frame True {
                        n743 = property class="DigNum (strict)"(reference=w1428) -> ("Value"=w1427:dbl)  [unwired: 1 in, 2 out]
                      }
                    }
                    n744 = case shown="False" w1414 {
                      tunnel: w1413 -> [w1421 w1424]
                      tunnel: w1412 -> [w1420 w1423]
                      tunnel: [w1419 w1422] -> w1409
                      frame False {
                        n745 = Subtract(x=w1421, y=w1420) -> (x-y=w1419:dbl)
                      }
                      frame True {
                        n746 = Add(x=w1424, y=w1423) -> (x+y=w1422:dbl)
                      }
                    }
                    n747 = case shown="False" w1410 {
                      tunnel: w1409 -> [w1415 w1417]
                      tunnel: w1408 -> [w1416 _]
                      tunnel: w1407 -> [_ w1418]
                      frame False {
                        n748 = property class="DigNum (strict)"(reference=w1416, "Val(Sgnl)"=w1415) -> ()  [unwired: 1 in, 2 out]
                      }
                      frame True {
                        n749 = property class="DigNum (strict)"(reference=w1418, "Val(Sgnl)"=w1417) -> ()  [unwired: 1 in, 2 out]
                      }
                    }
                  }
                }
              }
            }
            "Arguments Y" <- w1345
            "Moving Y" <- w1345
          }
          frame "Wait" {
            # "Your code here.\n(You can make a copy of, or modify, this frame)"
            n750 = flat-sequence {
              frame #0 {
                n751 = Wait (ms)(milliseconds to wait=u32 300) -> ()  [unwired: 1 out]
              }
              frame #1 {
                n752 = property on="Moving Y" class="Str"("Value"="") -> ()  [unwired: 2 in, 2 out]
                n753 = property on="Moving X" class="Str"("Value"="") -> ()  [unwired: 2 in, 2 out]
              }
            }
            n754 = call <vilib>:"Add State(s) to Queue__jki_lib_state_machine.vi"("State(s) in (\"\")"=w1434) -> ("States Out"=w1433:string)  [unwired: 14 in]
            n755 = local read "Mean Centroid X"() -> (w1429:dbl[][])
            n756 = Bundle By Name(cluster=w1431, "Mean Centroid X"=w1429, "Mean Centroid Y"=w1429) -> (w1430:T36)
          }
          frame "stats" {
            # "Your code here.\n(You can make a copy of, or modify, this frame)"
            n757 = Unbundle By Name(w1443) -> ("Offset X"=w1442:dbl[][], "Offset Y"=w1441:dbl[][], "Time"=w1440:timestamp[][], "Motor X"=w1439:dbl[][], "Motor Y"=w1438:dbl[][])
            n758 = for {
              tunnel: w1441 -> [w1481]
              tunnel: w1440 -> [w1482]
              tunnel: w1442 -> [w1483]
              tunnel: [w1486] -> w1469 mode=indexing
              tunnel: w1439 -> [w1480]
              tunnel: w1438 -> [w1479]
              tunnel: w1444 -> [_] mode=indexing
              i -> [w1473]
              n759 = Index Array(array=w1481, index (row)=w1473) -> (element=w1477:dbl[])  [unwired: 1 in]
              n760 = Index Array(array=w1480, index (row)=w1473) -> (element=w1475:dbl[])  [unwired: 1 in]
              n761 = Index Array(array=w1479, index (row)=w1473) -> (element=w1474:dbl[])  [unwired: 1 in]
              n762 = Index Array(array=w1483, index (row)=w1473) -> (element=w1478:dbl[])  [unwired: 1 in]
              n763 = Index Array(array=w1482, index (row)=w1473) -> (element=w1476:timestamp[])  [unwired: 1 in]
              n764 = Bundle("Time"=w1476, "Motor X"=w1475) -> (w1485:cluster{"Time":timestamp[], "Motor X":dbl[]})  [unwired: 1 in]
              n765 = Bundle("Time"=w1476, "Motor Y"=w1474) -> (w1484:cluster{"Time":timestamp[], "Motor Y":dbl[]})  [unwired: 1 in]
              n766 = Bundle("Time"=w1476, "Offset X"=w1478) -> (w1487:cluster{"Time":timestamp[], "Offset X":dbl[]})  [unwired: 1 in]
              n767 = Bundle("Time"=w1476, "Offset Y"=w1477) -> (w1488:cluster{"Time":timestamp[], "Offset Y":dbl[]})  [unwired: 1 in]
              n768 = Build Array(w1488, w1487, w1485, w1484) -> (w1486:cluster{"Time":timestamp[], "Motor Y":dbl[]}[])
            }
            n769 = call <vilib>:"Add State(s) to Queue__jki_lib_state_machine.vi"("State(s) in (\"\")"=w1472) -> ("States Out"=w1471:string)  [unwired: 14 in]
            n770 = Index Array(array=w1469, index (row) #1=0 ("index (row)"), index (row) #2=1 ("index (row)"), index (row) #3=2 ("index (row)"), index (row) #4=3 ("index (row)"), index (row) #5=4 ("index (row)"), index (row) #6=5 ("index (row)"), index (row) #7=6 ("index (row)"), index (row) #8=7 ("index (row)"), index (row) #9=8 ("index (row)"), index (row) #10=9 ("index (row)"), index (row) #11=10 ("index (row)"), index (row) #12=11 ("index (row)")) -> (element #1=→"CCD 1":cluster{"Time":timestamp[], "Motor Y":dbl[]}[], element #2=→"CCD 2":cluster{"Time":timestamp[], "Motor Y":dbl[]}[], element #3=→"CCD 3":cluster{"Time":timestamp[], "Motor Y":dbl[]}[], element #4=→"CCD 4":cluster{"Time":timestamp[], "Motor Y":dbl[]}[], element #5=→"CCD 5":cluster{"Time":timestamp[], "Motor Y":dbl[]}[], element #6=→"CCD 6":cluster{"Time":timestamp[], "Motor Y":dbl[]}[], element #7=→"CCD 7":cluster{"Time":timestamp[], "Motor Y":dbl[]}[], element #8=→"CCD 8":cluster{"Time":timestamp[], "Motor Y":dbl[]}[], element #9=→"CCD 9":cluster{"Time":timestamp[], "Motor Y":dbl[]}[], element #10=→"CCD 10":cluster{"Time":timestamp[], "Motor Y":dbl[]}[], element #11=→"CCD 11":cluster{"Time":timestamp[], "Motor Y":dbl[]}[], element #12=→"CCD 12":cluster{"Time":timestamp[], "Motor Y":dbl[]}[])  [unwired: 12 in]
          }
          frame "---------------Statistics--------------" {
            # "Template Separator\n(You can make a copy of, or modify, this frame)"
            n771 = call <vilib>:"Add State(s) to Queue__jki_lib_state_machine.vi"("State(s) in (\"\")"=w1492) -> ("States Out"=w1491:string)  [unwired: 14 in]
          }
          frame "Save Stats" {
            # "Your code here.\n(You can make a copy of, or modify, this frame)"
            n772 = property on="CCD 1" class="XYGraph (strict)"() -> ("Value"=w1502:cluster{timestamp[], dbl[]}[])  [unwired: 2 in, 2 out]
            n773 = property on="CCD 2" class="XYGraph (strict)"() -> ("Value"=w1501:cluster{timestamp[], dbl[]}[])  [unwired: 2 in, 2 out]
            n774 = property on="CCD 3" class="XYGraph (strict)"() -> ("Value"=w1500:cluster{timestamp[], dbl[]}[])  [unwired: 2 in, 2 out]
            n775 = property on="CCD 4" class="XYGraph (strict)"() -> ("Value"=w1499:cluster{timestamp[], dbl[]}[])  [unwired: 2 in, 2 out]
            n776 = property on="CCD 5" class="XYGraph (strict)"() -> ("Value"=w1498:cluster{timestamp[], dbl[]}[])  [unwired: 2 in, 2 out]
            n777 = property on="CCD 6" class="XYGraph (strict)"() -> ("Value"=w1497:cluster{timestamp[], dbl[]}[])  [unwired: 2 in, 2 out]
            n778 = property on="CCD 7" class="XYGraph (strict)"() -> ("Value"=w1496:cluster{timestamp[], dbl[]}[])  [unwired: 2 in, 2 out]
            n779 = property on="CCD 8" class="XYGraph (strict)"() -> ("Value"=w1495:cluster{timestamp[], dbl[]}[])  [unwired: 2 in, 2 out]
            n780 = Build Array(w1502, w1501, w1500, w1499, w1498, w1497, w1496, w1495) -> (w1494:cluster{timestamp[], dbl[]}[][])
            n781 = for {
              tunnel: w1494 -> [w1510] mode=indexing
              tunnel: w1493 -> [w1509] mode=indexing
              n782 = Empty String/Path?(string/path=w1509) -> (empty?=w1508:bool)
              n783 = case shown="False" w1508 {
                tunnel: w1510 -> [w1516 _]
                tunnel: w1509 -> [w1514 _]
                frame False {
                  n784 = Index Array(array=w1516, index #1=0 ("index"), index #2=1 ("index"), index #3=2 ("index"), index #4=3 ("index")) -> (element #1=w1551:cluster{timestamp[], dbl[]}, element #2=w1545:cluster{timestamp[], dbl[]}, element #3=w1544:cluster{timestamp[], dbl[]}, element #4=w1543:cluster{timestamp[], dbl[]})  [unwired: 1 in, 1 out]
                  n785 = Concatenate Strings(w1514, ".dat" ("string")) -> (w1512:string)
                  n786 = Unbundle(w1551) -> (w1550:timestamp[], w1528:dbl[])
                  n787 = Unbundle(w1545) -> (w1519:dbl[])  [unwired: 1 out]
                  n788 = Unbundle(w1544) -> (w1518:dbl[])  [unwired: 1 out]
                  n789 = Unbundle(w1543) -> (w1517:dbl[])  [unwired: 1 out]
                  n790 = Build Path(base path="save path", name or relative path=w1512) -> (appended path=w1511:path)
                  n791 = for {
                    tunnel: w1550 -> [w1553] mode=indexing
                    tunnel: [w1552] -> w1526 mode=indexing
                    n792 = Format Date/Time String(time format string (%c)="%Y%m%d%H%M%S", seconds (now)=w1553) -> (date/time string=w1552:string)  [unwired: 1 in]
                  }
                  n793 = Array Size(array=w1528) -> (size(s)=w1529:i32)
                  n794 = Number To Fractional String(number=w1528) -> (F-format string=w1525:string[])  [unwired: 3 in]
                  n795 = Number To Fractional String(number=w1519) -> (F-format string=w1522:string[])  [unwired: 3 in]
                  n796 = Number To Fractional String(number=w1518) -> (F-format string=w1521:string[])  [unwired: 3 in]
                  n797 = Number To Fractional String(number=w1517) -> (F-format string=w1520:string[])  [unwired: 3 in]
                  n798 = Initialize Array("", w1529, 5 ("dimension size")) -> (w1527:string[][])
                  n799 = Insert Into Array(array=w1527, index (col)=0 ("disabled index (col)"), new element=w1526) -> (w1537:string[][])  [unwired: 1 in]
                  n800 = Insert Into Array(array=w1537, index (col)=1 ("disabled index (col)"), new element=w1525) -> (w1536:string[][])  [unwired: 1 in]
                  n801 = Insert Into Array(array=w1536, index (col)=2 ("disabled index (col)"), new element=w1522) -> (w1540:string[][])  [unwired: 1 in]
                  n802 = Insert Into Array(array=w1540, index (col)=3 ("disabled index (col)"), new element=w1521) -> (w1541:string[][])  [unwired: 1 in]
                  n803 = Insert Into Array(array=w1541, index (col)=4 ("disabled index (col)"), new element=w1520) -> (w1542:string[][])  [unwired: 1 in]
                  n804 = Insert Into Array(array=w1542, index (row)=0, new element=string[] ["time", "Centroid X", "Centroid Y", "Motor Axis 1", "Motor Axis 2"] ("new element/subarray 2")) -> (w1524:string[][])  [unwired: 1 in]
                  n805 = call-poly <vilib>:"Write To Spreadsheet File.vi"("2D data"=w1524, "file path (dialog if empty)"=w1511) -> ()  [unwired: 6 in, 1 out]
                }
                frame True {
                }
              }
            }
            n806 = call <vilib>:"Add State(s) to Queue__jki_lib_state_machine.vi"("State(s) in (\"\")"=w1507) -> ("States Out"=w1506:string)  [unwired: 14 in]
            n807 = property on="Save Stats" class="Bool (strict)"("Value"=FALSE ("Save Stats")) -> ()  [unwired: 2 in, 2 out]
          }
          frame "tdms" {
            w1578 = 21600.0 ("new tdms")
            # "Your code here.\n(You can make a copy of, or modify, this frame)"
            n808 = Unbundle By Name(w1567) -> ("Data Value Reference out"=w1592:refnum<k34>, "Offset X"=w1594:dbl[][], "Offset Y"=w1589:dbl[][], "active axis refs 2"=w1591:T12)
            n809 = for {
              tunnel: w1594 -> [w1638]
              tunnel: w1589 -> [w1637]
              tunnel: w1593 -> [w1601] mode=indexing
              tunnel: w1592 -> [w1602]
              tunnel: w1591 -> [w1623]
              tunnel: w1590 -> [w1607]
              tunnel: [w1605] -> w1588
              i -> [w1624]
              n810 = Index Array(array=w1638, index (row)=w1624) -> (element=w1636:dbl[])  [unwired: 1 in]
              n811 = Index Array(array=w1637, index (row)=w1624) -> (element=w1635:dbl[])  [unwired: 1 in]
              n812 = Index Array(array=w1623, index=w1624) -> (element=w1622:cluster{"Ref X":refnum<vi>, "Ref Y":refnum<vi>})
              n813 = Reverse 1D Array(array=w1635) -> (reversed array=w1633:dbl[])
              n814 = Reverse 1D Array(array=w1636) -> (reversed array=w1634:dbl[])
              n815 = Unbundle By Name(w1622) -> ("Ref X"=w1621:refnum<vi>, "Ref Y"=w1620:refnum<vi>)
              n816 = Index Array(array=w1634) -> (element=w1632:dbl)  [unwired: 1 in]
              n817 = Index Array(array=w1633) -> (element=w1631:dbl)  [unwired: 1 in]
              n818 = property class="DigNum (strict)"(reference=w1621, error in=w1607) -> (error out=w1606:errorcluster, "Value"=w1615:dbl)  [unwired: 1 out]
              n819 = Build Array(w1632) -> (w1604:dbl[])
              n820 = Build Array(w1631) -> (w1626:dbl[])
              n821 = Get Date/Time In Seconds() -> (seconds since 1Jan1904=w1603:timestamp)
              n822 = Build Array(w1603) -> (w1599:timestamp[])
              n823 = property class="DigNum (strict)"(reference=w1620, error in=w1606) -> (error out=w1597:errorcluster, "Value"=w1609:dbl)  [unwired: 1 out]
              n824 = Build Array(w1615) -> (w1614:dbl[])
              n825 = TDMS Write(0:w1602, 5:w1601, 7:"time", 9:w1599, 11:w1597) -> (4:w1598:refnum<k34>, 15:w1596:errorcluster)  [unwired: 1 in, 2 out]
              n826 = Build Array(w1609) -> (w1608:dbl[])
              n827 = TDMS Write(0:w1598, 5:w1601, 7:"centroid X", 9:w1604, 11:w1596) -> (4:w1629:refnum<k34>, 6:w1628:string, 15:w1627:errorcluster)  [unwired: 1 in, 1 out]
              n828 = TDMS Write(0:w1629, 5:w1628, 7:"centroid Y", 9:w1626, 11:w1627) -> (4:w1618:refnum<k34>, 6:w1617:string, 15:w1619:errorcluster)  [unwired: 1 in, 1 out]
              n829 = TDMS Write(0:w1618, 5:w1617, 7:"Motor Axis 1", 9:w1614, 11:w1619) -> (4:w1613:refnum<k34>, 6:w1612:string, 15:w1610:errorcluster)  [unwired: 1 in, 1 out]
              n830 = TDMS Write(0:w1613, 5:w1612, 7:"Motor Axis 2", 9:w1608, 11:w1610) -> (15:w1605:errorcluster)  [unwired: 1 in, 3 out]
            }
            n831 = Unbundle By Name(w1567) -> ("img to avg"=w1565:i32)
            n832 = property on="millisecond timer value" class="DigNum (strict)"() -> ("Value"=w1568:u32)  [unwired: 2 in, 2 out]
            n833 = local read "millisecond timer 2"() -> (w1584:u32)
            n834 = Tick Count (ms)() -> (millisecond timer value=w1569:u32)
            n835 = call <userlib>:"Tick Count (ms)__ogtk.vi"("error in (no error)"=w1588) -> ("error out"=w1585:errorcluster, "millisecond timer value"=w1587:u32)  [unwired: 9 in]
            n836 = Subtract(x=w1569, y=w1568) -> (x-y=w1583:u32)
            n837 = Subtract(x=w1569, y=w1568) -> (x-y=w1570:u32)
            n838 = Subtract(x=w1587, y=w1584) -> (x-y=→"Waveform Chart":u32)
            n839 = Multiply(x=5.0 ("new tdms"), y=w1565) -> (x*y=w1563:dbl)
            n840 = Divide(x=w1583, y=u32 1000) -> (x/y=w1581:dbl)
            n841 = Divide(x=w1570, y=u32 1000) -> (x/y=w1572:dbl)
            n842 = Quotient & Remainder(x=w1581, y=w1578) -> (x-y*floor(x/y)=w1580:dbl)  [unwired: 1 out]
            n843 = Quotient & Remainder(x=w1572, y=w1563) -> (x-y*floor(x/y)=w1564:dbl)  [unwired: 1 out]
            "x-y*floor(x/y)" <- w1564
            n844 = Subtract(x=w1563, y=2.0) -> (x-y=w1561:dbl)
            n845 = Greater?(x=w1564, y=w1561) -> (0:w1560:bool)
            n846 = Subtract(x=w1578, y=20.0) -> (x-y=w1576:dbl)
            n847 = Greater?(x=w1580, y=w1576) -> (0:w1579:bool)
            n848 = Select(t="Device Ini", s=w1560, f="") -> (s? t:f=w1557:string)
            n849 = Select(t="newtdms", s=w1579, f="") -> (s? t:f=w1573:string)
            n850 = call <vilib>:"Add State(s) to Queue__jki_lib_state_machine.vi"("State(s) in (\"\")"=w1595, "State(s) at Back (\"\")"=w1573) -> ("States Out"=w1556:string)  [unwired: 13 in]
            n851 = call <vilib>:"Add State(s) to Queue__jki_lib_state_machine.vi"("State(s) in Front (\"\")"=w1557, "State(s) in (\"\")"=w1556) -> ("States Out"=w1555:string)  [unwired: 13 in]
          }
          frame "Reset History" {
            # "Your code here.\n(You can make a copy of, or modify, this frame)"
            n852 = for {
              N: 1 -> [_]
              shift-right: [w1648] -> w1640
              shift-left: timestamp[][] [] ("Time") -> [w1650]
              n853 = for {
                N: 12 -> [_]
                tunnel: w1650 -> [w1653] mode=indexing
                tunnel: [w1651] -> w1648 mode=indexing
                n854 = Get Date/Time In Seconds() -> (seconds since 1Jan1904=w1652:timestamp)
                n855 = Build Array (concatenate)(w1653, w1652) -> (w1651:timestamp[])
              }
            }
            n856 = local read "Offset X"() -> (w1639:dbl[][])
            n857 = Bundle By Name(cluster=w1644, "Offset X"=w1639, "Offset Y"=w1639, "Time"=w1640, "Motor X"=w1639) -> (w1643:T36)
            n858 = call <vilib>:"Add State(s) to Queue__jki_lib_state_machine.vi"("State(s) in (\"\")"=w1647) -> ("States Out"=w1646:string)  [unwired: 14 in]
          }
          frame "New Category: 2" {
            # "Your code here.\n(You can make a copy of, or modify, this frame)"
            n859 = call <vilib>:"Add State(s) to Queue__jki_lib_state_machine.vi"("State(s) in (\"\")"=w1657) -> ("States Out"=w1656:string)  [unwired: 14 in]
          }
          frame "ImgToAvg" {
            # "Your code here.\n(You can make a copy of, or modify, this frame)"
            n860 = Decimal String To Number(string=w1661) -> (number=w1658:i32)  [unwired: 2 in, 1 out]
            n861 = Bundle By Name(cluster=w1660, "img to avg"=w1658) -> (w1659:T36)
            n862 = call <vilib>:"Add State(s) to Queue__jki_lib_state_machine.vi"("State(s) in (\"\")"=w1664) -> ("States Out"=w1663:string)  [unwired: 14 in]
          }
          frame "newtdms" {
            # "Your code here.\n(You can make a copy of, or modify, this frame)"
            n863 = Unbundle By Name(w1673) -> ("Data Value Reference out"=w1672:refnum<k34>)
            n864 = TDMS Close(8:w1671, 11:w1672) -> (0:w1670:errorcluster)  [unwired: 1 out]
            n865 = Get Date/Time In Seconds() -> (seconds since 1Jan1904=w1684:timestamp)
            n866 = Format Date/Time String(time format string (%c)="%Y%m%d%H%M", seconds (now)=w1684) -> (date/time string=w1675:string)  [unwired: 1 in]
            n867 = Concatenate Strings(w1675, "Beampointing_Pico.tdms" ("string")) -> (w1681:string)
            n868 = String To Path(string=w1681) -> (path=w1682:path)
            n869 = Build Path(base path=path "w:/BP_upstairs", name or relative path=w1682) -> (appended path=w1676:path)
            n870 = TDMS Open(6:FALSE ("disable buffering (T)"), 7:enum16{"1.0", "2.0"}."2.0" ("file format version (2.0)"), 8:w1670, 10:T17."create or replace" ("operation"), 11:w1676) -> (0:w1666:errorcluster, 3:w1669:refnum<k34>)  [unwired: 1 in]
            n871 = call "TDMSbuffersize.vi"("error in (no error)"=w1666, "group names"=w1668, "Data Value Reference in"=w1669) -> ("error out"=w1665:errorcluster, "Data Value Reference out"=w1667:refnum<k34>)  [unwired: 7 in]
            n872 = call <vilib>:"Add State(s) to Queue__jki_lib_state_machine.vi"("State(s) in (\"\")"=w1687) -> ("States Out"=w1686:string)  [unwired: 14 in]
            n873 = Bundle By Name(cluster=w1673, "Data Value Reference out"=w1667) -> (w1674:T36)
          }
          frame "Center" {
            # "Your code here.\n(You can make a copy of, or modify, this frame)"
            n874 = property on="Center" class="Bool (strict)"("Value"=FALSE ("Center")) -> ()  [unwired: 2 in, 2 out]
            n875 = control-ref of="image::1"() -> (w1702:refnum<vi>)
            n876 = control-ref of="image::2"() -> (w1701:refnum<vi>)
            n877 = control-ref of="image::3"() -> (w1700:refnum<vi>)
            n878 = control-ref of="image::4"() -> (w1699:refnum<vi>)
            n879 = control-ref of="image::5"() -> (w1698:refnum<vi>)
            n880 = control-ref of="image::6"() -> (w1697:refnum<vi>)
            n881 = control-ref of="image::7"() -> (w1696:refnum<vi>)
            n882 = control-ref of="image::8"() -> (w1695:refnum<vi>)
            n883 = control-ref of="image::9"() -> (w1694:refnum<vi>)
            n884 = control-ref of="image::10"() -> (w1693:refnum<vi>)
            n885 = control-ref of="image::11"() -> (w1692:refnum<vi>)
            n886 = control-ref of="image::12"() -> (w1691:refnum<vi>)
            n887 = for {
              tunnel: w1688 -> [w1715] mode=indexing
              tunnel: [w1710] -> w1703 mode=indexing
              n888 = Unbundle By Name(w1715) -> ("Target.X::12"=w1714:refnum<vi>, "Target.Y::12"=w1713:refnum<vi>)
              n889 = property class="DigNum (strict)"(reference=w1714) -> ("Value"=w1712:dbl)  [unwired: 1 in, 2 out]
              n890 = property class="DigNum (strict)"(reference=w1713) -> ("Value"=w1711:dbl)  [unwired: 1 in, 2 out]
              n891 = Bundle("Value"=w1712, "Value"=w1711) -> (w1710:cluster{"Value":dbl, "Value":dbl})  [unwired: 1 in]
            }
            n892 = call <vilib>:"Add State(s) to Queue__jki_lib_state_machine.vi"("State(s) in (\"\")"=w1707) -> ("States Out"=w1706:string)  [unwired: 14 in]
            n893 = Build Array(w1702, w1701, w1700, w1699, w1698, w1697, w1696, w1695, w1694, w1693, w1692, w1691) -> (w1690:refnum<vi>[])
            n894 = for {
              tunnel: w1690 -> [w1709] mode=indexing
              tunnel: w1703 -> [w1708] mode=indexing
              n895 = property class="ImageControl"(reference=w1709, "Image Center Position"=w1708) -> ()  [unwired: 1 in, 2 out]
            }
          }
          frame "history" {
            # "Your code here.\n(You can make a copy of, or modify, this frame)"
            n896 = Unbundle By Name(w1725) -> ("Offset X"=w1731:dbl[][], "Offset Y"=w1730:dbl[][], "Mean Centroid X"=w1729:dbl[][], "Mean Centroid Y"=w1728:dbl[][], "Motor X"=w1727:dbl[][], "Motor Y"=w1726:dbl[][], "Time"=w1717:timestamp[][])
            n897 = for {
              tunnel: w1731 -> [w1749] mode=indexing
              tunnel: w1730 -> [w1747] mode=indexing
              tunnel: w1729 -> [w1746] mode=indexing
              tunnel: w1728 -> [w1745] mode=indexing
              tunnel: w1727 -> [w1744] mode=indexing
              tunnel: w1726 -> [w1743] mode=indexing
              tunnel: [w1748] -> w1723 mode=indexing
              tunnel: [w1742] -> w1722 mode=indexing
              tunnel: [w1738] -> w1721 mode=indexing
              tunnel: [w1741] -> w1720 mode=indexing
              tunnel: [w1740] -> w1719 mode=indexing
              tunnel: [w1739] -> w1718 mode=indexing
              tunnel: w1717 -> [w1737] mode=indexing
              tunnel: [w1735] -> w1716 mode=indexing
              w1736 = 0
              n898 = Delete From Array(array=w1744, index=w1736) -> (array with subset deleted=w1740:dbl[])  [unwired: 1 in, 1 out]
              n899 = Delete From Array(array=w1743, index=w1736) -> (array with subset deleted=w1739:dbl[])  [unwired: 1 in, 1 out]
              n900 = Delete From Array(array=w1737, index=w1736) -> (array with subset deleted=w1735:timestamp[])  [unwired: 1 in, 1 out]
              n901 = Delete From Array(array=w1746, index=w1736) -> (array with subset deleted=w1738:dbl[])  [unwired: 1 in, 1 out]
              n902 = Delete From Array(array=w1745, index=w1736) -> (array with subset deleted=w1741:dbl[])  [unwired: 1 in, 1 out]
              n903 = Delete From Array(array=w1747, index=w1736) -> (array with subset deleted=w1742:dbl[])  [unwired: 1 in, 1 out]
              n904 = Delete From Array(array=w1749, index=w1736) -> (array with subset deleted=w1748:dbl[])  [unwired: 1 in, 1 out]
            }
            n905 = call <vilib>:"Add State(s) to Queue__jki_lib_state_machine.vi"("State(s) in (\"\")"=w1734) -> ("States Out"=w1733:string)  [unwired: 14 in]
            n906 = Bundle By Name(cluster=w1725, "Offset X"=w1723, "Offset Y"=w1722, "Mean Centroid X"=w1721, "Mean Centroid Y"=w1720, "Motor X"=w1719, "Motor Y"=w1718, "Time"=w1716) -> (w1724:T36)
          }
        }
        n907 = property on="Box" class="Arr (strict)"() -> ("Value"=w260:T6)  [unwired: 2 in, 2 out]
        n908 = for {
          tunnel: w262 -> [w287]
          tunnel: w261 -> [w288]
          tunnel: w253 -> [w280] mode=indexing
          tunnel: w260 -> [w281] mode=indexing
          n909 = call-poly <userlib>:"Filter 1D Array__ogtk.vi"("items to filter"=w280, "array"=w288) -> ("filtered item indices"=w289:i32[])  [unwired: 4 in, 1 out]
          n910 = Index Array(array=w289) -> (element=w283:i32)  [unwired: 1 in]
          n911 = Index Array(array=w287, index=w283) -> (element=w286:T30)
          n912 = Unbundle By Name(w286) -> ("Target.X::12"=w291:refnum<vi>, "Target.Y::12"=w290:refnum<vi>)
          n913 = property class="DigNum (strict)"(reference=w291) -> ("Value"=w285:dbl)  [unwired: 1 in, 2 out]
          n914 = property class="DigNum (strict)"(reference=w290) -> ("Value"=w284:dbl)  [unwired: 1 in, 2 out]
          n915 = call "draw crosshair imaq.vi"("Color"=u32 16774656, "Target.Y"=w284, "size"=cluster{"xhair size":dbl, "xhair size 2":dbl} {"xhair size"=25.0, "xhair size 2"=25.0}, "Target.X"=w285, "Bounding Rectangle"=T15 {"Left"=0, "Top"=0, "Right"=0, "Bottom"=0}, "image in"=w280) -> ("error out"=→"error out":errorcluster, "image out"=w279:T9)  [unwired: 4 in]
          n916 = call "draw box imaq.vi"("Color"=u32 1244928, "Rectangle"=w281, "image in"=w279) -> ()  [unwired: 8 in, 1 out]
        }
        n917 = property on="ActiveMotor" class="Ring (strict)"() -> ("Strings []"=w255:string[])  [unwired: 2 in, 2 out]
        n918 = Index Array(array=w255, index="ActiveMotor") -> (element=w256:string)
        n919 = Not Equal?(x="ActiveMotorName::99", y=w256) -> (x != y?=w257:bool)
        n920 = case shown="True" w257 {
          tunnel: w255 -> [_ w276]
          tunnel: "ActiveMotorName::99" -> [_ w275]
          frame False {
          }
          frame True {
            n921 = Search 1D Array(1D array=w276, element=w275) -> (index of element=w274:i32)  [unwired: 1 in]
            n922 = property on="ActiveMotor" class="Ring (strict)"("Value"=w274) -> ()  [unwired: 2 in, 2 out]
          }
        }
      }
      n923 = control-ref of="This Application"() -> (w243:refnum<vi>)
      n924 = control-ref of="This VI"() -> (w247:refnum<vi>)
      n925 = Current VI's Menubar() -> (w246:refnum<k9>)
      n926 = call "GUI_Master_subvi_reentrant_queues.vi"("This Application"=w243, "error in (no error)"=w244, "tcp data event"=w242, "Caller menu reference"=w246, "Caller VI ref"=w247) -> ("error out"=→"error IO 2":errorcluster)  [unwired: 6 in]
      n927 = Unbundle By Name(w132) -> ("Data Value Reference out"=w131:refnum<k34>)
      n928 = for {
        tunnel: w161 -> [w251] mode=indexing
        tunnel: w160 -> [w250]
        tunnel: [w249] -> w130
        n929 = call "IMAQ Dispose"("Image"=w251, "error in (no error)"=w250) -> ("error out"=w249:errorcluster)  [unwired: 4 in]
      }
      n930 = TDMS Close(8:w130, 11:w131) -> (0:→"error out 2":errorcluster)  [unwired: 1 out]
    }
  }
